vi "HV monitor.vi"() -> ()   [LabVIEW 2018]
uses:
  subvis/location cluster.ctl
  channel_cluster.ctl
  subvis/tabs.ctl
  subvis/crate.ctl
  subvis/card.ctl
  subvis/Channel Properties.ctl
  subvis/Group Properties.ctl
  subvis/channel.ctl
  subvis/Event Sources.ctl
  <vilib>/addons/zeromq/socket_type.ctl
  subvis/logs.ctl
  <vilib>/Utility/error.llb/DialogType.ctl
  history_array_type.ctl
  <vilib>/Utility/miscctls.llb/LVMinMaxIncTypeDef.ctl
  Tom Shaw/Lecroy Control/HV Documentation and Software for Testing/SubVIs/General_lecroy_command.ctl
  subvis/set location.ctl
  <vilib>/addons/zeromq/poll_type.ctl
  CAEN globals.vi
  <vilib>/Instr/_visa.llb/VISA Configure Serial Port (Instr).vi
  <vilib>/Utility/file.llb/Write Delimited Spreadsheet (string).vi
  subvis/bool to string small.vi
  <vilib>/Utility/file.llb/Read Delimited Spreadsheet (string).vi
  <vilib>/addons/zeromq/zmq_poll_scalar.vi
  <userlib>/_OpenG.lib/array/array.llb/Filter 1D Array with Scalar (I32)__ogtk.vi
  <userlib>/_OpenG.lib/array/array.llb/Delete Elements from 1D Array (I32)__ogtk.vi
  <userlib>/_OpenG.lib/array/array.llb/Remove Duplicates from 1D Array (I32)__ogtk.vi
  subvis/Timestamp String to LV Timestamp.vi
  subvis/buffer 2D array clust.vi
  subvis/buffer array clust.vi
  <vilib>/regexp/Match Regular Expression.xnode
  <vilib>/Utility/miscctls.llb/LVRowAndColumnTypeDef.ctl
  <vilib>/Utility/miscctls.llb/LVBoundsTypeDef.ctl
  <vilib>/addons/zeromq/zmq_context.lvclass
  <vilib>/addons/zeromq/zeromq.lvlib
  <vilib>/addons/zeromq/zmq_socket.lvclass
  <vilib>/platform/TimedLoop/XDataNode/XDataNode.xnode
  <vilib>/Platform/TimedLoop/XDataNode/nitl_modes.ctl
  <vilib>/Platform/TimedLoop/XDataNode/XDNodeRunTimeDep.lvlib
  <vilib>/Platform/TimedLoop/XDataNode/wakeup.ctl
  <vilib>/Platform/TimedLoop/XDataNode/timing_clust.ctl
panel:
  in  "Redundant bool":bool
  out "ZMQ_PMT_Err":string="\"%s\":\"%s\""
  out "slack":T1
  out "slack error":string
  in  "New Errors":string
  out "read error":cluster{"Crate":i32, "error out":errorcluster}
  in  "Reading LeCroy1 Page":bool
  in  "Reading LeCroy2 Page":bool
  in  "Update Plots & Alarms":T2
  in  "Do L2 Page Read":i32
  in  "Do L1 Page Read":i32
  in  "Read Crate Page":i32
  in  "Read Crate":i32
  in  "Do Caen Page Read":i32
  in  "Save PMT Voltage File":bool=TRUE
  out "Current ZMQ Log":path
  in  "Send ZMQ Reply":bool
  in  "Show hidden tabs":bool
  out "Status":string
  in  "get log file":bool=TRUE
  out "log file to get":string
  in  "Set Card.Channel":T3={" Card.Channel"=1.12, "Crate"=0} {"Card.Channel" format="%.2f"}
  in  "Handle ZMQ message":bool
  out "Selection Position":cluster{i32, i32}
  in  "Display String":string="Q"
  out "Time Element History.old":i32[][][](array[numeric])
  in  "Property":T4
  in  "Value":variant
  in  "Set channel property":bool
  out "bytes read Old":u32
  in  "Tab Control":T5
  in  "Shifter Notes":string
  out "Currents":cluster{dbl[], "TS History":dbl[]}[](graph)
  out "summary status":string
  out "Voltages":cluster{dbl[], "TS History":dbl[]}[](graph)
  in  "Clear Alarms":bool
  out "Read time (ms)":u32
  out "Key sent":string
  out "Screen Cluster":T6
  out "Display":string[][](table)
  out "lecroy2_hw_enable":bool
  out "lecroy1_hw_enable":bool
  out "caen_hw_enable":bool
  in  "Caen enable":bool
  in  "Lecroy 2 enable":bool
  in  "Lecroy 1 enable":bool
  in  "Show Group In Displayed Channels":bool
  in  "Add Group to Displayed Channels":bool
  in  "Restore PMT voltages":bool
  in  "Save PMT voltages":bool
  in  "Nominal PMT voltages":bool
  in  "Group":string(combo)="ACTIVE"
  in  "Set Group Property":bool
  in  "Value 2":dbl min=0.0 max=1.0 step=1.0 format="%1d"
  in  "Group Prop":T7 caption="Property"
  in  "Channel Array":T8[](array[typedef]) caption="Channel Name          ON    Status                                           Crate      Card      Chan       Vmon           Vset             Vfile               Imon            Imax              Timestamp                       Flag" {"Vfile (V)" format="%.1f V"; "Vswmax (V)" format="%#_g V"; "Iset (A)" format="%.2pA"; "Imon (A)" format="%.2pA"; "Vset (V)" format="%#_g V"; "Vmon (V)" format="%.1f V"}
  in  "Abort queued actions":bool
  in  "CAEN Vsel Buffer":bool=TRUE
  in  "re-read vfile voltages":bool
  in  "Channel Settings File":path=path "C:/Users/User/Documents/Logs/Channel_Settings.csv"
  in  "Ramp Voltages Slowly":bool
  in  "Start New Run":bool
  in  "Subrun":i32
  in  "Run":i32=1
  out "Current Channel Log":path
  out "Current Event Log":path
  in  "Start New Event Log":bool
  in  "Start New Channel Log":bool
  in  "Start New Error Log":bool
  in  "CAEN Serial Port":i32=6
  out "Current Error Log":path
  in  "Log Directory":path=path "C:/Users/User/Documents/Logs"
  in  "Log to File":bool=TRUE
  in  "Scan Rate (ms)":i32=1000
  in  "LeCroy 1 Serial Port":i32=5
  in  "LeCroy 2 Serial Port":i32=3
  in  "Slack port":u16=5995
  in  "CAEN Vsel Buffer Pin":u8=3 min=2 max=12 step=1
  in  "CAEN SW Enable Pin":u8=4 min=2 max=12 step=1
  in  "Arduino Serial Port":i32=9
  in  "ZMQ endpoint":string="tcp://*:5555"
  out "Crates":T9[](array[typedef]) caption="Crate Map"
  in  "Refresh Crate Map":bool
  out "Display array":string[][](array[string])
  in  "Crate":i32
  in  "Index":i32
  in  "Card":i32
  out "Current":T11(graph) caption="Current Graph"
  in  "History Length":i32=500
  out "Voltage":T11(graph) caption="Voltage Graph"
  in  "Channel":i32
  out "Error Timestamp":string
  out "Error Log":string[][](table)
  in  "Action log":string
  in  "error out":errorcluster
  out "Event Log":string[][](table)
  out "Alarm status":string
  in  "Send to Self":bool
  in  "Unsent Messages":string[](array[string])
  out "ZMQ Log":string[][](table)
  out "ZMQ message":string
  in  "ZMQ Reply":string[](array[string])
  out "Sending ZMQ":bool=TRUE
  in  "ZMQ Message":string[](array[string])=["{\"msg_id\":\"123\" , \"msg_type\":\"read\", \"msg_property\":\"vset\", \"2.4.2\":\"anything\"}", "{\"msg_id\":\"123\" , \"msg_type\":\"write\", \"msg_property\":\"vset\", \"2.4.2\":\"-1500\"}"]
  in  "Manual ZMQ Write":bool
  out "Screencap Timestamp":string
  out "Alarm Screencap":string
  out "Read buffer LeCroy 1":string
  out "Read buffer LeCroy 2":string
  out "Read buffer CAEN":string
  in  "Read":bool
  in  "'\\' codes display":bool
  in  "Line Wrapping":bool=TRUE
  in  "Write buffer":string caption="Write buffer ( '\\' code format)"
  in  "Write":bool
  in  "Reading page label":string="Reading page ..."
  in  "Config pg Crate":i32 caption="Crate" min=0 max=2 step=1
  in  "delay (ms)":u32=700 max=600000 step=1
  in  "stop":bool
  out "Reading page":bool
  in  "scan":bool=TRUE
  in  "Lock Page":bool
  in  "Kill All":bool
  out "Writing...":bool
  out "Reading...":bool
  in  "Timestamp":string
  in  "Status message":string
  out "hb":bool
  out "bytes read":cluster{dbl, "element":i32}(graph)
  # "N.B. demonstration messages: these are valid messages\nClear the array and write your own before sending!!!"
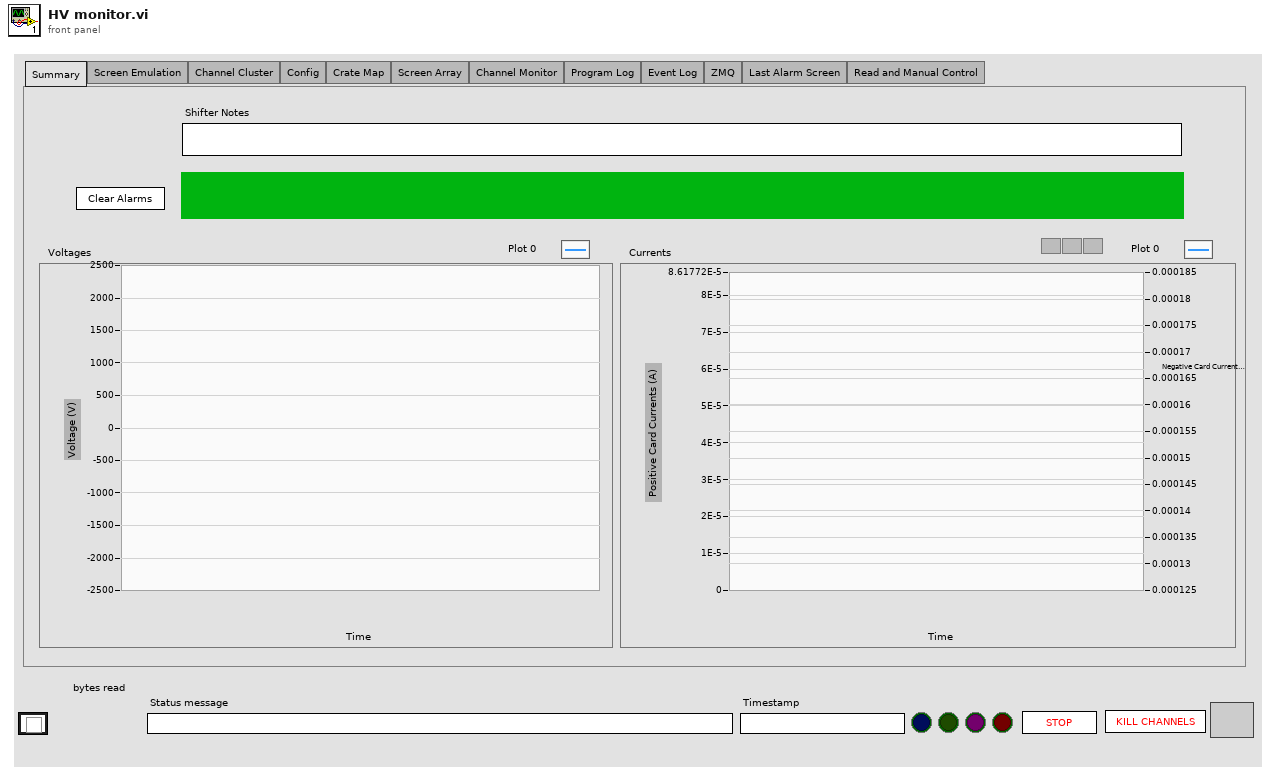
[diagram p1: front panel]
types:
  T1 = typedef "Semaphore RefNum" = refnum<k1>
  T2 = cluster{"Start Index":i32, "Num Channels Read":i32}
  T3 = typedef "channel.ctl" = cluster{" Card.Channel":dbl, "Crate":i32}
  T4 = typedef "Channel Properties.ctl" = enum16{"Name", "Vset", "Vfile", "Vswmax", "Iset", "Enable", "Flag", "Vbackup"}
  T5 = typedef "tabs.ctl" = enum32{"Summary", "Screen Emulation", "Channel Cluster", "Config", "Crate Map", "Screen Array", "Channel Monitor", "Program Log", "Event Log", "ZMQ", "Last Alarm Screen", "Read and Manual Control"}
  T6 = typedef "location cluster.ctl" = cluster{"Column":i32, "Card Type":string, "Channel":i32, "Card":i32, "Default response":string, "Entering":string, "Entering state":bool, "subpage":i32, "page":i32, "Crate":i32, "Screen":string, "Group":string, "Global HV Enable":bool, "Vsel_buffer":bool, "Vdisp_buffer":bool}
  T7 = typedef "Group Properties.ctl" = enum16{"Enable", "Vset", "Imax", "Vswmax", "Trip Time"}
  T8 = typedef "channel_cluster.ctl" = cluster{"Channel Name":string, "Crate":i32, "Card Type":string, "Card":i32, "Channel":i32, "Status Icon":picture, "Vmon (V)":dbl, "Vset (V)":dbl, "Imon (A)":dbl, "Iset (A)":dbl, "Timestamp":string, "ON/OFF":bool, "Status":string, "Vswmax (V)":dbl, "Flag":bool, "Vfile (V)":dbl, "Error Logged":bool[], "enable_file":bool}
  T9 = typedef "crate.ctl" = cluster{"CAENet Address":i32, "Crate Model":string, "Firmware Version":string, "Crate Map":T10[], "Total Channels":i32}
  T10 = typedef "card.ctl" = cluster{"Slot Number":i32, "Card Model":string, "Num Channels":i32, "Polarity":string, "Vmax":dbl, "Imax":dbl, "Revision":string}
  T11 = cluster{"Timestamp History":dbl[], "Vmon Hist":dbl[]}[]
  T12 = typedef "LVBoundsTypeDef.ctl" = cluster{"Width":u32, "Height":u32}
  T13 = typedef "LVRowAndColumnTypeDef.ctl" = cluster{"Row":i32, "Column":i32}
  T14 = cluster{"Channel Name":string, "Crate":i32, "Card Type":string, "Card":i32, "Channel":i32, "Status Icon":picture, "Vmon (V)":dbl, "Vset (V)":dbl, "Imon (mA)":dbl, "Iset (mA)":dbl, "Timestamp":string, "ON/OFF":bool, "Status":string}
  T15 = enum32{"Invalid", "Standard", "Closed", "Hidden", "Minimized", "Maximized"}
  T16 = typedef "Event Sources.ctl" = enum16{"ZMQ", "INTERNAL", "Check_Errors", "Send_ZMQ_Reply", "Save_PMT_Voltages", "Set_Ramp_Voltage", "Restore PMT Voltages"}
  T17 = typedef "zeromq.lvlib/socket_type.ctl" = enum8{"ZMQ_PAIR", "ZMQ_PUB", "ZMQ_SUB", "ZMQ_REQ", "ZMQ_REP", "ZMQ_DEALER", "ZMQ_ROUTER", "ZMQ_PULL", "ZMQ_PUSH", "ZMQ_XPUB", "ZMQ_XSUB"}
  T18 = cluster{"Group Name":string, "Channels in Group":T3[]}
  T19 = cluster{"Group Name":string, "Channels in Group":T3[]}[]
  T20 = typedef "logs.ctl" = enum16{"Event", "ZMQ", "Channel", "Program"}
  T21 = cluster{"seconds since 1Jan1904":timestamp, "element":cluster{"Source":T16, "Command":string}}[]
  T22 = typedef "LVMinMaxIncTypeDef.ctl" = cluster{"Minimum":dbl, "Maximum":dbl, "Increment":dbl}
  T23 = typedef "General_lecroy_command.ctl" = string
  T24 = typedef "set location.ctl" = cluster{"set index":i32, "set Screen":string, "set subpage":i32, "set column":i32, "Group":string, "Crate":i32}
  T25 = typedef "zeromq.lvlib/poll_type.ctl" = enum16{"None", "In", "Out", "In/Out"}
  T26 = cluster{"Group Value":timestamp, "element":cluster{"Source":T16, "Command":string}}
  T27 = cluster{"Group Value":timestamp, "element":cluster{"Source":T16, "Command":string}}[]
  T28 = typedef "eventvkey.ctl" = enum16{"ASCII", "Enter", "Return", "Shift", "Ctrl", "Alt", "Cmd", "Opt", "Caps", "NumLock", "Clear", "Break", "Up", "Down", "Left", "Right", "Insert", "Delete", "Home", "End", "PageUp", "PageDown", "Escape", "Help", "Pause", "ScrollLock", "F1", "F2", "F3", "F4", "F5", "F6", "F7", "F8", "F9", "F10", "F11", "F12", "F13", "F14", "F15", "F16", "F17", "F18", "F19", "F20", "F21", "F22", "F23", "F24", "Play", "VolumeUp", "VolumeDown", "Mute", "Two Byte Char"}
  T29 = cluster{"seconds since 1Jan1904":timestamp, "element":cluster{"Source":T16, "Command":string}}
  T30 = typedef "DialogType.ctl" = u16
  T31 = typedef "history_array_type.ctl" = enum16{"Vmon", "Vset", "Imon", "Iset", "TimeStamp"}
  T32 = typedef "XDNodeRunTimeDep.lvlib/timing_clust.ctl" = cluster{"Expected End [f-1]":u64, "Actual End [f-1]":u64, "Finished Late? [f-1]":bool, "Expected End [i-1]":u64, "Actual End [i-1]":u64, "Finished Late? [i-1]":bool, "Expected Start [i]":u64, "Actual Start [i]":u64, "Expected Start [f]":u64, "Actual Start [f]":u64, "Source Name":string, "Structure Name":string, "Period":i64, "Deadline":i64, "Offset":i64, "Start":i64, "Priority":i32, "Timeout":i32, "Mode":T33, "Wakeup Reason":T34, "Error":errorcluster, "Source Type":string, "Secondary Source Type":string, "Global End Time":u64, "Global Start Time":u64, "Frame Duration":u64, "Iteration Duration":u64, "Assigned CPU":i32, "I/O Scan Engine Mode":u32}
  T33 = typedef "XDNodeRunTimeDep.lvlib/nitl_modes.ctl" = enum32{"No Change", "Process missed periods, maintain original phase", "Discard missed periods, maintain original phase", "Process missed periods, ignore original phase", "Discard missed periods, ignore original phase"}
  T34 = typedef "XDNodeRunTimeDep.lvlib/wakeup.ctl" = enum32{"Normal", "Aborted", "Asynchronous wakeup", "Timing source error", "Timed loop error", "Timeout"}
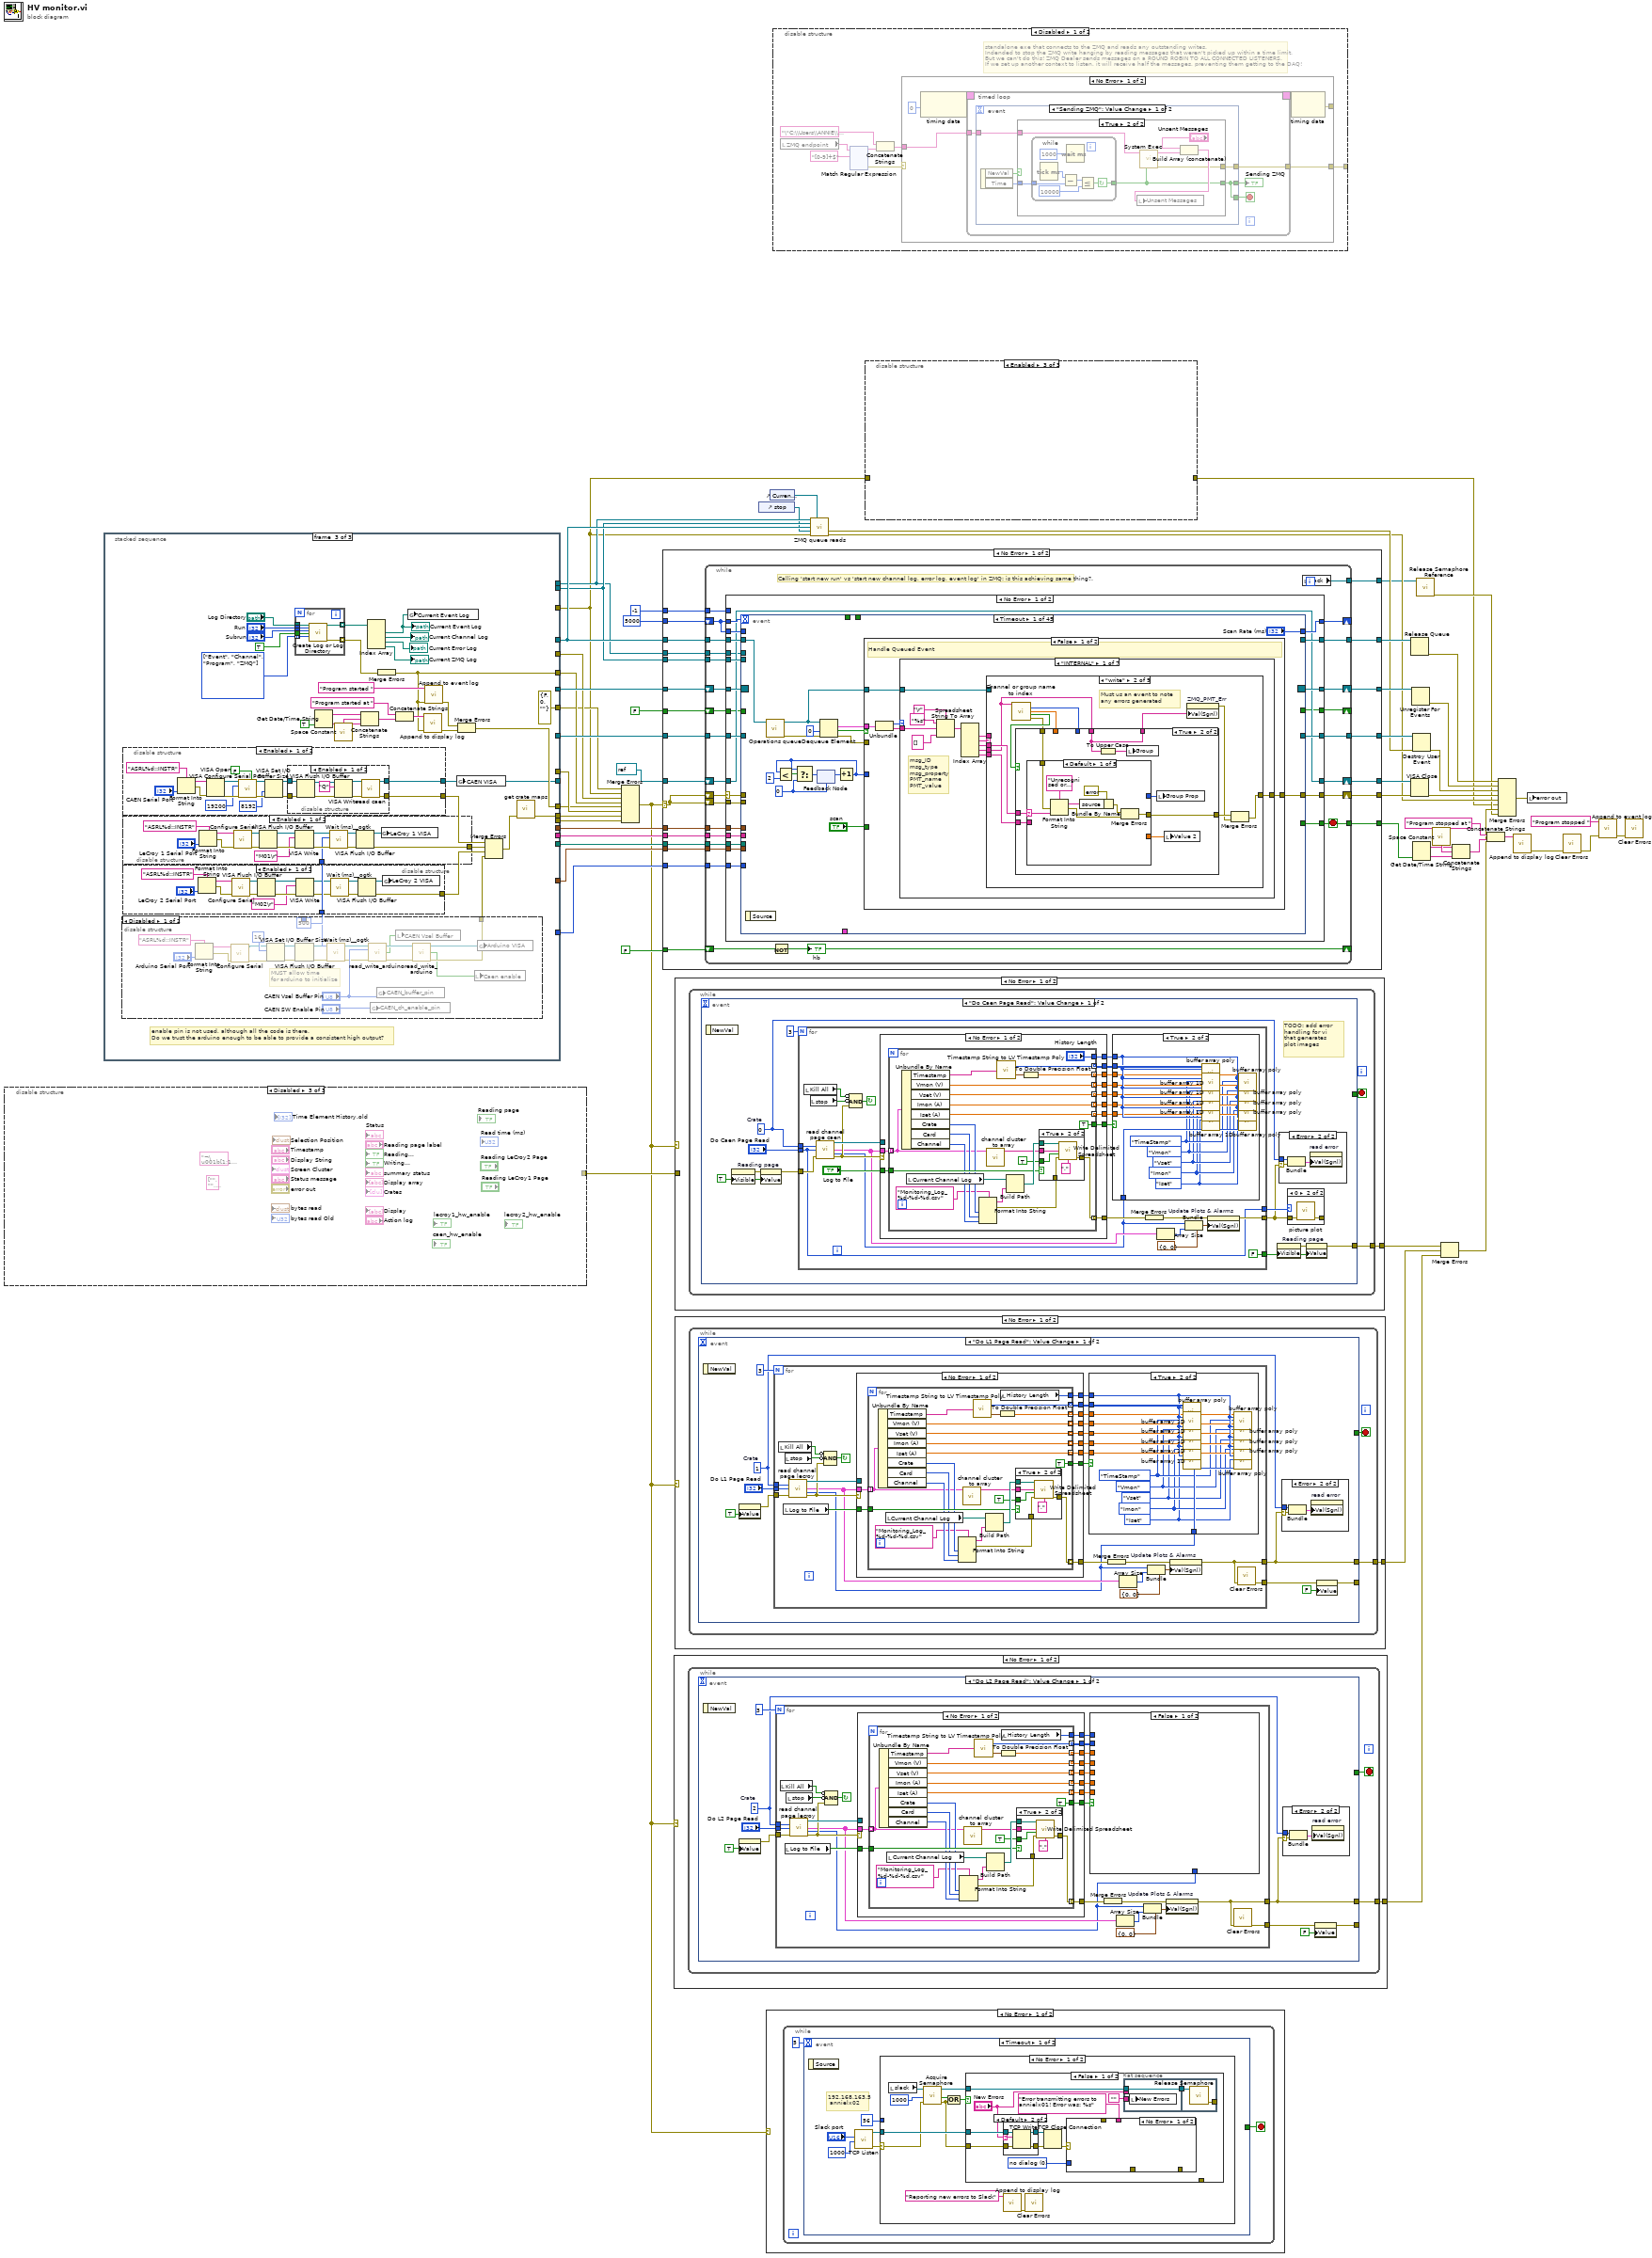
[diagram p0: block diagram]
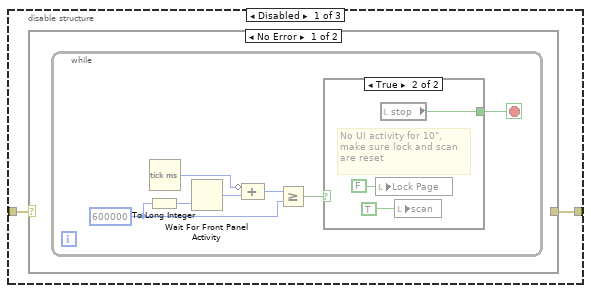
[diagram p2: hidden frame]
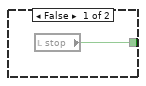
[diagram p3: hidden frame]
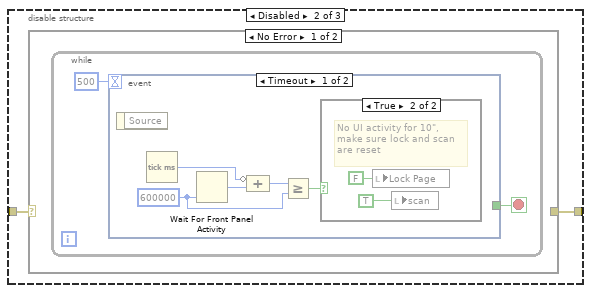
[diagram p5: hidden frame]
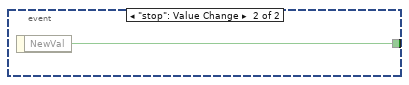
[diagram p7: hidden frame]
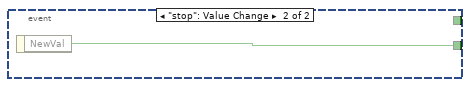
[diagram p10: hidden frame]
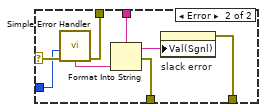
[diagram p13: hidden frame]
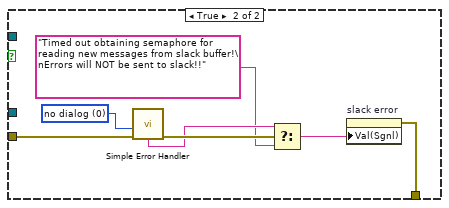
[diagram p15: hidden frame]
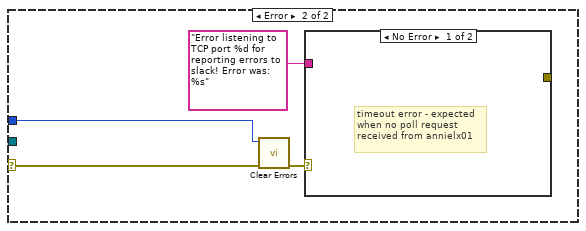
[diagram p16: hidden frame]
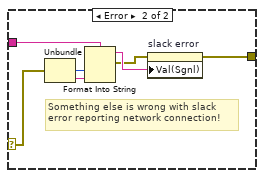
[diagram p17: hidden frame]
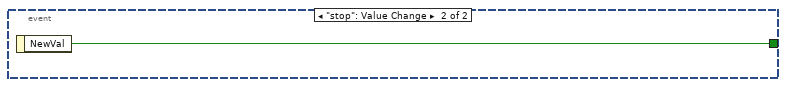
[diagram p18: hidden frame]
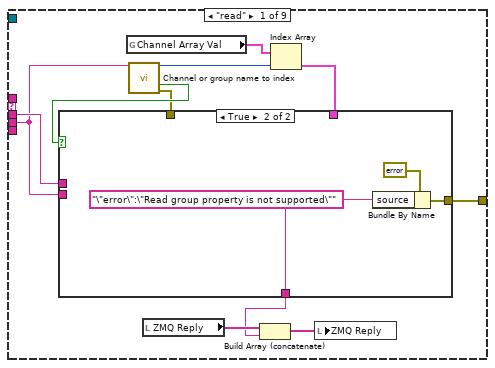
[diagram p20: hidden frame]
diagram:
  n1 = disable-structure shown="Disabled" {
    disable-tunnel: [w59 _ _] -> w11
    frame Disabled {
      w58 = 140 ("number")
      n2 = disable-structure shown="Disabled" {
        disable-tunnel: [w68 _] -> w65
        frame Disabled {
          n3 = property on="Display" class="Tbl (strict)"("Number of Columns"=u32 75, "Number of Rows"=u32 22 ("Number of Columns")) -> (error out=w68:errorcluster)  [unwired: 2 in, 1 out]
        }
        frame Enabled {
        }
      }
      n4 = property on="Display" class="Tbl (strict)" props=["Number of Columns", "Number of Rows"](error in=w65) -> ("Number of Rows"=w62:u32)  [unwired: 1 in, 3 out]
      n5 = To Long Integer(number=w62) -> (32bit integer=w63:i32)
      n6 = To Long Integer(number=w58) -> (32bit integer=w64:i32)
      n7 = disable-structure shown="Disabled" {
        disable-tunnel: w64 -> [w72 _]
        disable-tunnel: w63 -> [w71 _]
        disable-tunnel: [w70 w82] -> w61
        disable-tunnel: T12 {"Width"=13, "Height"=18} ("Active Cell:Cell Size") -> [w69 w82]
        frame Disabled {
          n8 = for {
            N: w72 -> [_]
            tunnel: w71 -> [w76]
            tunnel: [w74] -> w70
            tunnel: w69 -> [w73]
            i -> [w75]
            n9 = for {
              N: w76 -> [_]
              tunnel: w75 -> [w78]
              tunnel: [w77] -> w74
              tunnel: w73 -> [w77]
              i -> [w79]
              n10 = Bundle By Name(cluster=T13 {"Row"=0, "Column"=0} ("Active Cell:Active Cell"), "Row"=w79, "Column"=w78) -> (w80:T13)
              n11 = property on="Display" class="Tbl (strict)"("Active Cell"=w80, "Cell Size"=w77) -> ()  [unwired: 2 in, 2 out]
            }
          }
        }
        frame Enabled {
        }
      }
      n12 = for {
        N: w58 -> [_]
        tunnel: w61 -> [w84]
        tunnel: [w83] -> w59
        i -> [w86]
        n13 = Bundle By Name(cluster=T13 {"Row"=0, "Column"=0} ("Active Cell:Active Cell"), "Row"=0, "Column"=w86) -> (w87:T13)
        n14 = property on="Display" class="Tbl (strict)"("Active Cell"=w87, "Cell Size"=w84) -> (error out=w83:errorcluster)  [unwired: 2 in, 1 out]
      }
    }
    frame Enabled {
      (unwired) T14 {"Channel Name"="", "Crate"=0, "Card Type"="", "Card"=0, "Channel"=0, "Status Icon"=bytes[0], "Vmon (V)"=0.0, "Vset (V)"=0.0, "Imon (mA)"=0.0, "Iset (mA)"=0.0, "Timestamp"="", "ON/OFF"=FALSE, "Status"=""} ("Channel cluster")
      # "Channel, HVmax, Vmon, Imon, V*set, I*set, Pw, Status, Ch#\nChannel, SVmax, Rup, Rdwn, Trip, TripEx, PrOn, PrOff, Pon, Pdwn, Pswd, On/Off, Ch#"
      # "NEGAIVE: xxx.xxx mA only on chx.24\nreading also in mA\n\nPOSITIVE: xxxx.xx uA on all channels"
      # "0.* Channel name\n1.   Crate\n2.   Card Type\n3.   Card\n4.   Channel\n5.* Status Icon\n6.   Vmon\n7.* Vset\n8.   Imon\n9.* Iset\n10. Timestamp\n11.*On/Off"
      # "Display\nSet Protection (subpages todo)\nMain Menu\nLogo\nCrate Map\nKill Confirm\nConfigure Alarms\nFormat EEPROM\nUpgrade Firmware\nPage not recognised!"
    }
    frame Disabled {
      (unwired) "¬\u001b[1;1H¬\u001b[2J¬\u001b[4;10H¬\u001b[1mC.A.E.N.       SY527        V3.18¬\u001b[0m¬\u001b[4;62H¬\u001b[1mCrate 01¬\u001b[0m¬\u001b[9;7H¬\u001b[1mM A I N   M E N U¬\u001b[0m¬\u001b[11;1H      ¬\u001b[1mD¬\u001b[0misplay             Display/Modify channels\r\n      ¬\u001b[1mP¬\u001b[0mrotections         Set/Reset password\r\n      ¬\u001b[1mC¬\u001b[0mrate               Connect a new crate\r\n      ¬\u001b[1mM¬\u001b[0map                 Crate map\r\n      ¬\u001b[1mK¬\u001b[0mill                Kill all channels\r\n      ¬\u001b[1mA¬\u001b[0mlarms              Reset alarms\r\n      ¬\u001b[1mQ¬\u001b[0muit                Abandon program\r\n¬\u001b[0m¬\u001b[23;7HSelect item\r\n¬\u001b[23;1H¬\u001b[KEnter the crate number to be connected. [01]: " ("stripped output")
      (unwired) string[][] [["", "", "", "", "", "", "", "", "", "", "", "", ""], ["", "C.A.E.N.", "SY527", "V3.18", "A734 ", "", "", "", "", "", "", "", ""], ["", "GROUP00", "Ch_En is: On", "V0-SEL", "I0-SEL", "Crate 01", "Page 0 ", "", "", "", "", "", ""], ["", "", "", "", "", "", "", "", "", "", "", "", ""], ["Channel", "SVmax", "Rup", "Rdwn", "Trip", "TripEx", "PrOn", "PrOff", "Pon", "Pdwn", "Pswd", "On/Off", "Ch#"], ["KLn_1", "2200", "100", "100", "600.0", "--", "01", "01", "Off", "Kill", "Req", "En", "0.00"], ["KLn_2", "2200", "100", "100", "011.0", "--", "01", "01", "Off", "Kill", "", "", "0.01"], ["KLn_3", "2200", "100", "100", "010.0", "--", "01", "01", "Off", "Kill", "", "", "0.02"], ["KLn_4", "2200", "100", "100", "010.0", "--", "01", "01", "Off", "Kill", "", "", "0.03"], ["KLn_5", "2200", "100", "100", "010.0", "--", "01", "01", "Off", "Kill", "", "", "0.04"], ["KLn_6", "2200", "100", "100", "010.0", "--", "01", "01", "Off", "Kill", "", "", "0.05"], ["KLn_7", "2200", "100", "100", "010.0", "--", "01", "01", "Off", "Kill", "", "", "0.06"], ["KLn_8", "2200", "100", "100", "010.0", "--", "01", "01", "Off", "Kill", "", "", "0.07"], ["KLn_9", "2200", "100", "100", "010.0", "--", "01", "01", "Off", "Kill", "", "", "0.08"], ["KLn_10", "2200", "100", "100", "010.0", "--", "01", "01", "Off", "Kill", "", "", "0.09"], ["KLn_11", "2200", "100", "100", "010.0", "--", "01", "01", "Off", "Kill", "", "", "0.10"], ["KLn_12", "2200", "100", "100", "010.0", "--", "01", "01", "Off", "Kill", "", "", "0.11"], ["KLn_13", "2200", "100", "100", "010.0", "--", "01", "01", "Off", "Kill", "", "", "0.12"], ["KLn_14", "2200", "100", "100", "010.0", "--", "01", "01", "Off", "Kill", "", "", "0.13"], ["KLn_15", "2200", "100", "100", "110.0", "--", "01", "01", "Off", "Kill", "", "", "0.14"], ["KLn_16", "2200", "100", "100", "010.0", "--", "01", "01", "Off", "Kill", "", "", "0.15"], ["", "", "", "", "", "", "", "", "", "", "", "", ""], ["", "", "", "", "", "", "", "", "", "", "", "", ""], ["", "", "", "", "", "", "", "", "", "", "", "", ""], [" Quit Edit Change Update Next Prev More Switch", "", "", "", "", "", "", "", "", "", "", "", ""]] ("Display array 2")
    }
  }
  n15 = stacked-sequence {
    tunnel: [_ _ w191] -> w46
    tunnel: [_ w144 _] -> w49
    tunnel: [_ w170 _] -> w48
    tunnel: [_ w165 _] -> w47
    tunnel: [_ w169 _] -> w9
    tunnel: [_ w168 _] -> w19
    tunnel: [_ w167 _] -> w2
    tunnel: [_ _ w189] -> _
    tunnel: [w95 _ _] -> w17
    tunnel: [w93 _ _] -> w40
    tunnel: [_ _ w196] -> w39
    tunnel: [_ w161 _] -> w37
    tunnel: [_ w160 _] -> w38
    tunnel: [_ _ w197] -> w24
    tunnel: [w97 _ _] -> w23
    tunnel: [_ w151 _] -> w22
    tunnel: [_ w150 _] -> w21
    tunnel: [_ _ errorcluster {"status"=FALSE, "code"=0, "source"=""} ("error IO")] -> w20
    tunnel: [w109 _ _] -> w8
    frame #0 {
      w119 = "Everything is awesome" ("Alarm String")
      w120 = FALSE ("Append if exists?")
      # "This list MUST match the\ngroups defined on the CAEN\nand no additional groups\nshould be defined in the \nchannel settings file"
      # "num active\ncaen pages"
      n16 = invoke on="Action log" class="Str" method="Reinit To Default"() -> ()  [unwired: 3 in, 3 out]
      n17 = invoke on="Set Group Property" class="Bool (strict)" method="Reinit To Default"() -> ()  [unwired: 3 in, 3 out]
      n18 = invoke on="Channel Array" class="Arr (strict)" method="Reinit To Default"() -> ()  [unwired: 3 in, 3 out]
      n19 = invoke on="re-read vfile voltages" class="Bool" method="Reinit To Default"() -> ()  [unwired: 3 in, 3 out]
      n20 = invoke on="stop" class="Bool (strict)" method="Reinit To Default"() -> ()  [unwired: 3 in, 3 out]
      n21 = property on="summary status" class="Str"("Value"=w119, "Text.BGColor"=u32 46096, "Blinking"=w120) -> (error out=w118:errorcluster)  [unwired: 2 in, 1 out]
      n22 = invoke on="Writing..." class="Bool (strict)" method="Reinit To Default"() -> ()  [unwired: 3 in, 3 out]
      n23 = invoke on="New Errors" class="Str" method="Reinit To Default"() -> ()  [unwired: 3 in, 3 out]
      n24 = invoke on="Reading LeCroy1 Page" class="Bool (strict)" method="Reinit To Default"() -> ()  [unwired: 3 in, 3 out]
      n25 = invoke on="Reading LeCroy2 Page" class="Bool (strict)" method="Reinit To Default"() -> ()  [unwired: 3 in, 3 out]
      n26 = invoke on="Reading page" class="Bool (strict)" method="Reinit To Default"() -> ()  [unwired: 3 in, 3 out]
      n27 = call "load channel file.vi"("Group Names"=string[] ["GROUP00", "ACTIVE", "CARD0", "CARD1", "CARD2", "CARD3", "AGROUP", "CARD4", "MRD", "FACC", "TANK", "CAEN", "LeCroy1", "LeCroy2", "SPARE", "Broken"], "Channel List"="Channel Settings File") -> ("error out"=w98:errorcluster, "ACTIVE"=w106:T18, "GROUP00"=w108:T18, "Groups"=w100:T19)  [unwired: 5 in, 1 out]
      n28 = Read from Text File(file (use dialog)=path "C:/Users/User/Documents/Logs/Shifter_Notes.txt") -> (refnum out=w115:refnum<file>, text=w112:string, error out=w114:errorcluster)  [unwired: 3 in, 1 out]
      n29 = property on="Status message" class="Str"(error in=w118, "Value"=w119, "Blinking"=w120) -> ()  [unwired: 1 in, 2 out]
      n30 = Close File(refnum=w115, error in=w114) -> (error out=w113:errorcluster)  [unwired: 1 out]
      n31 = local write "Shifter Notes"(w112) -> ()
      n32 = for {
        tunnel: w100 -> [w131] mode=indexing
        tunnel: [w130] -> w99 mode=indexing
        n33 = Unbundle By Name(w131) -> ("Group Name"=w130:string)
      }
      n34 = global write "CAEN globals.vi" "Groups"(w100) -> ()
      n35 = Unbundle By Name(w106) -> ("Channels in Group"=w93:T3[])
      n36 = Unbundle By Name(w108) -> ("Channels in Group"=w95:T3[])
      n37 = call <vilib>:"Clear Errors.vi"("error in (no error)"=w113) -> ()  [unwired: 5 in, 2 out]
      n38 = property on="Group" class="CmbBox"(error in=w98, "Strings[]"=w99) -> (error out=w97:errorcluster)  [unwired: 1 in, 1 out]
      n39 = for {
        tunnel: w93 -> [w137] mode=indexing
        shift-right: [w134] -> w110
        shift-left: 0 ("Crate") -> [w132]
        n40 = Unbundle By Name(w137) -> ("Crate"=w136:i32)
        n41 = Increment(x=w132) -> (x+1=w133:i32)
        n42 = Not Equal To 0?(x=w136) -> (x != 0?=w135:bool)
        n43 = Select(t=w132, s=w135, f=w133) -> (s? t:f=w134:i32)
      }
      n44 = for {
        tunnel: w93 -> [w139] mode=indexing
        tunnel: w95 -> [w140]
        tunnel: [w138] -> w117 mode=indexing
        n45 = Search 1D Array(1D array=w140, element=w139) -> (index of element=w138:i32)  [unwired: 1 in]
      }
      n46 = control-ref of="CAEN Vsel Buffer"() -> (w89:refnum<vi>)
      n47 = control-ref of="Caen enable"() -> (w104:refnum<vi>)
      n48 = control-ref of="Lecroy 1 enable"() -> (w103:refnum<vi>)
      n49 = control-ref of="Lecroy 2 enable"() -> (w102:refnum<vi>)
      n50 = control-ref of="caen_hw_enable"() -> (w92:refnum<vi>)
      n51 = control-ref of="lecroy1_hw_enable"() -> (w91:refnum<vi>)
      n52 = control-ref of="lecroy2_hw_enable"() -> (w90:refnum<vi>)
      n53 = control-ref of="Writing..."() -> (w123:refnum<vi>)
      n54 = control-ref of="Reading..."() -> (w124:refnum<vi>)
      n55 = control-ref of="Screen Cluster"() -> (w101:refnum<vi>)
      n56 = control-ref of="This VI"() -> (w129:refnum<vi>)
      n57 = control-ref of="Display String"() -> (w126:refnum<vi>)
      n58 = control-ref of="Action log"() -> (w125:refnum<vi>)
      n59 = control-ref of="Channel Array"() -> (w96:refnum<vi>)
      n60 = control-ref of="Crates"() -> (w111:refnum<vi>)
      n61 = control-ref of="Display"() -> (w127:refnum<vi>)
      n62 = control-ref of="Display array"() -> (w128:refnum<vi>)
      n63 = control-ref of="Event Log"() -> (w122:refnum<vi>)
      n64 = global write "CAEN globals.vi" "Main VI"(w129) -> ()
      n65 = global write "CAEN globals.vi" "Channel Array"(w96) -> ()
      n66 = global write "CAEN globals.vi" "Crate Maps"(w111) -> ()
      n67 = global write "CAEN globals.vi" "Display"(w127) -> ()
      n68 = global write "CAEN globals.vi" "Display array"(w128) -> ()
      n69 = global write "CAEN globals.vi" "Location Cluster"(w101) -> ()
      n70 = global write "CAEN globals.vi" "Display string"(w126) -> ()
      n71 = global write "CAEN globals.vi" "Display Log"(w125) -> ()
      n72 = global write "CAEN globals.vi" "Event Log Indicator"(w122) -> ()
      n73 = global write "CAEN globals.vi" "Reading..."(w124) -> ()
      n74 = global write "CAEN globals.vi" "Writing..."(w123) -> ()
      n75 = global write "CAEN globals.vi" "CAEN HV enable"(w104) -> ()
      n76 = global write "CAEN globals.vi" "Lecroy 1 HV enable"(w103) -> ()
      n77 = global write "CAEN globals.vi" "Lecroy 2 HV enable"(w102) -> ()
      n78 = global write "CAEN globals.vi" "caen_hw_enable"(w92) -> ()
      n79 = global write "CAEN globals.vi" "lecroy1_hw_enable"(w91) -> ()
      n80 = global write "CAEN globals.vi" "lecroy2_hw_enable"(w90) -> ()
      n81 = global write "CAEN globals.vi" "CAEN Vsel Buffer"(w89) -> ()
      n82 = global write "CAEN globals.vi" "Visible Channels"(w117) -> ()
      n83 = global write "CAEN globals.vi" "Indices of ACTIVE"(w117) -> ()
      n84 = expression code="ceil(x/16)"(w110) -> (w109:i32)
    }
    frame #1 {
      w150 = "Run: %d Subrun: %d" ("ZMQ endpoint")
      n85 = control-ref of="This VI"() -> (w149:refnum<vi>)
      n86 = invoke class="VI" method="FP.Open"(reference=w149, "Activate"=TRUE ("Activate?"), "State"=T15."Standard") -> (error out=w143:errorcluster)  [unwired: 2 in, 4 out]
      n87 = disable-structure shown="Enabled" {
        disable-tunnel: [w180 _] -> w167
        disable-tunnel: [w177 _] -> w168
        disable-tunnel: [w182 _] -> w169
        frame Enabled {
          n88 = call <vilib>:"zmq_ctx_create.vi"() -> ("error out"=w185:errorcluster, "context out"=w186:refnum<class "zmq_context.lvclass">)  [unwired: 4 in]
          n89 = call <vilib>:"zmq_socket.vi"("error in"=w185, "linger (ms)"=100, "socket type"=socket_type."ZMQ_DEALER", "context in"=w186) -> ("error out"=w183:errorcluster, "socket out"=w178:refnum<class "zmq_socket.lvclass">, "context out"=w182:refnum<class "zmq_context.lvclass">)  [unwired: 1 in]
          n90 = call <vilib>:"zmq_bind.vi"("error in"=w183, "endpoint"="ZMQ endpoint", "socket in"=w178) -> ("error out"=w180:errorcluster, "socket out"=w177:refnum<class "zmq_socket.lvclass">)  [unwired: 1 in]
        }
        frame Disabled {
        }
      }
      n91 = Equal?(x=tabs."Screen Emulation" ("Tab Control"), y="Tab Control") -> (x = y?=w173:bool)
      n92 = control-ref of="This VI"() -> (w171:refnum<vi>)
      n93 = Select(t=w171, s=w173, f=refnum<vi> refnum ("vi reference")) -> (s? t:f=w175:refnum<vi>)
      n94 = Create User Event(user event datatype="" ("ZMQ endpoint")) -> (user event=w165:refnum<user-event>, error out=w176:errorcluster)  [unwired: 1 in]
      n95 = register-events(error in=w176, w175, w165) -> (reference out=w170:refnum<event-registration>, error out=w145:errorcluster)  [unwired: 1 in]
      n96 = Read from Text File(file (use dialog)=path "C:/Users/User/Documents/Logs/CurrentRun.txt" ("file path (dialog if empty)")) -> (refnum out=w154:refnum<file>, text=w157:string, error out=w153:errorcluster)  [unwired: 3 in, 1 out]
      n97 = call <vilib>:"Obtain Semaphore Reference.vi"() -> ("error out"=w141:errorcluster, "semaphore"=→"slack":T1)  [unwired: 5 in, 1 out]
      n98 = Close File(refnum=w154, error in=w153) -> (path=w151:path, error out=w152:errorcluster)
      n99 = Obtain Queue(element data type=cluster{"Source":T16, "Command":string} {"Source"=enum."ZMQ", "Command"=""} ("element")) -> (queue out=w163:refnum<queue>, error out=w162:errorcluster)  [unwired: 4 in, 1 out]
      n100 = Scan From String(format string=w150, input string=w157, error in=w152) -> (error out=w146:errorcluster, output 1=w156:i32, output 2=w155:i32)  [unwired: 3 in, 2 out]
      n101 = Flush Queue(queue=w163, error in (no error)=w162) -> (queue out=w161:refnum<queue>, error out=w160:errorcluster)  [unwired: 1 out]
      n102 = local write "Run"(w156) -> ()
      n103 = local write "Subrun"(w155) -> ()
      n104 = Merge Errors(w143, w145, w146, w141) -> (w144:errorcluster)
    }
    frame #2 {
      w199 = T20[] [enum."Event", enum."Channel", enum."Program", enum."ZMQ"] items=["Event", "ZMQ", "Channel", "Program"]
      # "enable pin is not used, although all the code is there.\nDo we trust the arduino enough to be able to provide a consistent high output?"
      n105 = disable-structure shown="Disabled" {
        disable-tunnel: [w229 _] -> w188
        disable-tunnel: [w221 _] -> w187
        frame Disabled {
          w229 = u32 500 ("milliseconds to wait")
          # "MUST allow time\nfor arduino to initialize"
          n106 = Format Into String(format string="ASRL%d::INSTR" ("write buffer"), "Arduino Serial Port") -> (resulting string=w233:string, error out=w234:errorcluster)  [unwired: 2 in]
          n107 = call "Configure Serial.vi"("error in"=w234, "Resource Name"=w233) -> ("error out"=w231:errorcluster, "VISA out"=w232:refnum<visa-resource-name>)  [unwired: 8 in]
          n108 = VISA Set I/O Buffer Size(VISA resource name=w232, mask (16)=u16 16 ("I/O Receive\nBuffer mask"), error in (no error)=w231) -> (VISA resource name out=w238:refnum<visa-resource-name>, error out=w237:errorcluster)  [unwired: 1 in]
          n109 = VISA Flush I/O Buffer(VISA resource name=w238, error in (no error)=w237) -> (VISA resource name out=w228:refnum<visa-resource-name>, error out=w230:errorcluster)  [unwired: 1 in]
          n110 = call <userlib>:"Wait (ms)__ogtk.vi"("error in (no error)"=w230, "milliseconds to wait"=w229) -> ("error out"=w225:errorcluster)  [unwired: 8 in, 1 out]
          n111 = call "read_write_arduino.vi"("VISA in"=w228, "Pin Num"="CAEN Vsel Buffer Pin", "error in"=w225) -> ("VISA out"=w223:refnum<visa-resource-name>, "State"=w219:bool, "error out"=w224:errorcluster)  [unwired: 9 in, 1 out]
          n112 = global write "CAEN globals.vi" "CAEN_ch_enable_pin"("CAEN SW Enable Pin") -> ()
          n113 = global write "CAEN globals.vi" "CAEN_buffer_pin"("CAEN Vsel Buffer Pin") -> ()
          n114 = local write "CAEN Vsel Buffer"(w219) -> ()
          n115 = call "read_write_arduino.vi"("VISA in"=w223, "error in"=w224) -> ("VISA out"=w222:refnum<visa-resource-name>, "State"=w220:bool, "error out"=w221:errorcluster)  [unwired: 10 in, 1 out]
          n116 = local write "Caen enable"(w220) -> ()
          n117 = global write "CAEN globals.vi" "Arduino VISA"(w222) -> ()
        }
        frame Enabled {
        }
      }
      n118 = disable-structure shown="Enabled" {
        disable-tunnel: [w283 _] -> w189
        disable-tunnel: [w282 _] -> w195
        frame Enabled {
          n119 = Format Into String(format string="ASRL%d::INSTR" ("write buffer"), "CAEN Serial Port") -> (resulting string=w284:string, error out=w287:errorcluster)  [unwired: 2 in]
          n120 = VISA Open(error in (no error)=w287, VISA resource name=w284) -> (VISA resource name=w291:refnum<visa-resource-name>, error out=w290:errorcluster)  [unwired: 3 in]
          n121 = call-poly "VISA Configure Serial Port"("VISA resource name"=w291, "Enable Termination\nChar (T)"=FALSE ("Enable Termination\nChar (T)"), "baud rate (9600)"=u32 19200, "error in (no error)"=w290) -> ("VISA resource name out"=w281:refnum<visa-resource-name>, "error out"=w280:errorcluster)  [unwired: 10 in]
          n122 = VISA Set I/O Buffer Size(VISA resource name=w281, size (4096)=u32 8192 ("baud rate (9600)"), error in (no error)=w280) -> (VISA resource name out=w279:refnum<visa-resource-name>, error out=w278:errorcluster)  [unwired: 1 in]
          n123 = disable-structure shown="Enabled" {
            disable-tunnel: [w293 w302] -> w283
            disable-tunnel: w278 -> [w297 w301]
            disable-tunnel: w279 -> [w296 w302]
            disable-tunnel: [w292 w301] -> w282
            frame Enabled {
              n124 = VISA Flush I/O Buffer(VISA resource name=w296, error in (no error)=w297) -> (VISA resource name out=w294:refnum<visa-resource-name>, error out=w295:errorcluster)  [unwired: 1 in]
              n125 = VISA Write(VISA resource name=w294, write buffer="Q", error in (no error)=w295) -> (VISA resource name out=w299:refnum<visa-resource-name>, error out=w298:errorcluster)  [unwired: 1 out]
              n126 = call "read caen.vi"("VISA in"=w299, "error in"=w298) -> ("VISA out"=w293:refnum<visa-resource-name>, "error out"=w292:errorcluster)  [unwired: 8 in, 4 out]
            }
            frame Disabled {
            }
          }
        }
        frame Disabled {
        }
      }
      n127 = disable-structure shown="Enabled" {
        disable-tunnel: [w259 _] -> w194
        disable-tunnel: w188 -> [w256 _]
        frame Enabled {
          n128 = Format Into String(format string="ASRL%d::INSTR" ("write buffer"), "LeCroy 1 Serial Port") -> (resulting string=w267:string, error out=w264:errorcluster)  [unwired: 2 in]
          n129 = call "Configure Serial.vi"("error in"=w264, "Resource Name"=w267) -> ("error out"=w265:errorcluster, "VISA out"=w266:refnum<visa-resource-name>)  [unwired: 8 in]
          n130 = VISA Flush I/O Buffer(VISA resource name=w266, error in (no error)=w265) -> (VISA resource name out=w262:refnum<visa-resource-name>, error out=w263:errorcluster)  [unwired: 1 in]
          n131 = VISA Write(VISA resource name=w262, write buffer="M01\r", error in (no error)=w263) -> (VISA resource name out=w261:refnum<visa-resource-name>, error out=w258:errorcluster)  [unwired: 1 out]
          n132 = call <userlib>:"Wait (ms)__ogtk.vi"("error in (no error)"=w258, "milliseconds to wait"=w256) -> ("error out"=w257:errorcluster)  [unwired: 8 in, 1 out]
          n133 = VISA Flush I/O Buffer(VISA resource name=w261, error in (no error)=w257) -> (VISA resource name out=w260:refnum<visa-resource-name>, error out=w259:errorcluster)  [unwired: 1 in]
          n134 = global write "CAEN globals.vi" "LeCroy 1 VISA"(w260) -> ()
        }
        frame Disabled {
        }
      }
      n135 = disable-structure shown="Enabled" {
        disable-tunnel: [w250 _] -> w193
        disable-tunnel: w188 -> [w240 _]
        frame Enabled {
          n136 = Format Into String(format string="ASRL%d::INSTR" ("write buffer"), "LeCroy 2 Serial Port") -> (resulting string=w253:string, error out=w254:errorcluster)  [unwired: 2 in]
          n137 = call "Configure Serial.vi"("error in"=w254, "Resource Name"=w253) -> ("error out"=w248:errorcluster, "VISA out"=w247:refnum<visa-resource-name>)  [unwired: 8 in]
          n138 = VISA Flush I/O Buffer(VISA resource name=w247, error in (no error)=w248) -> (VISA resource name out=w245:refnum<visa-resource-name>, error out=w244:errorcluster)  [unwired: 1 in]
          n139 = VISA Write(VISA resource name=w245, write buffer="M02\r", error in (no error)=w244) -> (VISA resource name out=w246:refnum<visa-resource-name>, error out=w242:errorcluster)  [unwired: 1 out]
          n140 = call <userlib>:"Wait (ms)__ogtk.vi"("error in (no error)"=w242, "milliseconds to wait"=w240) -> ("error out"=w241:errorcluster)  [unwired: 8 in, 1 out]
          n141 = VISA Flush I/O Buffer(VISA resource name=w246, error in (no error)=w241) -> (VISA resource name out=w249:refnum<visa-resource-name>, error out=w250:errorcluster)  [unwired: 1 in]
          n142 = global write "CAEN globals.vi" "LeCroy 2 VISA"(w249) -> ()
        }
        frame Disabled {
        }
      }
      n143 = for {
        tunnel: "Log Directory" -> [w276]
        tunnel: "Run" -> [w275]
        tunnel: "Subrun" -> [w274]
        tunnel: w199 -> [w273] mode=indexing
        tunnel: [w272] -> w206 mode=indexing
        tunnel: [w271] -> w198 mode=indexing
        tunnel: TRUE ("Append if exists?") -> [w270]
        n144 = call "Create Log or Log Directory.vi"("Base Directory"=w276, "Run"=w275, "Subrun"=w274, "Append if exists?"=w270, "Log Type"=w273) -> ("Path"=w272:path, "error out"=w271:errorcluster)  [unwired: 13 in]
      }
      n145 = Get Date/Time String(want seconds? (F)=TRUE) -> (date string=w218:string, time string=w217:string)  [unwired: 2 in]
      n146 = call <vilib>:"Space Constant.vi"() -> ("String"=w216:string)
      n147 = Concatenate Strings(w218, w216, w217) -> (w215:string)
      n148 = Index Array(array=w206) -> (element #1=w202:path, element #2=→"Current Channel Log":path, element #3=→"Current Error Log":path, element #4=→"Current ZMQ Log":path)  [unwired: 4 in]
      "Current Event Log" <- w202
      n149 = Merge Errors(w198) -> (w197:errorcluster)
      n150 = Concatenate Strings("Program started at " ("string"), w215) -> (w210:string)
      n151 = global write "CAEN globals.vi" "Current Event Log"(w202) -> ()
      n152 = call "Append to display log.vi"("error in"=w197, "string"=w210) -> ("error out"=w211:errorcluster)  [unwired: 9 in]
      n153 = call "Append to event log.vi"("error in"=w197, "string"="Program started ") -> ("error out"=w213:errorcluster)  [unwired: 9 in]
      n154 = global write "CAEN globals.vi" "CAEN VISA"(w189) -> ()
      n155 = Merge Errors(w213, w211) -> (w191:errorcluster)
      n156 = Merge Errors(w195, w194, w193, w187) -> (w192:errorcluster)
      n157 = call "get crate maps.vi"("error in"=w192) -> ("error out"=w196:errorcluster)  [unwired: 12 in, 2 out]
    }
  }
  n158 = Merge Errors(w20, w2, w38, w24, w46, w49, w39, w23) -> (w7:errorcluster)
  n159 = case shown="No Error" w7 {
    selector: w7 -> [w304 w2959]
    tunnel: FALSE ("READ") -> [w325 _]
    tunnel: 5000 -> [w324 _]
    tunnel: [w323 w2962] -> w55
    tunnel: w48 -> [w322 w2962]
    tunnel: w47 -> [w321 w2961]
    tunnel: w40 -> [w320 _]
    tunnel: w37 -> [w319 w2964]
    tunnel: [w318 w2964] -> w35
    tunnel: [w317 w2960] -> w33
    tunnel: [w316 w2959] -> w32
    tunnel: [w315 w2961] -> w29
    tunnel: -1 -> [w314 _]
    tunnel: w22 -> [w313 _]
    tunnel: w21 -> [w312 _]
    tunnel: w19 -> [w311 _]
    tunnel: [w310 TRUE ("stop")] -> w18
    tunnel: w17 -> [w309 _]
    tunnel: FALSE ("READ") -> [w308 _]
    tunnel: w8 -> [w307 _]
    tunnel: refnum<visa-resource-name> refnum ("VISA out") -> [w306 w2960]
    tunnel: w9 -> [w305 _]
    tunnel: [w303 w2957] -> w6
    frame No Error {
      n160 = while {
        shift-right: [w348] -> w316
        shift-left: w304 -> [w347]
        shift-right: [w349] -> _
        shift-left: w325 -> [w350]
        shift-right: [w346] -> _
        shift-left: w324 -> [w345]
        shift-right: [w343] -> w323
        shift-left: w322 -> [w344]
        tunnel: w311 -> [w340]
        tunnel: w321 -> [w342]
        tunnel: w309 -> [w341]
        tunnel: w320 -> [w339]
        tunnel: w307 -> [w338]
        tunnel: w319 -> [w337]
        tunnel: [w336] -> w315
        tunnel: [w335] -> w318
        shift-left: w304 -> [w334]
        tunnel: w314 -> [w333]
        tunnel: w313 -> [w332]
        tunnel: w312 -> [w331]
        shift-right: [w351] -> w317
        shift-left: w306 -> [w352]
        tunnel: [w330] -> w310
        shift-right: [w329] -> _
        shift-left: w308 -> [w328]
        tunnel: w305 -> [w327]
        tunnel: [w326] -> w303
        stop <- w330 stop-if-true
        # "Calling 'start new run' vs 'start new channel log, error log, event log' in ZMQ: is this achieving same thing?."
        n161 = case shown="No Error" w347 {
          selector: w347 -> [w374 w2731]
          tunnel: w352 -> [w356 w2729]
          tunnel: [w375 _] -> w330
          tunnel: [w356 w2730] -> w351
          tunnel: w345 -> [w359 w2733]
          tunnel: [w373 w2728] -> w348
          tunnel: [w372 w2733] -> w346
          tunnel: w345 -> [w371 _]
          tunnel: w344 -> [w370 w2732]
          tunnel: [w369 w2732] -> w343
          tunnel: w340 -> [w364 _]
          tunnel: w342 -> [w368 _]
          tunnel: w341 -> [w367 _]
          tunnel: w339 -> [w366 _]
          tunnel: w338 -> [w365 _]
          tunnel: w337 -> [w363 _]
          tunnel: [w362 _] -> w336
          tunnel: [w361 _] -> w335
          tunnel: w334 -> [w360 _]
          tunnel: w333 -> [_ _]
          tunnel: w332 -> [w358 _]
          tunnel: w331 -> [w357 _]
          tunnel: [w355 _] -> w329
          tunnel: w328 -> [w354 _]
          tunnel: w327 -> [w353 _]
          frame No Error {
            n162 = event shown="[0] Timeout" {
              selector: w370 -> [_ _ _ _ _ _ _ _ _ _ _ _ _ _ _ _ _ _ _ _ _ _ _ _ _ _ _ _ _ _ _ _ _ _ _ _ _ _ _ _ w2689 _ _ _ _]
              dyn-events: [_ _ _ _ _ _ _ _ _ _ _ _ _ _ _ _ _ _ _ _ _ _ _ _ _ _ _ _ _ _ _ _ _ _ _ _ _ _ _ _ w2693 _ _ _ _] -> w369
              timeout: w359 -> [_ _ _ w809 _ _ _ _ _ _ _ _ _ _ _ _ _ _ _ _ _ _ _ _ _ _ _ _ _ _ _ _ _ _ _ _ _ _ _ _ _ _ _ _ _]
              tunnel: w374 -> [_ _ _ _ _ _ _ _ _ _ _ _ _ _ _ _ _ _ _ _ _ _ _ _ _ _ _ _ _ _ _ _ _ _ _ _ _ _ _ _ _ _ _ _ _]
              tunnel: [_ _ _ _ _ _ _ _ _ _ _ _ _ _ _ _ _ _ _ _ _ _ _ _ _ _ _ _ _ _ _ _ _ _ _ _ _ _ _ _ _ _ _ _ "stop"] -> w375
              tunnel: [w387 w763 _ w811 _ w910 w993 w1063 w1142 w1166 w1259 w1342 w1382 w1435 w1465 w1487 w1497 w1509 w1523 w1580 w1703 w1724 w1767 w1840 w1869 w1882 w1896 w1916 w1927 w1939 w1967 w2007 w2066 w2088 w2132 w2338 _ w2405 w2597 w2635 w2696 w2706 w2713 w2721 w2725] -> w373
              tunnel: [_ _ "Ramp Voltages Slowly" _ "Redundant bool" "Read" "Write" _ _ _ _ _ _ _ "Start New Run" "Start New Error Log" "Start New Event Log" "Start New Channel Log" _ "Set channel property" _ "Set Group Property" "re-read vfile voltages" _ _ _ _ _ "Save PMT voltages" "Save PMT Voltage File" "Kill All" "Clear Alarms" "Refresh Crate Map" "get log file" "Handle ZMQ message" "Send ZMQ Reply" _ "Manual ZMQ Write" "Show Group In Displayed Channels" "Add Group to Displayed Channels" _ "Show hidden tabs" "'\\' codes display" "Line Wrapping" _] -> _
              tunnel: [_ _ _ _ _ _ _ _ _ _ _ _ _ _ _ _ _ _ "Channel Array" _ _ _ _ _ _ _ _ _ _ _ _ _ _ _ _ _ _ _ _ _ _ _ _ _ _] -> _
              tunnel: ["Scan Rate (ms)" w770 w799 w810 w863 w908 5000 w1065 w1141 w1176 w1263 w1343 w1383 w1441 w1464 w1492 w1505 w1518 w1521 w1581 w1705 w1725 w1763 w1836 w1863 w1876 w1890 w1914 w1932 w1945 5000 w2009 1000 w2102 w2140 w2360 50 ("Scan Rate (ms)") w2421 w2594 w2661 w2684 w2704 w2711 w2718 w2724] -> w372
              tunnel: w371 -> [_ w770 w799 _ w863 w908 _ w1065 w1141 w1176 w1263 w1343 w1383 w1441 w1464 w1492 w1505 w1518 w1521 w1581 w1705 w1725 w1763 w1836 w1863 w1876 w1890 w1914 w1932 w1945 _ w2009 _ w2102 w2140 w2360 _ w2421 w2594 w2661 w2684 w2704 w2711 w2718 w2724]
              tunnel: w364 -> [_ _ _ _ _ _ _ _ _ _ _ _ _ _ _ _ _ _ _ _ _ _ _ _ _ _ _ _ _ _ _ _ _ _ _ w2328 _ w2409 _ _ _ _ _ _ _]
              tunnel: w368 -> [_ _ _ _ _ _ _ _ _ _ _ _ _ _ _ _ _ _ _ _ _ _ _ _ _ _ _ _ _ _ _ _ _ _ _ _ _ _ _ _ w2686 _ _ _ w2723]
              tunnel: w367 -> [_ _ _ _ _ _ _ _ _ _ _ _ _ _ _ _ _ _ _ _ _ _ _ _ _ _ _ _ _ _ _ _ _ _ _ _ _ _ _ _ _ _ _ _ _]
              tunnel: w366 -> [_ _ _ _ _ _ _ _ _ w1153 _ _ _ w1436 _ _ _ _ _ _ _ _ _ _ _ _ _ _ _ _ _ _ _ _ _ _ _ _ _ _ _ _ _ _ _]
              tunnel: w365 -> [_ _ _ _ _ _ _ w1064 _ _ _ _ _ _ _ _ _ _ _ _ _ _ _ _ _ _ _ _ _ _ _ _ _ _ _ _ _ _ _ _ _ _ _ _ _]
              tunnel: w363 -> [w384 w773 _ _ _ _ _ _ _ _ _ _ _ _ _ _ _ _ _ _ _ _ w1764 w1837 _ _ _ _ w1931 _ _ _ _ _ w2136 _ _ _ _ _ _ _ _ _ w2722]
              tunnel: [_ _ _ _ _ _ _ _ _ _ _ _ _ _ _ _ _ _ _ _ _ _ _ _ _ _ _ _ _ _ _ _ _ _ _ _ _ _ _ _ _ _ _ _ w2723] -> w362
              tunnel: [_ w764 _ _ _ _ _ _ _ _ _ _ _ _ _ _ _ _ _ _ _ _ _ _ _ _ _ _ _ _ _ _ _ _ _ _ _ _ _ _ _ _ _ _ w2722] -> w361
              tunnel: w360 -> [_ _ _ _ _ _ _ _ _ _ _ _ _ _ _ _ _ _ _ _ _ _ _ _ _ _ _ _ _ _ _ _ _ _ _ _ w2385 _ _ _ _ _ _ _ _]
              tunnel: w358 -> [_ _ _ _ _ _ _ _ _ _ _ _ _ _ w1463 _ _ _ _ _ _ _ _ _ _ _ _ _ _ _ _ _ _ _ _ _ _ _ _ _ _ _ _ _ _]
              tunnel: w357 -> [_ _ _ _ _ _ _ _ _ _ _ _ _ _ w1462 _ _ _ _ _ _ _ _ _ _ _ _ _ _ _ _ _ _ _ _ _ _ _ _ _ _ _ _ _ _]
              tunnel: [_ "Abort queued actions" _ _ _ _ _ _ _ _ _ _ _ _ _ _ _ _ _ _ _ _ "Restore PMT voltages" "Nominal PMT voltages" _ _ _ _ _ _ _ _ _ _ _ _ _ _ _ _ _ _ _ _ _] -> _
              tunnel: [_ _ _ w808 _ _ _ _ _ _ _ _ _ _ _ _ _ _ _ _ _ _ _ _ _ _ _ _ _ _ _ _ _ _ _ _ _ _ _ _ _ _ _ _ _] -> w355
              tunnel: w354 -> [_ _ _ _ _ w907 _ _ _ _ _ _ _ _ _ _ _ _ _ _ _ _ _ _ _ _ _ _ _ _ _ _ _ _ _ _ _ _ _ _ _ _ _ _ _]
              tunnel: w353 -> [_ _ _ _ _ _ _ _ _ _ _ _ _ _ _ _ _ _ _ _ _ _ _ _ _ _ _ _ _ _ _ _ _ _ _ _ _ w2408 _ _ _ _ _ _ _]
              event Timeout {
                w380 = 0 ("Page")
                n163 = event-data() -> ()  [unwired: 1 in, 1 out]
                n164 = call "Operations queue.vi"("queue in"=w384) -> ("error out"=w385:errorcluster, "queue out"=w376:refnum<queue>)  [unwired: 7 in, 2 out]
                n165 = feedback #1(w380) -> (w383:i32)
                n166 = Dequeue Element(queue=w376, timeout in ms (-1)=0, error in (no error)=w385) -> (element=w388:cluster{"Source":T16, "Command":string}, timed out?=w390:bool, error out=w386:errorcluster)  [unwired: 1 out]
                n167 = Increment(x=w383) -> (x+1=w378:i32)
                n168 = Less?(x=w378, y=2 ("Page")) -> (x < y?=w382:bool)
                n169 = Select(t=w378, s=w382, f=w380) -> (s? t:f=w379:i32)
                n170 = feedback-in #1(w379) -> ()
                n171 = case shown="False" w390 {
                  tunnel: w388 -> [w396 _]
                  tunnel: [w393 w724] -> w387
                  tunnel: w376 -> [w392 _]
                  tunnel: w386 -> [_ _]
                  tunnel: w378 -> [_ w725]
                  tunnel: "scan" -> [_ w726]
                  frame False {
                    # "Handle Queued Event"
                    n172 = Unbundle(w396) -> ("Source"=w395:T16, "Command"=w394:string)
                    n173 = case shown="\"INTERNAL\"" w395 {
                      selector: w395 -> [_ _ w705 _ _ _ _]
                      tunnel: w394 -> [w397 _ w706 _ _ w715 _]
                      tunnel: [w400 _ w708 w710 w712 w716 w721] -> w393
                      tunnel: w392 -> [w399 _ w707 _ _ _ _]
                      frame "INTERNAL" {
                        # "msg_ID\nmsg_type\nmsg_property\nPMT_name\nPMT_value"
                        n174 = Spreadsheet String To Array(delimiter (Tab)="\r", format string="%s" ("spreadsheet string"), spreadsheet string=w397, array type (2D Dbl)=string[] []) -> (array=w406:string[])
                        n175 = Index Array(array=w406) -> (element #1=w404:string, element #2=w405:string, element #3=w403:string, element #4=w402:string, element #5=w401:string)  [unwired: 5 in]
                        n176 = case shown="\"write\"" w405 {
                          selector: w405 -> [_ _ w629 w638 w647 w659 w671 w681 w695]
                          tunnel: w404 -> [_ _ _ _ _ _ _ _ w697]
                          tunnel: w403 -> [w416 w512 _ _ _ _ w670 w680 _]
                          tunnel: w402 -> [w412 w504 _ _ _ _ _ _ _]
                          tunnel: w401 -> [_ w511 _ _ _ _ w668 _ _]
                          tunnel: [w414 w506 w634 w643 w652 w663 w676 w686 w692] -> w400
                          tunnel: w399 -> [_ _ w632 w641 w650 w661 w674 w684 _]
                          frame "read" {
                            n177 = global read "CAEN globals.vi" "Channel Array Val"() -> (w417:T8[])
                            n178 = call "Channel or group name to index.vi"("Name"=w412) -> ("Index"=w411:i32, "Group"=w410:bool, "error out"=w409:errorcluster)  [unwired: 10 in, 2 out]
                            n179 = local read "ZMQ Reply"() -> (w419:string[])
                            n180 = Index Array(array=w417, index=w411) -> (element=w415:T8)
                            n181 = case shown="True" w410 {
                              tunnel: w416 -> [w425 _]
                              tunnel: w415 -> [w424 _]
                              tunnel: [w423 w501] -> w414
                              tunnel: [w422 w499] -> w413
                              tunnel: w412 -> [w421 _]
                              tunnel: w409 -> [w420 _]
                              frame False {
                                n182 = case shown="\"enable\"" w425 {
                                selector: w425 -> [w432 _ _ _ _ _ _ _ _ _]
                                tunnel: w424 -> [_ w440 w447 w454 w461 w468 w477 w484 w491 w498]
                                tunnel: w421 -> [w431 w438 w445 w452 w459 w466 w475 w482 w489 w496]
                                tunnel: [w429 w437 w444 w451 w458 w465 w474 w481 w488 w495] -> w423
                                tunnel: [w428 w436 w443 w450 w457 w464 w473 w480 w487 w494] -> w422
                                tunnel: [w427 _ _ _ _ _ _ _ _ _] -> _
                                tunnel: w420 -> [w426 w434 w441 w448 w455 w462 w469 w478 w485 w492]
                                frame Default {
                                n183 = Format Into String(format string="\"error\":\"Unrecognised read property: %s for PMT %s\"" ("source"), error in=w426, w432, w431) -> (resulting string=w428:string, error out=w427:errorcluster)  [unwired: 1 in]
                                n184 = Bundle By Name(cluster=errorcluster {"status"=TRUE, "code"=0, "source"=""} ("error in"), "source"=w428) -> (w429:errorcluster)
                                }
                                frame "vset" {
                                n185 = Unbundle By Name(w440) -> ("Vset (V)"=w439:dbl)
                                n186 = Format Into String(format string="\"%s\":\"%.3f\"" ("source"), error in=w434, w438, w439) -> (resulting string=w436:string, error out=w437:errorcluster)  [unwired: 1 in]
                                }
                                frame "vmon" {
                                n187 = Unbundle By Name(w447) -> ("Vmon (V)"=w446:dbl)
                                n188 = Format Into String(format string="\"%s\":\"%.3f\"" ("source"), error in=w441, w445, w446) -> (resulting string=w443:string, error out=w444:errorcluster)  [unwired: 1 in]
                                }
                                frame "vswmax" {
                                n189 = Unbundle By Name(w454) -> ("Vswmax (V)"=w453:dbl)
                                n190 = Format Into String(format string="\"%s\":\"%d\"" ("source"), error in=w448, w452, w453) -> (resulting string=w450:string, error out=w451:errorcluster)  [unwired: 1 in]
                                }
                                frame "imax" {
                                n191 = Unbundle By Name(w461) -> ("Iset (A)"=w460:dbl)
                                n192 = Format Into String(format string="\"%s\":\"%.3pA\"" ("source"), error in=w455, w459, w460) -> (resulting string=w457:string, error out=w458:errorcluster)  [unwired: 1 in]
                                }
                                frame "imon" {
                                n193 = Unbundle By Name(w468) -> ("Imon (A)"=w467:dbl)
                                n194 = Format Into String(format string="\"%s\":\"%.3pA\"" ("source"), error in=w462, w466, w467) -> (resulting string=w464:string, error out=w465:errorcluster)  [unwired: 1 in]
                                }
                                frame "card", "channel", "crate" {
                                n195 = Unbundle By Name(w477) -> ("Crate"=w470:i32, "Card"=w476:i32, "Channel"=w471:i32)
                                n196 = Format Into String(format string="\"%s\":\"%d.%d.%02d\"" ("source"), error in=w469, w475, w470, w476, w471) -> (resulting string=w473:string, error out=w474:errorcluster)  [unwired: 1 in]
                                }
                                frame "status" {
                                n197 = Unbundle By Name(w484) -> ("Status"=w483:string)
                                n198 = Format Into String(format string="\"%s\":\"%s\"" ("source"), error in=w478, w482, w483) -> (resulting string=w480:string, error out=w481:errorcluster)  [unwired: 1 in]
                                }
                                frame "enable" {
                                n199 = Unbundle By Name(w491) -> ("ON/OFF"=w490:bool)
                                n200 = Format Into String(format string="\"%s\":\"%s\"" ("source"), error in=w485, w489, w490) -> (resulting string=w487:string, error out=w488:errorcluster)  [unwired: 1 in]
                                }
                                frame "timestamp" {
                                n201 = Unbundle By Name(w498) -> ("Timestamp"=w497:string)
                                n202 = Format Into String(format string="\"%s\":\"%s\"" ("source"), error in=w492, w496, w497) -> (resulting string=w494:string, error out=w495:errorcluster)  [unwired: 1 in]
                                }
                                }
                              }
                              frame True {
                                w499 = "\"error\":\"Read group property is not supported\"" ("spreadsheet string")
                                n203 = Bundle By Name(cluster=errorcluster {"status"=TRUE, "code"=0, "source"=""} ("error IO"), "source"=w499) -> (w501:errorcluster)
                              }
                            }
                            n204 = Build Array (concatenate)(w419, w413) -> (w418:string[])
                            n205 = local write "ZMQ Reply"(w418) -> ()
                          }
                          frame "write" {
                            # "Must us an event to note\nany errors generated"
                            n206 = call "Channel or group name to index.vi"("Name"=w504) -> ("Crate"=w505:i32, "Card.Channel"=w508:dbl, "Group"=w510:bool, "error out"=w509:errorcluster)  [unwired: 10 in, 1 out]
                            n207 = case shown="True" w510 {
                              tunnel: w512 -> [w525 w579]
                              tunnel: [w514 w578] -> w507
                              tunnel: w511 -> [w524 w577]
                              tunnel: w509 -> [w520 w575]
                              tunnel: w504 -> [w513 w572]
                              tunnel: w508 -> [w516 _]
                              tunnel: w505 -> [w515 _]
                              tunnel: [w513 w572] -> w502
                              frame False {
                                n208 = case shown="\"vset\"" w525 {
                                selector: w525 -> [w532 _ _ _ _ _ _]
                                tunnel: w524 -> [_ w538 w545 w552 w558 w565 w568]
                                tunnel: [w527 w539 w546 w553 w557 w561 w569] -> w519
                                tunnel: [_ w536 w543 w550 w560 w564 w570] -> w523
                                tunnel: [_ Channel_Properties."Vset" ("Property") Channel_Properties."Vbackup" ("Property") Channel_Properties."Vswmax" ("Property") Channel_Properties."Iset" ("Property") Channel_Properties."Enable" ("Property") Channel_Properties."Name" ("Property")] -> w522
                                tunnel: w520 -> [w529 w534 w541 w548 w555 w561 w569]
                                frame Default {
                                n209 = Format Into String(format string="Unrecognised or read-ony  property: %s" ("source"), error in=w529, w532) -> (resulting string=w530:string, error out=w526:errorcluster)  [unwired: 1 in]
                                n210 = Bundle By Name(cluster=errorcluster {"status"=TRUE, "code"=0, "source"=""} ("error in"), "source"=w530) -> (w528:errorcluster)
                                n211 = Merge Errors(w528, w526) -> (w527:errorcluster)
                                }
                                frame "vset" {
                                n212 = Scan From String(format string="%f" ("source"), input string=w538, error in=w534) -> (error out=w539:errorcluster, output 1=w537:dbl)  [unwired: 2 in, 2 out]
                                n213 = To Variant(anything=w537) -> (Variant=w536:variant)
                                }
                                frame "vbackup" {
                                n214 = Scan From String(format string="%f" ("source"), input string=w545, error in=w541) -> (error out=w546:errorcluster, output 1=w544:dbl)  [unwired: 2 in, 2 out]
                                n215 = To Variant(anything=w544) -> (Variant=w543:variant)
                                }
                                frame "vswmax" {
                                n216 = Scan From String(format string="%d" ("source"), input string=w552, error in=w548) -> (error out=w553:errorcluster, output 1=w551:i32)  [unwired: 2 in, 2 out]
                                n217 = To Variant(anything=w551) -> (Variant=w550:variant)
                                }
                                frame "imax" {
                                n218 = call "SI string to double.vi"("error in"=w555, "SI String"=w558) -> ("error out"=w557:errorcluster, "Numeric output"=w556:dbl)  [unwired: 6 in, 2 out]
                                n219 = To Variant(anything=w556) -> (Variant=w560:variant)
                                }
                                frame "enable" {
                                n220 = Equal?(x=w565, y="1" ("x")) -> (x = y?=w563:bool)
                                n221 = To Variant(anything=w563) -> (Variant=w564:variant)
                                }
                                frame "name" {
                                n222 = To Upper Case(1:w568) -> (0:w567:string)
                                n223 = To Variant(anything=w567) -> (Variant=w570:variant)
                                }
                                }
                                n224 = Bundle(cluster=T3 {" Card.Channel"=1.12, "Crate"=0} ("Set Card.Channel"), "Card.Channel"=w516, "Crate"=w515) -> (w517:T3)
                                n225 = local write "Set Card.Channel"(w517) -> ()
                                n226 = local write "Property"(w522) -> ()
                                n227 = local write "Value"(w523) -> ()
                                n228 = property on="Set channel property" class="Bool (strict)"(error in=w519, "Val(Sgnl)"=TRUE ("Value (Signaling)")) -> (error out=w514:errorcluster)  [unwired: 1 in, 1 out]
                              }
                              frame True {
                                n229 = case shown="Default" w579 {
                                selector: w579 -> [w586 _ _ _ _]
                                tunnel: w577 -> [_ w594 w602 w610 w615]
                                tunnel: [w580 w588 w597 w604 w613] -> w578
                                tunnel: [_ w593 w601 w609 w612] -> w574
                                tunnel: [_ Group_Properties."Vset" ("Group Prop") Group_Properties."Vswmax" ("Group Prop") Group_Properties."Imax" ("Group Prop") w611] -> w576
                                tunnel: w575 -> [w583 w591 w599 w607 w614]
                                frame Default {
                                n230 = Format Into String(format string="Unrecognised or read-ony  property: %s" ("source"), error in=w583, w586) -> (resulting string=w584:string, error out=w582:errorcluster)  [unwired: 1 in]
                                n231 = Bundle By Name(cluster=errorcluster {"status"=TRUE, "code"=0, "source"=""} ("error in"), "source"=w584) -> (w581:errorcluster)
                                n232 = Merge Errors(w581, w582) -> (w580:errorcluster)
                                }
                                frame "vset" {
                                n233 = Scan From String(format string="%f" ("source"), input string=w594, error in=w591) -> (error out=w589:errorcluster, output 1=w593:dbl)  [unwired: 2 in, 2 out]
                                n234 = property on="Set Group Property" class="Bool (strict)"(error in=w589, "Val(Sgnl)"=TRUE ("Value (Signaling)")) -> (error out=w588:errorcluster)  [unwired: 1 in, 1 out]
                                }
                                frame "vswmax" {
                                n235 = Scan From String(format string="%d" ("source"), input string=w602, error in=w599) -> (error out=w596:errorcluster, output 1=w601:i32)  [unwired: 2 in, 2 out]
                                n236 = property on="Set Group Property" class="Bool (strict)"(error in=w596, "Val(Sgnl)"=TRUE ("Value (Signaling)")) -> (error out=w597:errorcluster)  [unwired: 1 in, 1 out]
                                }
                                frame "imax" {
                                n237 = call "SI string to double.vi"("error in"=w607, "SI String"=w610) -> ("error out"=w605:errorcluster, "Numeric output"=w609:dbl)  [unwired: 6 in, 2 out]
                                n238 = property on="Set Group Property" class="Bool (strict)"(error in=w605, "Val(Sgnl)"=TRUE ("Value (Signaling)")) -> (error out=w604:errorcluster)  [unwired: 1 in, 1 out]
                                }
                                frame "enable" {
                                n239 = case shown="\"0\"" w615 {
                                tunnel: w614 -> [w617 w621 w625]
                                tunnel: [w616 w623 w624] -> w613
                                tunnel: [1.0 ("Card.Channel") _ 0.0 ("Card.Channel")] -> w612
                                tunnel: [Group_Properties."Enable" ("Group Prop") _ Group_Properties."Enable" ("Group Prop")] -> w611
                                frame "1" {
                                n240 = property on="Set Group Property" class="Bool (strict)"(error in=w617, "Val(Sgnl)"=TRUE ("Value (Signaling)")) -> (error out=w616:errorcluster)  [unwired: 1 in, 1 out]
                                }
                                frame Default {
                                n241 = Merge Errors(w621, errorcluster {"status"=TRUE, "code"=0, "source"="Unrecognised enable value"} ("error in")) -> (w623:errorcluster)
                                }
                                frame "0" {
                                n242 = property on="Set Group Property" class="Bool (strict)"(error in=w625, "Val(Sgnl)"=TRUE ("Value (Signaling)")) -> (error out=w624:errorcluster)  [unwired: 1 in, 1 out]
                                }
                                }
                                }
                                }
                                n243 = To Upper Case(1:w572) -> (0:w573:string)
                                n244 = local write "Group"(w573) -> ()
                                n245 = local write "Group Prop"(w576) -> ()
                                n246 = local write "Value 2"(w574) -> ()
                              }
                            }
                            n247 = property on="ZMQ_PMT_Err" class="Str"("Val(Sgnl)"=w502) -> (error out=w503:errorcluster)  [unwired: 2 in, 1 out]
                            n248 = Merge Errors(w507, w503) -> (w506:errorcluster)
                          }
                          frame "kill" {
                            n249 = property on="Kill All" class="Bool (strict)"("Val(Sgnl)"=TRUE ("Value (Signaling)")) -> (error out=w630:errorcluster)  [unwired: 2 in, 1 out]
                            n250 = Bundle(cluster=cluster{"Source":T16, "Command":string} {"Source"=enum."ZMQ", "Command"=""} ("element"), "Source"=Event_Sources."Check_Errors", "Command"=w629) -> (w637:cluster{"Source":T16, "Command":string})
                            n251 = Enqueue Element At Opposite End(queue=w632, element=w637) -> (error out=w635:errorcluster)  [unwired: 2 in, 2 out]
                            n252 = Merge Errors(w630, w635) -> (w634:errorcluster)
                          }
                          frame "clear" {
                            n253 = property on="Clear Alarms" class="Bool (strict)"("Val(Sgnl)"=TRUE ("Value (Signaling)")) -> (error out=w639:errorcluster)  [unwired: 2 in, 1 out]
                            n254 = Bundle(cluster=cluster{"Source":T16, "Command":string} {"Source"=enum."ZMQ", "Command"=""} ("element"), "Source"=Event_Sources."Check_Errors", "Command"=w638) -> (w646:cluster{"Source":T16, "Command":string})
                            n255 = Enqueue Element At Opposite End(queue=w641, element=w646) -> (error out=w644:errorcluster)  [unwired: 2 in, 2 out]
                            n256 = Merge Errors(w639, w644) -> (w643:errorcluster)
                          }
                          frame "map" {
                            n257 = property on="Refresh Crate Map" class="Bool (strict)"("Val(Sgnl)"=TRUE ("Value (Signaling)")) -> (error out=w648:errorcluster)  [unwired: 2 in, 1 out]
                            n258 = Bundle(cluster=cluster{"Source":T16, "Command":string} {"Source"=enum."ZMQ", "Command"=""} ("element"), "Source"=Event_Sources."Check_Errors", "Command"=w647) -> (w655:cluster{"Source":T16, "Command":string})
                            n259 = Enqueue Element At Opposite End(queue=w650, element=w655) -> (error out=w653:errorcluster)  [unwired: 2 in, 2 out]
                            n260 = Merge Errors(w648, w653) -> (w652:errorcluster)
                          }
                          frame "logs" {
                            w656 = TRUE ("Value (Signaling)")
                            n261 = property on="Start New Channel Log" class="Bool (strict)"("Val(Sgnl)"=w656) -> (error out=w660:errorcluster)  [unwired: 2 in, 1 out]
                            n262 = property on="Start New Error Log" class="Bool (strict)"("Val(Sgnl)"=w656) -> (error out=w658:errorcluster)  [unwired: 2 in, 1 out]
                            n263 = property on="Start New Event Log" class="Bool (strict)"("Val(Sgnl)"=w656) -> (error out=w657:errorcluster)  [unwired: 2 in, 1 out]
                            n264 = Bundle(cluster=cluster{"Source":T16, "Command":string} {"Source"=enum."ZMQ", "Command"=""} ("element"), "Source"=Event_Sources."Check_Errors", "Command"=w659) -> (w666:cluster{"Source":T16, "Command":string})
                            n265 = Enqueue Element At Opposite End(queue=w661, element=w666) -> (error out=w664:errorcluster)  [unwired: 2 in, 2 out]
                            n266 = Merge Errors(w660, w664, w658, w657) -> (w663:errorcluster)
                          }
                          frame "run" {
                            n267 = Decimal String To Number(string=w670) -> (number=w669:i32)  [unwired: 2 in, 1 out]
                            n268 = Decimal String To Number(string=w668) -> (number=w667:i32)  [unwired: 2 in, 1 out]
                            n269 = local write "Run"(w669) -> ()
                            n270 = local write "Subrun"(w667) -> ()
                            n271 = property on="Start New Run" class="Bool (strict)"("Val(Sgnl)"=TRUE ("Value (Signaling)")) -> (error out=w672:errorcluster)  [unwired: 2 in, 1 out]
                            n272 = Bundle(cluster=cluster{"Source":T16, "Command":string} {"Source"=enum."ZMQ", "Command"=""} ("element"), "Source"=Event_Sources."Check_Errors", "Command"=w671) -> (w679:cluster{"Source":T16, "Command":string})
                            n273 = Enqueue Element At Opposite End(queue=w674, element=w679) -> (error out=w677:errorcluster)  [unwired: 2 in, 2 out]
                            n274 = Merge Errors(w672, w677) -> (w676:errorcluster)
                          }
                          frame "get" {
                            n275 = property on="get log file" class="Bool (strict)"("Val(Sgnl)"=TRUE ("Value (Signaling)")) -> (error out=w682:errorcluster)  [unwired: 2 in, 1 out]
                            n276 = Bundle(cluster=cluster{"Source":T16, "Command":string} {"Source"=enum."ZMQ", "Command"=""} ("element"), "Source"=Event_Sources."Check_Errors", "Command"=w681) -> (w689:cluster{"Source":T16, "Command":string})
                            n277 = Enqueue Element At Opposite End(queue=w684, element=w689) -> (error out=w687:errorcluster)  [unwired: 2 in, 2 out]
                            n278 = Merge Errors(w682, w687) -> (w686:errorcluster)
                            "log file to get" <- w680
                          }
                          frame Default {
                            n279 = Format Into String(format string="Unrecognised ZMQ message type: %s for message ID %s" ("source"), w695, w697) -> (resulting string=w700:string, error out=w690:errorcluster)  [unwired: 2 in]
                            n280 = local read "ZMQ Reply"() -> (w702:string[])
                            n281 = Format Into String(format string="\"error\":\"unrecognised message type: %s\"" ("source"), w695) -> (resulting string=w696:string, error out=w691:errorcluster)  [unwired: 2 in]
                            n282 = Build Array (concatenate)(w702, w696) -> (w701:string[])
                            n283 = Bundle By Name(cluster=errorcluster {"status"=TRUE, "code"=0, "source"=""} ("error in"), "source"=w700) -> (w693:errorcluster)
                            n284 = local write "ZMQ Reply"(w701) -> ()
                            n285 = Merge Errors(w693, w690, w691) -> (w692:errorcluster)
                          }
                        }
                      }
                      frame "Check_Errors" {
                        # "Deprecated case, not used"
                      }
                      frame "ZMQ" {
                        # "perform message interpretation"
                        n286 = Bundle("Source"=w705, "Command"=w706) -> (w704:cluster{"Source":T16, "Command":string})  [unwired: 1 in]
                        n287 = Enqueue Element At Opposite End(queue=w707, element=w704) -> (error out=w703:errorcluster)  [unwired: 2 in, 2 out]
                        n288 = property on="Handle ZMQ message" class="Bool (strict)"(error in=w703, "Val(Sgnl)"=TRUE ("Value (Signaling)")) -> (error out=w708:errorcluster)  [unwired: 1 in, 1 out]
                      }
                      frame "Send_ZMQ_Reply" {
                        # "perform message interpretation"
                        n289 = property on="Send ZMQ Reply" class="Bool (strict)"("Val(Sgnl)"=TRUE ("Value (Signaling)")) -> (error out=w710:errorcluster)  [unwired: 2 in, 1 out]
                      }
                      frame "Save_PMT_Voltages" {
                        # "perform message interpretation"
                        n290 = property on="Save PMT Voltage File" class="Bool (strict)"("Val(Sgnl)"=TRUE ("Value (Signaling)")) -> (error out=w712:errorcluster)  [unwired: 2 in, 1 out]
                      }
                      frame "Set_Ramp_Voltage" {
                        n291 = Fract/Exp String To Number(string=w715) -> (number=w714:dbl)  [unwired: 3 in, 1 out]
                        n292 = local write "Value 2"(w714) -> ()
                        n293 = property on="Group Prop" class="Enum (strict)"("Val(Sgnl)"=Group_Properties."Vset" ("Value (Signaling)")) -> (error out=w717:errorcluster)  [unwired: 2 in, 1 out]
                        n294 = local write "Group"("ACTIVE" ("Group")) -> ()
                        n295 = property on="Set Group Property" class="Bool (strict)"(error in=w717, "Val(Sgnl)"=TRUE ("Value (Signaling)")) -> (error out=w716:errorcluster)  [unwired: 1 in, 1 out]
                      }
                      frame "Restore PMT Voltages" {
                        n296 = property on="Restore PMT voltages" class="Bool (strict)"("Val(Sgnl)"=TRUE ("Value (Signaling)")) -> (error out=w721:errorcluster)  [unwired: 2 in, 1 out]
                      }
                    }
                  }
                  frame True {
                    # "No Queued Events - Trigger Idle Read"
                    n297 = case shown="True" w726 {
                      tunnel: w725 -> [_ w738]
                      tunnel: [w728 w739] -> w723
                      frame False {
                        # "read any trailing info from read buffers"
                        # "Page Scanning Paused"
                        n298 = for {
                          N: 3 -> [_]
                          tunnel: [w731] -> w728 mode=indexing
                          i -> [w730]
                          # "skip reads if we're already busy"
                          n299 = case shown="0" w730 {
                            tunnel: [w734 w735 TRUE ("Reading page") w737] -> w729
                            frame 1 {
                              n300 = local read "Reading LeCroy1 Page"() -> (w734:bool)
                            }
                            frame 2 {
                              n301 = local read "Reading LeCroy2 Page"() -> (w735:bool)
                            }
                            frame Default {
                            }
                            frame 0 {
                              n302 = local read "Reading page"() -> (w737:bool)
                            }
                          }
                          n303 = case shown="False" w729 {
                            tunnel: [w733 _] -> w731
                            tunnel: w730 -> [w732 _]
                            frame False {
                              n304 = property on="Read Crate" class="DigNum (strict)"("Val(Sgnl)"=w732) -> (error out=w733:errorcluster)  [unwired: 2 in, 1 out]
                            }
                            frame True {
                            }
                          }
                        }
                      }
                      frame True {
                        # "Scan Through Pages - Trigger Next Page Read"
                        n305 = case shown="2" w738 {
                          tunnel: [w741 w752] -> w739
                          frame Default {
                            n306 = for {
                              N: 3 -> [_]
                              tunnel: [w744] -> w741 mode=indexing
                              i -> [w743]
                              # "read any trailing info from read buffers"
                              n307 = case shown="0" w743 {
                                tunnel: [w747 w748 TRUE ("Reading page") w750] -> w742
                                frame 1 {
                                n308 = local read "Reading LeCroy1 Page"() -> (w747:bool)
                                }
                                frame 2 {
                                n309 = local read "Reading LeCroy2 Page"() -> (w748:bool)
                                }
                                frame Default {
                                }
                                frame 0 {
                                n310 = local read "Reading page"() -> (w750:bool)
                                }
                              }
                              n311 = case shown="False" w742 {
                                tunnel: [w746 _] -> w744
                                tunnel: w743 -> [w745 _]
                                frame False {
                                n312 = property on="Read Crate" class="DigNum (strict)"("Val(Sgnl)"=w745) -> (error out=w746:errorcluster)  [unwired: 2 in, 1 out]
                                }
                                frame True {
                                }
                              }
                            }
                          }
                          frame 2 {
                            n313 = for {
                              N: 3 -> [_]
                              tunnel: [w755] -> w752 mode=indexing
                              i -> [w754]
                              # "read the next page from each crate"
                              n314 = case shown="0" w754 {
                                tunnel: [w758 w759 TRUE ("Reading page") w761] -> w753
                                frame 1 {
                                n315 = local read "Reading LeCroy1 Page"() -> (w758:bool)
                                }
                                frame 2 {
                                n316 = local read "Reading LeCroy2 Page"() -> (w759:bool)
                                }
                                frame Default {
                                }
                                frame 0 {
                                n317 = local read "Reading page"() -> (w761:bool)
                                }
                              }
                              n318 = case shown="False" w753 {
                                tunnel: [w757 _] -> w755
                                tunnel: w754 -> [w756 _]
                                frame False {
                                n319 = property on="Read Crate Page" class="DigNum (strict)"("Val(Sgnl)"=w756) -> (error out=w757:errorcluster)  [unwired: 2 in, 1 out]
                                }
                                frame True {
                                }
                              }
                            }
                          }
                        }
                      }
                    }
                    n320 = Merge Errors(w723) -> (w724:errorcluster)
                  }
                }
              }
              event "Abort queued actions": Value Change {
                n321 = event-data() -> ()  [unwired: 1 in, 1 out]
                n322 = Get Queue Status(queue=w773, return elements? (F)=TRUE) -> (queue out=w768:refnum<queue>, error out=w767:errorcluster, elements=w769:cluster{"Source":T16, "Command":string}[])  [unwired: 1 in, 5 out]
                n323 = Flush Queue(queue=w768, error in (no error)=w767) -> (queue out=w765:refnum<queue>, error out=w766:errorcluster)  [unwired: 1 out]
                n324 = for {
                  tunnel: w769 -> [w775] mode=indexing
                  shift-right: [w776] -> w763
                  shift-left: w766 -> [w778]
                  shift-right: [w777] -> w764
                  shift-left: w765 -> [w779]
                  n325 = Unbundle By Name(w775) -> ("Source"=w774:T16)
                  n326 = case shown="Default" w774 {
                    tunnel: w779 -> [w781 w787]
                    tunnel: w778 -> [w780 w786]
                    tunnel: [w781 w785] -> w777
                    tunnel: [w780 w784] -> w776
                    tunnel: w775 -> [_ w783]
                    frame "INTERNAL" {
                    }
                    frame Default {
                      n327 = Enqueue Element(queue=w787, element=w783, timeout in ms (-1)=500, error in (no error)=w786) -> (queue out=w785:refnum<queue>, error out=w784:errorcluster)  [unwired: 1 out]
                    }
                  }
                }
                n328 = global write "CAEN globals.vi" "Held Actions"(T21 [] ("Held Actions")) -> ()
              }
              event "Ramp Voltages Slowly": Value Change {
                (unwired) cluster{"Source":T16, "Command":string} {"Source"=enum."Restore PMT Voltages", "Command"="0"} ("element")
                w798 = dbl[] [0.0, 60.0, 120.0, 180.0]  # Delays in mins
                # "this needs to have a manual override.\nyou have to be able to see queued operations and delete them\nbefore they occur. \nalso possibly add a queued operation"
                # "make entry string more general so that\nthe event case in timeout can be used to\nset more than just group active voltages"
                n329 = event-data() -> ()  [unwired: 1 in, 1 out]
                n330 = local write "Ramp Voltages Slowly"(FALSE ("Ramp Voltages Slowly")) -> ()
                n331 = Get Date/Time In Seconds() -> (seconds since 1Jan1904=w795:timestamp)
                n332 = Multiply(x=w798, y=60.0 ("Group Value")) -> (x*y=w796:dbl[])
                n333 = Add(x=w795, y=w796) -> (x+y=w789:timestamp[])
                n334 = Build Array(cluster{"Source":T16, "Command":string} {"Source"=enum."Set_Ramp_Voltage", "Command"="200"} ("element"), cluster{"Source":T16, "Command":string} {"Source"=enum."Set_Ramp_Voltage", "Command"="400"} ("element"), cluster{"Source":T16, "Command":string} {"Source"=enum."Set_Ramp_Voltage", "Command"="700"} ("element"), cluster{"Source":T16, "Command":string} {"Source"=enum."Set_Ramp_Voltage", "Command"="1000"} ("element")) -> (w788:cluster{"Source":T16, "Command":string}[])
                n335 = for {
                  tunnel: w789 -> [w803] mode=indexing
                  tunnel: w788 -> [w802] mode=indexing
                  n336 = global read "CAEN globals.vi" "Held Actions"() -> (w804:T21)
                  n337 = Bundle("Group Value"=w803, "element"=w802) -> (w801:T26)  [unwired: 1 in]
                  n338 = Build Array (concatenate)(w804, w801) -> (w805:T27)
                  n339 = global write "CAEN globals.vi" "Held Actions"(w805) -> ()
                }
              }
              event Key Down? {
                n340 = event-data() -> ("VKey"=w812:T28, "Char"=w813:i16)  [unwired: 1 in]
                n341 = Tick Count (ms)() -> (millisecond timer value=w807:u32)
                n342 = while {
                  tunnel: w807 -> [w857]
                  tunnel: [w852] -> w806
                  stop <- w859 stop-if-true
                  # "if we're in the process of a page read, \nwait up to 6s for it to finish, \nthen timeout and abandon the key send."
                  n343 = Tick Count (ms)() -> (millisecond timer value=w858:u32)
                  n344 = local read "stop"() -> (w853:bool)
                  n345 = local read "Reading page"() -> (w860:bool)
                  n346 = Subtract(x=w858, y=w857) -> (x-y=w856:u32)
                  n347 = Greater?(x=w856, y=u32 6000) -> (0:w854:bool)
                  n348 = Or(x=w854, y=w853) -> (x .or. y?=w852:bool)
                  n349 = Wait (ms)(milliseconds to wait=u32 50) -> ()  [unwired: 1 out]
                  n350 = Compound Arithmetic op=OR(w852, invert w860) -> (w859:bool)
                }
                n351 = case shown="False" w806 {
                  tunnel: w813 -> [w824 _]
                  tunnel: w812 -> [w823 _]
                  tunnel: [w822 _] -> w811
                  tunnel: [w818 _] -> w808
                  tunnel: [w819 w850] -> w810
                  tunnel: w809 -> [w817 w850]
                  frame False {
                    n352 = case shown="\"Up\"" w823 {
                      tunnel: w824 -> [w841 _ _ _ _ _ _]
                      tunnel: [w840 "" ("search string") "\r" ("search string") "\u001b[A" ("search string") "\u001b[B" ("search string") "\u001b[D" ("search string") "\u001b[C" ("search string")] -> w821
                      tunnel: [_ TRUE ("Value (Signaling)") _ _ _ _ _] -> w820
                      frame "ASCII" {
                        n353 = Build Array(w841) -> (w842:i16[])
                        n354 = Byte Array To String(unsigned byte array=w842) -> (string=w840:string)
                      }
                      frame Default {
                      }
                      frame "Enter", "Return" {
                      }
                      frame "Up" {
                      }
                      frame "Down" {
                      }
                      frame "Left" {
                      }
                      frame "Right" {
                      }
                    }
                    n355 = call "Get Mainframe VISA.vi"("Crate"=0) -> ("Error Out"=w815:errorcluster, "VISA out"=w816:refnum<visa-resource-name>)  [unwired: 8 in, 1 out]
                    n356 = case shown="False" w820 {
                      tunnel: w816 -> [w838 _]
                      tunnel: [w834 _] -> w822
                      tunnel: w821 -> [w830 _]
                      tunnel: [w833 _] -> _
                      tunnel: [5000 w839] -> w819
                      tunnel: [TRUE ("READ") _] -> w818
                      tunnel: w817 -> [_ w839]
                      tunnel: w815 -> [w825 _]
                      frame False {
                        n357 = VISA Write(VISA resource name=w838, write buffer=w830, error in (no error)=w825) -> (error out=w835:errorcluster)  [unwired: 2 out]
                        n358 = call <userlib>:"Wait (ms)__ogtk.vi"("error in (no error)"=w835, "milliseconds to wait"=u32 10) -> ("error out"=w837:errorcluster)  [unwired: 8 in, 1 out]
                        n359 = property on="Read Crate" class="DigNum (strict)"(error in=w837, "Val(Sgnl)"=0 ("Value (Signaling)")) -> (error out=w834:errorcluster)  [unwired: 1 in, 1 out]
                        n360 = Concatenate Strings("Sending key '" ("string"), w830, "'" ("string")) -> (w832:string)
                        n361 = call "Append to display log.vi"("string"=w832) -> ("error out"=w833:errorcluster)  [unwired: 10 in]
                        "Key sent" <- w830
                      }
                      frame True {
                      }
                    }
                  }
                  frame True {
                    # "timed out waiting for a page read to finish,\nor 'Stop' button was pressed. Abandon the write."
                  }
                }
                n362 = event-data() -> ()  [unwired: 2 in, 1 out]
              }
              event "Redundant bool": Value Change {
                # "Redundant case: See 'restore PMT Voltages' event to re-read Vfile values from file,\nor see 'Nominal PMT voltages' event for restoring from internal Vfile to Vset"
                n363 = event-data() -> ()  [unwired: 1 in, 6 out]
                n364 = global read "CAEN globals.vi" "Channel Array Val"() -> (w862:T8[])
                n365 = for {
                  tunnel: w862 -> [w891] mode=indexing
                  stop <- FALSE stop-if-true
                  w883 = "." ("string")
                  # "Held actions are more useful for adding times to events\notherwise this is the same as just adding to the queue"
                  # "msg_ID                 (unused)\nmsg_type             (write) \nmsg_property      (vset)\nPMT_name           (crate.card.channel)\nPMT_value           (vset value)"
                  # "msg_id -999 generates no response"
                  n366 = Unbundle By Name(w891) -> ("Crate"=w864:i32, "Card"=w871:i32, "Channel"=w888:i32, "Vfile (V)"=w887:dbl)
                  n367 = Equal To 0?(x=w864) -> (x = 0?=w873:bool)
                  n368 = Number To Decimal String(number=w871) -> (decimal integer string=w885:string)  [unwired: 1 in]
                  n369 = Number To Decimal String(number=w888) -> (decimal integer string=w884:string)  [unwired: 1 in]
                  n370 = Number To Fractional String(number=w887) -> (F-format string=w880:string)  [unwired: 3 in]
                  n371 = Number To Decimal String(number=w864) -> (decimal integer string=w886:string)  [unwired: 1 in]
                  n372 = Concatenate Strings(w886, w883, w885, w883, w884) -> (w881:string)
                  n373 = Select(t="vset" ("format string"), s=w873, f="vbackup" ("format string")) -> (s? t:f=w874:string)
                  n374 = Build Array (concatenate)(string[] ["-999", "write"] ("array type (2D Dbl)"), w874, w881, w880) -> (w879:string[])
                  n375 = Array To Spreadsheet String(delimiter (Tab)="\r", array=w879, 3:"%s" ("spreadsheet string")) -> (spreadsheet string=w872:string)
                  n376 = Bundle By Name(cluster=cluster{"Source":T16, "Command":string} {"Source"=enum."ZMQ", "Command"=""} ("element"), "Command"=w872, "Source"=Event_Sources."INTERNAL") -> (w868:cluster{"Source":T16, "Command":string})
                  n377 = global read "CAEN globals.vi" "Held Actions"() -> (w866:T21)
                  n378 = Get Date/Time In Seconds() -> (seconds since 1Jan1904=w869:timestamp)
                  n379 = Bundle("seconds since 1Jan1904"=w869, "element"=w868) -> (w867:T29)  [unwired: 1 in]
                  n380 = case shown="4" w864 {
                    tunnel: w867 -> [_ w895]
                    tunnel: w866 -> [w892 w894]
                    tunnel: [w892 w893] -> w865
                    frame 4 {
                    }
                    frame Default {
                      n381 = Build Array (concatenate)(w894, w895) -> (w893:T21)
                    }
                  }
                  n382 = global write "CAEN globals.vi" "Held Actions"(w865) -> ()
                }
              }
              event "Read", "Read Crate": Value Change {
                n383 = event-data() -> ("CtlRef"=w906:refnum<vi>, "NewVal"=w899:variant)  [unwired: 1 in]
                n384 = control-ref of="Read Crate"() -> (w903:refnum<vi>)
                n385 = local read "Config pg Crate"() -> (w905:i32)
                n386 = Equal?(x=w903, y=w906) -> (x = y?=w904:bool)
                n387 = Variant To Data(type="Read Crate", Variant=w899) -> (data=w897:i32, error out=w896:errorcluster)  [unwired: 1 in]
                n388 = Tick Count (ms)() -> (millisecond timer value=w901:u32)
                n389 = Select(t=w897, s=w904, f=w905) -> (s? t:f=w902:i32)
                n390 = local write "Read"(FALSE ("READ")) -> ()
                n391 = case shown="0" w902 {
                  tunnel: w901 -> [w950 w962 w974 _]
                  tunnel: [w949 w961 w973 _] -> w900
                  tunnel: w896 -> [_ _ _ _]
                  frame 0 {
                    n392 = while {
                      tunnel: w950 -> [w958]
                      tunnel: [w953] -> w949
                      stop <- w960 stop-if-true
                      # "if we're in the process of a page read, \nwait up to 6s for it to finish, \nthen timeout and abandon the read."
                      n393 = Tick Count (ms)() -> (millisecond timer value=w959:u32)
                      n394 = local read "stop"() -> (w954:bool)
                      n395 = local read "Reading page"() -> (w951:bool)
                      n396 = Subtract(x=w959, y=w958) -> (x-y=w957:u32)
                      n397 = Greater?(x=w957, y=u32 6000) -> (0:w955:bool)
                      n398 = Or(x=w955, y=w954) -> (x .or. y?=w953:bool)
                      n399 = Wait (ms)(milliseconds to wait=u32 50) -> ()  [unwired: 1 out]
                      n400 = Compound Arithmetic op=OR(w953, invert w951) -> (w960:bool)
                    }
                  }
                  frame 1 {
                    n401 = while {
                      tunnel: w962 -> [w970]
                      tunnel: [w965] -> w961
                      stop <- w972 stop-if-true
                      # "if we're in the process of a page read, \nwait up to 6s for it to finish, \nthen timeout and abandon the read."
                      n402 = local read "Reading LeCroy1 Page"() -> (w963:bool)
                      n403 = Tick Count (ms)() -> (millisecond timer value=w971:u32)
                      n404 = local read "stop"() -> (w966:bool)
                      n405 = Subtract(x=w971, y=w970) -> (x-y=w969:u32)
                      n406 = Greater?(x=w969, y=u32 6000) -> (0:w967:bool)
                      n407 = Or(x=w967, y=w966) -> (x .or. y?=w965:bool)
                      n408 = Wait (ms)(milliseconds to wait=u32 50) -> ()  [unwired: 1 out]
                      n409 = Compound Arithmetic op=OR(w965, invert w963) -> (w972:bool)
                    }
                  }
                  frame 2 {
                    n410 = while {
                      tunnel: w974 -> [w982]
                      tunnel: [w977] -> w973
                      stop <- w984 stop-if-true
                      # "if we're in the process of a page read, \nwait up to 6s for it to finish, \nthen timeout and abandon the read."
                      n411 = local read "Reading LeCroy2 Page"() -> (w975:bool)
                      n412 = Tick Count (ms)() -> (millisecond timer value=w983:u32)
                      n413 = local read "stop"() -> (w978:bool)
                      n414 = Subtract(x=w983, y=w982) -> (x-y=w981:u32)
                      n415 = Greater?(x=w981, y=u32 6000) -> (0:w979:bool)
                      n416 = Or(x=w979, y=w978) -> (x .or. y?=w977:bool)
                      n417 = Wait (ms)(milliseconds to wait=u32 50) -> ()  [unwired: 1 out]
                      n418 = Compound Arithmetic op=OR(w977, invert w975) -> (w984:bool)
                    }
                  }
                  frame Default {
                    # "unknown crate"
                  }
                }
                n419 = case shown="False" w900 {
                  tunnel: [w916 w947] -> w910
                  tunnel: w907 -> [w915 _]
                  tunnel: w902 -> [w913 _]
                  frame False {
                    n420 = call "Get Mainframe VISA.vi"("Crate"=w913) -> ("Error Out"=w912:errorcluster, "VISA out"=w914:refnum<visa-resource-name>)  [unwired: 8 in, 1 out]
                    n421 = case shown="0" w913 {
                      selector: w913 -> [w923 _]
                      tunnel: w914 -> [w918 w936]
                      tunnel: [w924 w935] -> w916
                      tunnel: w915 -> [_ w934]
                      tunnel: w912 -> [w917 w929]
                      frame Default {
                        n422 = property class="Instr"(reference=w918, error in=w917) -> (reference out=w922:refnum<visa-resource-name>, error out=w921:errorcluster, "Serial Settings:Number of Bytes at Serial Port"=w920:u32)
                        n423 = VISA Read(VISA resource name=w922, byte count=w920, error in (no error)=w921) -> (read buffer=w919:string, error out=w924:errorcluster)  [unwired: 2 out]
                        n424 = case shown="1" w923 {
                          tunnel: w919 -> [_ w925 w927]
                          frame Default {
                          }
                          frame 2 {
                            n425 = case shown="Default" w925 {
                              selector: w925 -> [_ w926]
                              frame "" {
                              }
                              frame Default {
                                "Read buffer LeCroy 2" <- w926
                              }
                            }
                          }
                          frame 1 {
                            n426 = case shown="Default" w927 {
                              selector: w927 -> [_ w928]
                              frame "" {
                              }
                              frame Default {
                                "Read buffer LeCroy 1" <- w928
                              }
                            }
                          }
                        }
                      }
                      frame 0 {
                        # "Already updated in Read Caen vi"
                        n427 = case shown="True" w934 {
                          tunnel: [u32 150 ("Short Loop Read Time (ms)") w942] -> w931
                          tunnel: [u32 310 ("First read time (ms)") w941] -> w930
                          frame False {
                          }
                          frame True {
                            n428 = local read "Key sent"() -> (w940:string)
                            n429 = To Lower Case(string=w940) -> (all lower case string=w939:string)
                            n430 = case shown="Default" w939 {
                              tunnel: [u32 50 ("First read time (ms)") u32 150 ("Short Loop Read Time (ms)")] -> w942
                              tunnel: [u32 150 ("First read time (ms)") u32 310 ("First read time (ms)")] -> w941
                              frame Default {
                              }
                              frame "g", "n", "p" {
                              }
                            }
                          }
                        }
                        n431 = call "read caen.vi"("VISA in"=w936, "Extended Delay"=FALSE, "error in"=w929, "First read time (ms)"=w930, "Short Loop Read Time (ms)"=w931) -> ("error out"=w932:errorcluster)  [unwired: 5 in, 5 out]
                        n432 = call <vilib>:"Clear Errors.vi"("error in (no error)"=w932) -> ("error out"=w935:errorcluster)  [unwired: 5 in, 1 out]
                      }
                    }
                  }
                  frame True {
                    n433 = disable-structure shown="Disabled" {
                      disable-tunnel: [errorcluster {"status"=TRUE, "code"=0, "source"="Skipped manual read due to timeout waiting\nfor page read"} ("error out") _] -> w947
                      frame Disabled {
                      }
                      frame Enabled {
                      }
                    }
                  }
                }
              }
              event "Write": Value Change {
                n434 = event-data() -> ()  [unwired: 1 in, 1 out]
                n435 = Tick Count (ms)() -> (millisecond timer value=w985:u32)
                n436 = case shown="1" "Config pg Crate" {
                  tunnel: [w1023 w1035 w1047 _] -> w987
                  tunnel: w985 -> [w1022 w1034 w1046 _]
                  frame 0 {
                    n437 = while {
                      tunnel: w1022 -> [w1030]
                      tunnel: [w1025] -> w1023
                      stop <- w1032 stop-if-true
                      # "if we're in the process of a page read, \nwait up to 6s for it to finish, \nthen timeout and abandon the write."
                      n438 = Tick Count (ms)() -> (millisecond timer value=w1031:u32)
                      n439 = local read "stop"() -> (w1026:bool)
                      n440 = local read "Reading page"() -> (w1033:bool)
                      n441 = Subtract(x=w1031, y=w1030) -> (x-y=w1029:u32)
                      n442 = Greater?(x=w1029, y=u32 6000) -> (0:w1027:bool)
                      n443 = Or(x=w1027, y=w1026) -> (x .or. y?=w1025:bool)
                      n444 = Wait (ms)(milliseconds to wait=u32 500) -> ()  [unwired: 1 out]
                      n445 = Compound Arithmetic op=OR(w1025, invert w1033) -> (w1032:bool)
                    }
                  }
                  frame 1 {
                    n446 = while {
                      tunnel: w1034 -> [w1042]
                      tunnel: [w1037] -> w1035
                      stop <- w1044 stop-if-true
                      # "if we're in the process of a page read, \nwait up to 6s for it to finish, \nthen timeout and abandon the write."
                      n447 = local read "Reading LeCroy1 Page"() -> (w1045:bool)
                      n448 = Tick Count (ms)() -> (millisecond timer value=w1043:u32)
                      n449 = local read "stop"() -> (w1038:bool)
                      n450 = Subtract(x=w1043, y=w1042) -> (x-y=w1041:u32)
                      n451 = Greater?(x=w1041, y=u32 6000) -> (0:w1039:bool)
                      n452 = Or(x=w1039, y=w1038) -> (x .or. y?=w1037:bool)
                      n453 = Wait (ms)(milliseconds to wait=u32 500) -> ()  [unwired: 1 out]
                      n454 = Compound Arithmetic op=OR(w1037, invert w1045) -> (w1044:bool)
                    }
                  }
                  frame 2 {
                    n455 = while {
                      tunnel: w1046 -> [w1054]
                      tunnel: [w1049] -> w1047
                      stop <- w1056 stop-if-true
                      # "if we're in the process of a page read, \nwait up to 6s for it to finish, \nthen timeout and abandon the write."
                      n456 = local read "Reading LeCroy2 Page"() -> (w1057:bool)
                      n457 = Tick Count (ms)() -> (millisecond timer value=w1055:u32)
                      n458 = local read "stop"() -> (w1050:bool)
                      n459 = Subtract(x=w1055, y=w1054) -> (x-y=w1053:u32)
                      n460 = Greater?(x=w1053, y=u32 6000) -> (0:w1051:bool)
                      n461 = Or(x=w1051, y=w1050) -> (x .or. y?=w1049:bool)
                      n462 = Wait (ms)(milliseconds to wait=u32 500) -> ()  [unwired: 1 out]
                      n463 = Compound Arithmetic op=OR(w1049, invert w1057) -> (w1056:bool)
                    }
                  }
                  frame Default {
                  }
                }
                n464 = local write "Write"(FALSE ("Write")) -> ()
                n465 = call "Append to display log.vi"("string"="Performing manual write") -> ("error out"=w989:errorcluster)  [unwired: 10 in]
                n466 = call <vilib>:"Clear Errors.vi"("error in (no error)"=w989) -> ("error out"=w988:errorcluster)  [unwired: 5 in, 1 out]
                n467 = case shown="False" w987 {
                  tunnel: [w1000 errorcluster {"status"=TRUE, "code"=0, "source"="Skipping manual write due to read page timeout"} ("error out")] -> w993
                  tunnel: "Config pg Crate" -> [w995 _]
                  tunnel: w988 -> [w998 _]
                  frame False {
                    n468 = call "Get Mainframe VISA.vi"("Crate"=w995) -> ("Error Out"=w997:errorcluster, "VISA out"=w996:refnum<visa-resource-name>)  [unwired: 8 in, 1 out]
                    n469 = case shown="Default" w995 {
                      selector: w995 -> [w1001 _]
                      tunnel: [w1012 w1019] -> w1000
                      tunnel: "Write buffer" -> [w1013 w1018]
                      tunnel: w998 -> [_ _]
                      tunnel: w997 -> [w1003 _]
                      tunnel: w996 -> [w1002 w1020]
                      frame Default {
                        n470 = VISA Write(VISA resource name=w1002, write buffer=w1013, error in (no error)=w1003) -> (VISA resource name out=w1010:refnum<visa-resource-name>, error out=w1011:errorcluster)  [unwired: 1 out]
                        n471 = call <userlib>:"Wait (ms)__ogtk.vi"("error in (no error)"=w1011, "milliseconds to wait"="delay (ms)") -> ("error out"=w1008:errorcluster)  [unwired: 8 in, 1 out]
                        n472 = property class="Instr"(reference=w1010, error in=w1008) -> (reference out=w1009:refnum<visa-resource-name>, error out=w1007:errorcluster, "Serial Settings:Number of Bytes at Serial Port"=w1006:u32)
                        n473 = VISA Read(VISA resource name=w1009, byte count=w1006, error in (no error)=w1007) -> (read buffer=w1004:string, error out=w1012:errorcluster)  [unwired: 2 out]
                        n474 = case shown="2" w1001 {
                          tunnel: w1004 -> [_ w1014 w1015]
                          frame Default {
                          }
                          frame 1 {
                            n475 = local write "Read buffer LeCroy 1"(w1014) -> ()
                          }
                          frame 2 {
                            n476 = local write "Read buffer LeCroy 2"(w1015) -> ()
                          }
                        }
                      }
                      frame 0 {
                        n477 = VISA Write(VISA resource name=w1020, write buffer=w1018) -> (VISA resource name out=w1017:refnum<visa-resource-name>, error out=w1016:errorcluster)  [unwired: 1 in, 1 out]
                        n478 = call "read caen.vi"("VISA in"=w1017, "error in"=w1016) -> ("error out"=w1019:errorcluster)  [unwired: 8 in, 5 out]
                      }
                    }
                  }
                  frame True {
                  }
                }
              }
              event "Read Crate Page": Value Change {
                n479 = event-data() -> ("NewVal"=w1060:i32)  [unwired: 1 in]
                n480 = local read "Crate"() -> (w1058:i32)
                n481 = Greater?(x=3, y=w1060) -> (0:w1062:bool)
                n482 = case shown="True" w1062 {
                  tunnel: w1064 -> [_ w1079]
                  tunnel: [w1067 w1078] -> w1063
                  tunnel: "Lock Page" -> [_ w1073]
                  tunnel: w1060 -> [w1066 w1076]
                  tunnel: w1058 -> [_ w1077]
                  frame False {
                    # "Invalid crate number"
                    n483 = Format Into String(format string="Request to read page from crate out of range: %d" ("source"), w1066) -> (resulting string=w1071:string, error out=w1069:errorcluster)  [unwired: 2 in]
                    n484 = Bundle By Name(cluster=errorcluster {"status"=TRUE, "code"=0, "source"=""} ("error out"), "code"=w1066, "source"=w1071) -> (w1068:errorcluster)
                    n485 = Merge Errors(w1068, w1069) -> (w1067:errorcluster)
                  }
                  frame True {
                    # "Crate number is valid"
                    n486 = Equal?(x=w1076, y=w1077) -> (x = y?=w1074:bool)
                    n487 = And(x=w1074, y=w1073) -> (x .and. y?=w1075:bool)
                    n488 = case shown="False" w1075 {
                      tunnel: w1079 -> [w1082 _]
                      tunnel: [w1081 w1120] -> w1078
                      tunnel: w1076 -> [w1080 w1119]
                      frame False {
                        # "cycle through pages"
                        n489 = case shown="0" w1080 {
                          selector: w1080 -> [_ w1093 w1106 w1116]
                          tunnel: w1082 -> [w1085 _ _ _]
                          tunnel: [w1086 w1099 w1112 w1117] -> w1081
                          frame 0 {
                            # "read CAEN page"
                            # "Otherwise, scan through all active channels. \nIncrement shift register to read next page\non next execution."
                            n490 = feedback #2() -> (w1083:i32)  [unwired: 1 in]
                            n491 = Increment(x=w1083) -> (x+1=w1087:i32)
                            n492 = Less?(x=w1087, y=w1085) -> (x < y?=w1088:bool)
                            n493 = Select(t=w1087, s=w1088, f=0 ("t")) -> (s? t:f=w1084:i32)
                            n494 = feedback-in #2(w1084) -> ()
                            n495 = property on="Do Caen Page Read" class="DigNum (strict)"("Val(Sgnl)"=w1083) -> (error out=w1086:errorcluster)  [unwired: 2 in, 1 out]
                          }
                          frame 1 {
                            # "num pages of channels\non this crate"
                            n496 = global read "CAEN globals.vi" "Crate Maps"() -> (w1095:refnum<vi>)
                            n497 = property class="Arr (strict)"(reference=w1095) -> (error out=w1091:errorcluster, "Value"=w1094:T9[])  [unwired: 1 in, 1 out]
                            n498 = Index Array(array=w1094, index=w1093) -> (element=w1096:T9)
                            n499 = Unbundle By Name(w1096) -> ("Total Channels"=w1092:i32)
                            n500 = expression code="ceil((x+1)/16)-1"(w1092) -> (w1090:i32)
                            n501 = feedback #3() -> (w1097:i32)  [unwired: 1 in]
                            n502 = Increment(x=w1097) -> (x+1=w1100:i32)
                            n503 = Less?(x=w1100, y=w1090) -> (x < y?=w1101:bool)
                            n504 = Select(t=w1100, s=w1101, f=0 ("t")) -> (s? t:f=w1098:i32)
                            n505 = feedback-in #3(w1098) -> ()
                            n506 = property on="Do L1 Page Read" class="DigNum (strict)"(error in=w1091, "Val(Sgnl)"=w1097) -> (error out=w1099:errorcluster)  [unwired: 1 in, 1 out]
                          }
                          frame 2 {
                            # "num pages of channels\non this crate"
                            n507 = global read "CAEN globals.vi" "Crate Maps"() -> (w1108:refnum<vi>)
                            n508 = property class="Arr (strict)"(reference=w1108) -> (error out=w1104:errorcluster, "Value"=w1107:T9[])  [unwired: 1 in, 1 out]
                            n509 = Index Array(array=w1107, index=w1106) -> (element=w1109:T9)
                            n510 = Unbundle By Name(w1109) -> ("Total Channels"=w1105:i32)
                            n511 = expression code="ceil((x+1)/16)-1"(w1105) -> (w1103:i32)
                            n512 = feedback #4() -> (w1110:i32)  [unwired: 1 in]
                            n513 = Increment(x=w1110) -> (x+1=w1113:i32)
                            n514 = Less?(x=w1113, y=w1103) -> (x < y?=w1114:bool)
                            n515 = Select(t=w1113, s=w1114, f=0 ("t")) -> (s? t:f=w1111:i32)
                            n516 = feedback-in #4(w1111) -> ()
                            n517 = property on="Do L2 Page Read" class="DigNum (strict)"(error in=w1104, "Val(Sgnl)"=w1110) -> (error out=w1112:errorcluster)  [unwired: 1 in, 1 out]
                          }
                          frame Default {
                            n518 = Bundle By Name(cluster=errorcluster {"status"=TRUE, "code"=0, "source"="Read Crate Page: Invalid Crate Number"} ("error out"), "code"=w1116) -> (w1117:errorcluster)
                          }
                        }
                      }
                      frame True {
                        # "Reading fixed page based on channel selected on monitoring page"
                        n519 = local read "Channel"() -> (w1125:i32)
                        n520 = local read "Card"() -> (w1124:i32)
                        n521 = call "convert rel chan num.vi"("Card"=w1124, "Channel"=w1125, "Crate"=w1119) -> ("error out"=w1123:errorcluster, "Crate index"=w1121:i32, "ACTIVE index"=w1122:i32)  [unwired: 5 in, 1 out]
                        n522 = case shown="0" w1119 {
                          selector: w1119 -> [_ _ _ w1138]
                          tunnel: w1123 -> [w1126 w1131 w1135 _]
                          tunnel: w1122 -> [w1128 _ _ _]
                          tunnel: w1121 -> [_ w1133 w1137 _]
                          tunnel: [w1127 w1130 w1134 w1139] -> w1120
                          frame 0 {
                            # "read caen page based on which page in ACTIVE"
                            n523 = expression code="ceil((x+1)/16)-1"(w1128) -> (w1129:i32)
                            n524 = property on="Do Caen Page Read" class="DigNum (strict)"(error in=w1126, "Val(Sgnl)"=w1129) -> (error out=w1127:errorcluster)  [unwired: 1 in, 1 out]
                          }
                          frame 1 {
                            # "Read lecroy page based on index in crate\n(lecroys cannot hide inactive channels)"
                            n525 = expression code="ceil((x+1)/16)-1"(w1133) -> (w1132:i32)
                            n526 = property on="Do L1 Page Read" class="DigNum (strict)"(error in=w1131, "Val(Sgnl)"=w1132) -> (error out=w1130:errorcluster)  [unwired: 1 in, 1 out]
                          }
                          frame 2 {
                            # "Read lecroy page based on index in crate\n(lecroys cannot hide inactive channels)"
                            n527 = expression code="ceil((x+1)/16)-1"(w1137) -> (w1136:i32)
                            n528 = property on="Do L2 Page Read" class="DigNum (strict)"(error in=w1135, "Val(Sgnl)"=w1136) -> (error out=w1134:errorcluster)  [unwired: 1 in, 1 out]
                          }
                          frame Default {
                            n529 = Bundle By Name(cluster=errorcluster {"status"=TRUE, "code"=0, "source"="Read Crate Page: Invalid Crate Number"} ("error out"), "code"=w1138) -> (w1139:errorcluster)
                          }
                        }
                      }
                    }
                  }
                }
              }
              event "Shifter Notes": Value Change {
                w1145 = "Updating shifter notes" ("string")
                n530 = event-data() -> ()  [unwired: 1 in, 2 out]
                n531 = Write to Text File(file (use dialog)=path "C:/Users/ANNIE/Documents/Logs/Shifter_Notes.txt", text="Shifter Notes") -> (refnum out=w1147:refnum<file>, error out=w1148:errorcluster)  [unwired: 2 in, 1 out]
                n532 = Close File(refnum=w1147, error in=w1148) -> (error out=w1143:errorcluster)  [unwired: 1 out]
                n533 = call "Append to display log.vi"("string"=w1145) -> ("error out"=w1146:errorcluster)  [unwired: 10 in]
                n534 = call "Append to event log.vi"("string"=w1145) -> ("error out"=w1144:errorcluster)  [unwired: 10 in]
                n535 = call <vilib>:"Clear Errors.vi"("error in (no error)"=w1146) -> ()  [unwired: 5 in, 2 out]
                n536 = Merge Errors(w1143, w1144) -> (w1142:errorcluster)
              }
              event "Update Plots & Alarms": Value Change {
                n537 = event-data() -> ("NewVal"=w1162:T2)  [unwired: 1 in]
                n538 = global read "CAEN globals.vi" "TimeStamp History"() -> (w1160:dbl[][])
                n539 = global read "CAEN globals.vi" "Vmon History"() -> (w1156:dbl[][])
                n540 = global read "CAEN globals.vi" "Imon History"() -> (w1158:dbl[][])
                n541 = global read "CAEN globals.vi" "Vset History"() -> (w1157:dbl[][])
                n542 = global read "CAEN globals.vi" "Iset History"() -> (w1159:dbl[][])
                n543 = Unbundle By Name(w1162) -> ("Num Channels Read"=w1161:i32, "Start Index"=w1151:i32)
                n544 = call "active_index_to_crate_card_chan.vi"("Channels in Active"=w1153, "Index"=w1151) -> ("Crate"=w1152:i32)  [unwired: 7 in, 2 out]
                n545 = Get Date/Time String(want seconds? (F)=TRUE) -> (date string=w1175:string, time string=w1174:string)  [unwired: 2 in]
                n546 = call <vilib>:"Space Constant.vi"() -> ("String"=w1173:string)
                n547 = call "convert rel chan num.vi"("Card"="Card", "Channel"="Channel", "Crate"="Crate") -> ("ACTIVE index"=w1168:i32)  [unwired: 5 in, 3 out]
                n548 = Concatenate Strings(w1175, w1173, w1174) -> (w1171:string)
                n549 = call "form alarm string.vi"("Vmon"=w1156, "Vset"=w1157, "Imon"=w1158, "Iset"=w1159, "Timestamps"=w1160, "Start index"=w1151, "Crate"=w1152, "Num Channels Read"=w1161) -> ("Alarm String"=w1181:string, "Background colour"=w1189:u32, "All alarms string"=w1167:string, "Alarm Array"=w1188:string[][], "Alarm"=w1182:bool, "error out"=w1163:errorcluster)  [unwired: 6 in]
                "Alarm status" <- w1167
                n550 = local write "Timestamp"(w1171) -> ()
                n551 = Transpose 2D Array(2D array=w1158) -> (transposed array=w1184:dbl[][])
                n552 = Transpose 2D Array(2D array=w1160) -> (transposed array=w1185:dbl[][])
                n553 = call "extract channel history.vi"("Vmon Hist in"=w1156, "Vset Hist in"=w1157, "Imon Hist in"=w1158, "Iset Hist in"=w1159, "TS History"=w1160, "index"=w1168) -> ("Voltage"=→"Voltage":cluster{dbl[], dbl[]}[], "Current"=→"Current":cluster{dbl[], dbl[]}[])  [unwired: 8 in, 4 out]
                n554 = Transpose 2D Array(2D array=w1160) -> (transposed array=w1186:dbl[][])
                n555 = Transpose 2D Array(2D array=w1156) -> (transposed array=w1187:dbl[][])
                n556 = call "Append to display log.vi"("string"="Updating plots & alarms") -> ("error out"=w1180:errorcluster)  [unwired: 10 in]
                n557 = call "trim history.vi"("Values"=w1184, "Timestamps"=w1185) -> ("Array 3"=→"Currents":cluster{dbl[], dbl[]}[])  [unwired: 13 in]
                n558 = call <vilib>:"Clear Errors.vi"("error in (no error)"=w1180) -> ()  [unwired: 5 in, 2 out]
                n559 = call "trim history.vi"("Values"=w1187, "Timestamps"=w1186) -> ("Array 3"=→"Voltages":cluster{dbl[], dbl[]}[])  [unwired: 13 in]
                n560 = case shown="Default" w1167 {
                  tunnel: w1189 -> [_ w1220]
                  tunnel: [_ w1219] -> w1165
                  tunnel: w1188 -> [_ w1198]
                  tunnel: w1182 -> [_ w1218]
                  tunnel: w1181 -> [_ w1217]
                  tunnel: [_ w1211] -> w1164
                  tunnel: "Crate" -> [_ w1208]
                  tunnel: [_ w1194] -> w1155
                  frame "" {
                    # "No errors or alarms"
                  }
                  frame Default {
                    # "this array has already \nlogged errors removed"
                    n561 = property on="summary status" class="Str"("Value"=w1217, "Text.BGColor"=w1220, "Blinking"=w1218) -> (error out=w1210:errorcluster)  [unwired: 2 in, 1 out]
                    n562 = local read "slack"() -> (w1197:T1)
                    n563 = local read "Current Event Log"() -> (w1216:path)
                    n564 = call <vilib>:"Acquire Semaphore.vi"("ms timeout (-1)"=5000, "semaphore"=w1197) -> ("error out"=w1192:errorcluster, "timed out"=w1191:bool, "semaphore out"=w1195:T1)  [unwired: 3 in]
                    n565 = property on="Status message" class="Str"(error in=w1210, "Value"=w1217, "Blinking"=w1218) -> (error out=w1209:errorcluster)  [unwired: 1 in, 1 out]
                    n566 = Or(x=w1191, y=w1192) -> (x .or. y?=w1193:bool)
                    n567 = Empty Array?(array=w1198) -> (empty?=w1199:bool)
                    n568 = case shown="False" w1193 {
                      tunnel: w1198 -> [w1224 _]
                      tunnel: w1195 -> [w1222 _]
                      tunnel: [w1221 w1238] -> w1194
                      tunnel: w1192 -> [_ w1239]
                      tunnel: w1191 -> [_ w1235]
                      frame False {
                        n569 = flat-sequence {
                          tunnel: w1224 -> [w1229]
                          tunnel: [w1226] -> w1223
                          tunnel: w1222 -> [w1226]
                          tunnel: w1223 -> [w1233]
                          tunnel: [w1232] -> w1221
                          frame #0 {
                            n570 = local read "New Errors"() -> (w1228:string)
                            n571 = Array To Spreadsheet String(delimiter (Tab)=",", array=w1229, 3:"%s" ("delimiter (Tab)")) -> (spreadsheet string=w1230:string)
                            n572 = Concatenate Strings(w1230, w1228) -> (w1227:string)
                            n573 = local write "New Errors"(w1227) -> ()
                          }
                          frame #1 {
                            n574 = call <vilib>:"Release Semaphore.vi"("semaphore"=w1233) -> ("error out"=w1232:errorcluster)  [unwired: 5 in, 1 out]
                          }
                        }
                      }
                      frame True {
                        # "timeout does not generate an error:\nmake one manually"
                        n575 = Select(t=errorcluster {"status"=TRUE, "code"=0, "source"="Timed out obtaining semaphore for writing new messages to slack buffer!\nErrors will NOT be sent to slack!!"} ("error out"), s=w1235, f=errorcluster {"status"=FALSE, "code"=0, "source"=""}) -> (s? t:f=w1234:errorcluster)
                        n576 = Merge Errors(w1239, w1234) -> (w1238:errorcluster)
                      }
                    }
                    n577 = call <vilib>:"Check if File or Folder Exists.vi"("path"=w1216) -> ("error out"=w1213:errorcluster, "file or folder exists?"=w1215:bool, "dup path"=w1214:path)  [unwired: 8 in]
                    n578 = case shown="False" w1199 {
                      tunnel: [w1242 w1251] -> w1211
                      tunnel: w1209 -> [w1241 w1251]
                      tunnel: w1208 -> [w1240 _]
                      frame False {
                        n579 = case shown="0" w1240 {
                          tunnel: [w1243 w1250] -> w1242
                          tunnel: w1241 -> [w1243 w1249]
                          frame Default {
                            # "Only take a screenshot for the CAEN"
                          }
                          frame 0 {
                            n580 = local read "Display String"() -> (w1246:string)
                            n581 = Search and Replace String(replace all?=TRUE ("want seconds? (F)"), input string=w1246, search string="\t", error in=w1249) -> (result string=w1247:string, error out=w1248:errorcluster)  [unwired: 4 in, 2 out]
                            n582 = property on="Alarm Screencap" class="Str"(error in=w1248, "Val(Sgnl)"=w1247) -> (error out=w1250:errorcluster)  [unwired: 1 in, 1 out]
                          }
                        }
                      }
                      frame True {
                      }
                    }
                    n583 = case shown="False" w1215 {
                      tunnel: w1214 -> [w1255 w1258]
                      tunnel: [w1253 w1257] -> w1203
                      tunnel: w1213 -> [w1256 w1257]
                      tunnel: [w1254 w1258] -> w1202
                      tunnel: string[] ["Timestamp", "Type", "Info"] ("subarray") -> [w1252 _]
                      frame False {
                        n584 = call-poly <vilib>:"Write Delimited Spreadsheet.vi"("file path (dialog if empty)"=w1255, "1D data"=w1252, "error in (no error)"=w1256) -> ("new file path (Not A Path if cancelled)"=w1254:path, "error out"=w1253:errorcluster)  [unwired: 11 in]
                      }
                      frame True {
                      }
                    }
                    n585 = local read "Event Log"() -> (w1200:string[][])
                    n586 = Build Array (concatenate)(w1200, w1198) -> (w1205:string[][])
                    n587 = Delete From Array(array=w1205, length=100) -> (deleted portion=→"Event Log":string[][])  [unwired: 2 in, 1 out]
                    n588 = call-poly <vilib>:"Write Delimited Spreadsheet.vi"("file path (dialog if empty)"=w1202, "2D data"=w1198, "append to file? (new file:F)"=TRUE ("append to file? (F)"), "error in (no error)"=w1203, "delimiter (\\t)"="," ("delimiter (\\t)")) -> ("error out"=w1219:errorcluster)  [unwired: 9 in, 1 out]
                  }
                }
                n589 = Merge Errors(w1164, w1165, w1163, w1155) -> (w1166:errorcluster)
              }
              event "read error": Value Change {
                n590 = event-data() -> ("NewVal"=w1262:cluster{"Crate":i32, "error out":errorcluster})  [unwired: 1 in, 1 out]
                n591 = Unbundle(w1262) -> ("Crate"=w1260:i32, "error out"=w1261:errorcluster)
                n592 = case shown="Error" w1261 {
                  selector: w1261 -> [_ w1304]
                  tunnel: w1260 -> [_ w1282]
                  tunnel: [_ w1286] -> w1259
                  frame No Error {
                  }
                  frame Error {
                    w1303 = TRUE ("Alarm")
                    n593 = Unbundle By Name(w1304) -> ("source"=w1279:string)
                    n594 = Get Date/Time String(want seconds? (F)=TRUE) -> (date string=w1278:string, time string=w1277:string)  [unwired: 2 in]
                    n595 = call <vilib>:"Space Constant.vi"() -> ("String"=w1276:string)
                    n596 = Concatenate Strings(w1278, w1276, w1277) -> (w1274:string)
                    n597 = call "Append to display log.vi"("string"="Logging Read Error") -> ("error out"=w1305:errorcluster)  [unwired: 10 in]
                    n598 = Format Into String(format string="Crate %d Error: %s" ("stripped output"), w1282, w1279) -> (resulting string=w1281:string, error out=w1280:errorcluster)  [unwired: 2 in]
                    n599 = Build Array(w1274, "Read Error" ("stripped output"), w1279) -> (w1272:string[])
                    n600 = call <vilib>:"Clear Errors.vi"("error in (no error)"=w1305) -> ()  [unwired: 5 in, 2 out]
                    n601 = Build Array(w1272) -> (w1265:string[][])
                    n602 = property on="summary status" class="Str"(error in=w1280, "Value"=w1281, "Text.BGColor"=u32 16711680, "Blinking"=w1303) -> (error out=w1296:errorcluster)  [unwired: 1 in, 1 out]
                    n603 = local write "Alarm status"(w1281) -> ()
                    n604 = local read "Current Event Log"() -> (w1301:path)
                    n605 = local read "slack"() -> (w1271:T1)
                    n606 = call <vilib>:"Acquire Semaphore.vi"("ms timeout (-1)"=5000, "semaphore"=w1271) -> ("error out"=w1264:errorcluster, "timed out"=w1267:bool, "semaphore out"=w1269:T1)  [unwired: 3 in]
                    n607 = property on="Status message" class="Str"(error in=w1296, "Value"=w1281, "Blinking"=w1303) -> (error out=w1295:errorcluster)  [unwired: 1 in, 1 out]
                    n608 = Or(x=w1267, y=w1264) -> (x .or. y?=w1268:bool)
                    n609 = call <vilib>:"Check if File or Folder Exists.vi"("path"=w1301) -> ("error out"=w1298:errorcluster, "file or folder exists?"=w1300:bool, "dup path"=w1299:path)  [unwired: 8 in]
                    n610 = case shown="False" w1268 {
                      tunnel: w1265 -> [w1310 _]
                      tunnel: w1269 -> [w1308 _]
                      tunnel: [w1307 w1324] -> w1266
                      tunnel: w1264 -> [_ w1325]
                      tunnel: w1267 -> [_ w1321]
                      frame False {
                        n611 = flat-sequence {
                          tunnel: w1310 -> [w1315]
                          tunnel: [w1312] -> w1309
                          tunnel: w1308 -> [w1312]
                          tunnel: w1309 -> [w1319]
                          tunnel: [w1318] -> w1307
                          frame #0 {
                            n612 = local read "New Errors"() -> (w1314:string)
                            n613 = Array To Spreadsheet String(delimiter (Tab)=",", array=w1315, 3:"%s" ("delimiter (Tab)")) -> (spreadsheet string=w1316:string)
                            n614 = Concatenate Strings(w1316, w1314) -> (w1313:string)
                            n615 = local write "New Errors"(w1313) -> ()
                          }
                          frame #1 {
                            n616 = call <vilib>:"Release Semaphore.vi"("semaphore"=w1319) -> ("error out"=w1318:errorcluster)  [unwired: 5 in, 1 out]
                          }
                        }
                      }
                      frame True {
                        # "timeout does not generate an error:\nmake one manually"
                        n617 = Select(t=errorcluster {"status"=TRUE, "code"=0, "source"="Timed out obtaining semaphore for writing new messages to slack buffer!\nErrors will NOT be sent to slack!!"} ("error out"), s=w1321, f=errorcluster {"status"=FALSE, "code"=0, "source"=""}) -> (s? t:f=w1320:errorcluster)
                        n618 = Merge Errors(w1325, w1320) -> (w1324:errorcluster)
                      }
                    }
                    n619 = case shown="0" w1282 {
                      tunnel: [w1333 w1340] -> w1285
                      tunnel: w1295 -> [w1333 w1339]
                      frame Default {
                        # "Only take a screenshot for the CAEN"
                      }
                      frame 0 {
                        n620 = local read "Display String"() -> (w1336:string)
                        n621 = Search and Replace String(replace all?=TRUE ("want seconds? (F)"), input string=w1336, search string="\t", error in=w1339) -> (result string=w1337:string, error out=w1338:errorcluster)  [unwired: 4 in, 2 out]
                        n622 = property on="Alarm Screencap" class="Str"(error in=w1338, "Val(Sgnl)"=w1337) -> (error out=w1340:errorcluster)  [unwired: 1 in, 1 out]
                      }
                    }
                    n623 = local read "Event Log"() -> (w1288:string[][])
                    n624 = case shown="False" w1300 {
                      tunnel: w1299 -> [w1329 w1332]
                      tunnel: [w1327 w1331] -> w1290
                      tunnel: w1298 -> [w1330 w1331]
                      tunnel: [w1328 w1332] -> w1289
                      tunnel: string[] ["Timestamp", "Type", "Info"] ("subarray") -> [w1326 _]
                      frame False {
                        n625 = call-poly <vilib>:"Write Delimited Spreadsheet.vi"("file path (dialog if empty)"=w1329, "1D data"=w1326, "error in (no error)"=w1330) -> ("new file path (Not A Path if cancelled)"=w1328:path, "error out"=w1327:errorcluster)  [unwired: 11 in]
                      }
                      frame True {
                      }
                    }
                    n626 = Build Array (concatenate)(w1288, w1265) -> (w1292:string[][])
                    n627 = Delete From Array(array=w1292, length=100) -> (deleted portion=w1287:string[][])  [unwired: 2 in, 1 out]
                    n628 = call-poly <vilib>:"Write Delimited Spreadsheet.vi"("file path (dialog if empty)"=w1289, "2D data"=w1265, "append to file? (new file:F)"=TRUE ("append to file? (F)"), "error in (no error)"=w1290, "delimiter (\\t)"="," ("delimiter (\\t)")) -> ("error out"=w1284:errorcluster)  [unwired: 9 in, 1 out]
                    n629 = local write "Event Log"(w1287) -> ()
                    n630 = Merge Errors(w1285, w1284, w1266) -> (w1286:errorcluster)
                  }
                }
              }
              event "slack error": Value Change {
                n631 = event-data() -> ("NewVal"=w1341:string)  [unwired: 1 in]
                n632 = case shown="Default" w1341 {
                  selector: w1341 -> [_ w1346]
                  tunnel: [_ w1344] -> w1342
                  frame "" {
                  }
                  frame Default {
                    w1370 = TRUE ("Alarm")
                    # "if we couldn't send the messages to slack\nwipe the new errors variable\notherwise if it keeps happening\nwe'll never flush the new errors variable\nand it'll just keep growing"
                    n633 = Get Date/Time String(want seconds? (F)=TRUE) -> (date string=w1354:string, time string=w1353:string)  [unwired: 2 in]
                    n634 = call <vilib>:"Space Constant.vi"() -> ("String"=w1352:string)
                    n635 = Concatenate Strings(w1354, w1352, w1353) -> (w1350:string)
                    n636 = call "Append to display log.vi"("string"="Logging Slack Error") -> ("error out"=w1371:errorcluster)  [unwired: 10 in]
                    n637 = Build Array(w1350, "Slack Error" ("stripped output"), w1346) -> (w1348:string[])
                    n638 = call <vilib>:"Clear Errors.vi"("error in (no error)"=w1371) -> ()  [unwired: 5 in, 2 out]
                    n639 = Build Array(w1348) -> (w1347:string[][])
                    n640 = property on="summary status" class="Str"("Value"=w1346, "Text.BGColor"=u32 16711680, "Blinking"=w1370) -> (error out=w1363:errorcluster)  [unwired: 2 in, 1 out]
                    n641 = local write "Alarm status"(w1346) -> ()
                    n642 = local read "Current Event Log"() -> (w1368:path)
                    n643 = property on="Status message" class="Str"(error in=w1363, "Value"=w1346, "Blinking"=w1370) -> ()  [unwired: 1 in, 2 out]
                    n644 = call <vilib>:"Check if File or Folder Exists.vi"("path"=w1368) -> ("error out"=w1365:errorcluster, "file or folder exists?"=w1367:bool, "dup path"=w1366:path)  [unwired: 8 in]
                    n645 = local read "Event Log"() -> (w1356:string[][])
                    n646 = case shown="False" w1367 {
                      tunnel: w1366 -> [w1376 w1379]
                      tunnel: [w1374 w1378] -> w1358
                      tunnel: w1365 -> [w1377 w1378]
                      tunnel: [w1375 w1379] -> w1357
                      tunnel: string[] ["Timestamp", "Type", "Info"] ("subarray") -> [w1373 _]
                      frame False {
                        n647 = call-poly <vilib>:"Write Delimited Spreadsheet.vi"("file path (dialog if empty)"=w1376, "1D data"=w1373, "error in (no error)"=w1377) -> ("new file path (Not A Path if cancelled)"=w1375:path, "error out"=w1374:errorcluster)  [unwired: 11 in]
                      }
                      frame True {
                      }
                    }
                    n648 = local write "New Errors"("") -> ()
                    n649 = Build Array (concatenate)(w1356, w1347) -> (w1360:string[][])
                    n650 = Delete From Array(array=w1360, length=100) -> (deleted portion=w1355:string[][])  [unwired: 2 in, 1 out]
                    n651 = call-poly <vilib>:"Write Delimited Spreadsheet.vi"("file path (dialog if empty)"=w1357, "2D data"=w1347, "append to file? (new file:F)"=TRUE ("append to file? (F)"), "error in (no error)"=w1358, "delimiter (\\t)"="," ("delimiter (\\t)")) -> ("error out"=w1344:errorcluster)  [unwired: 9 in, 1 out]
                    n652 = local write "Event Log"(w1355) -> ()
                  }
                }
              }
              event "Alarm Screencap": Value Change {
                w1389 = TRUE ("want seconds? (F)")
                n653 = event-data() -> ("NewVal"=→"Alarm Screencap":string)  [unwired: 1 in]
                n654 = local read "Current Error Log"() -> (w1419:path)
                n655 = local read "Display"() -> (w1417:string[][])
                n656 = Get File Size(file=w1419) -> (refnum out=w1390:refnum<file>, size (in bytes)=w1394:i64, 0:w1393:errorcluster)  [unwired: 1 in]
                n657 = Array To Spreadsheet String(delimiter (Tab)=",", array=w1417, 3:"%s" ("delimiter (Tab)")) -> (spreadsheet string=w1388:string)
                n658 = Close File(refnum=w1390, error in=w1393) -> (path=w1391:path, error out=w1392:errorcluster)
                n659 = global read "CAEN globals.vi" "Selection Position"() -> (w1410:cluster{i32, i32})
                n660 = case shown="0" w1394 {
                  tunnel: [w1426 w1429] -> w1420
                  tunnel: [w1425 w1428] -> w1421
                  tunnel: w1392 -> [w1424 w1428]
                  tunnel: w1391 -> [w1423 w1429]
                  frame 0 {
                    # "write headers if \nthis is a new file"
                    n661 = call-poly <vilib>:"Write Delimited Spreadsheet.vi"("file path (dialog if empty)"=w1423, "1D data"=string[] ["Timestamp", "Error Code", "Error Source", "Display at Time of Error", "Selection Position"] ("subarray"), "error in (no error)"=w1424) -> ("new file path (Not A Path if cancelled)"=w1426:path, "error out"=w1425:errorcluster)  [unwired: 11 in]
                  }
                  frame Default {
                  }
                }
                n662 = local read "Event Log"() -> (w1385:string[][])
                n663 = Search and Replace String(replace all?=w1389, input string=w1388, search string="\n" ("input string"), replace string="\\n" ("input string")) -> (result string=w1406:string, error out=w1405:errorcluster)  [unwired: 4 in, 2 out]
                n664 = Search and Replace String(replace all?=w1389, input string=w1406, search string="\t" ("input string"), replace string="\\t" ("input string"), error in=w1405) -> (result string=w1400:string, error out=w1402:errorcluster)  [unwired: 3 in, 2 out]
                n665 = local read "Alarm status"() -> (w1387:string)
                n666 = Unbundle(w1410) -> (w1409:i32, w1408:i32)
                n667 = Delete From Array(array=w1385) -> (deleted portion=w1384:string[])  [unwired: 3 in, 1 out]
                n668 = Search and Replace String(replace all?=w1389, input string=w1400, search string="\r" ("input string"), replace string="\\r" ("input string"), error in=w1402) -> (result string=w1401:string, error out=w1396:errorcluster)  [unwired: 3 in, 2 out]
                n669 = Index Array(array=w1384) -> (element=w1380:string)  [unwired: 1 in]
                "Screencap Timestamp" <- w1380
                n670 = Number To Decimal String(number=-1) -> (decimal integer string=w1414:string)  [unwired: 1 in]
                n671 = Format Into String(w1409, w1408) -> (resulting string=w1407:string, error out=w1397:errorcluster)  [unwired: 3 in]
                n672 = call <vilib>:"Trim Whitespace.vi"("string"=w1401) -> ("trimmed string"=w1415:string)  [unwired: 1 in]
                n673 = Merge Errors(w1396, w1397) -> (w1395:errorcluster)
                n674 = Build Array(w1380, w1414, w1387, w1415, w1407) -> (w1418:string[])
                n675 = call <vilib>:"Find First Error.vi"("error in (no error)"=w1395) -> ()  [unwired: 3 in, 2 out]
                n676 = call-poly <vilib>:"Write Delimited Spreadsheet.vi"("file path (dialog if empty)"=w1420, "1D data"=w1418, "append to file? (new file:F)"=TRUE ("append to file? (F)"), "error in (no error)"=w1421) -> ("error out"=w1382:errorcluster)  [unwired: 10 in, 1 out]
              }
              event "Card", "Channel", "Index", "Crate": Value Change {
                n677 = event-data() -> ("CtlRef"=w1439:refnum<vi>)  [unwired: 1 in]
                n678 = control-ref of="Index"() -> (w1440:refnum<vi>)
                n679 = Equal?(x=w1440, y=w1439) -> (x = y?=w1438:bool)
                n680 = case shown="True" w1438 {
                  tunnel: w1436 -> [_ w1449]
                  tunnel: [w1445 "Index"] -> w1437
                  tunnel: [w1444 _] -> w1435
                  frame False {
                    n681 = local read "Channel"() -> (w1447:i32)
                    n682 = local read "Crate"() -> (w1448:i32)
                    n683 = local read "Card"() -> (w1446:i32)
                    n684 = call "convert rel chan num.vi"("Card"=w1446, "Channel"=w1447, "Crate"=w1448) -> ("error out"=w1444:errorcluster, "ACTIVE index"=w1445:i32)  [unwired: 5 in, 2 out]
                    n685 = local write "Index"(w1445) -> ()
                  }
                  frame True {
                    n686 = call "active_index_to_crate_card_chan.vi"("Channels in Active"=w1449, "Index"="Index") -> ("Card"=w1452:i32, "Channel"=w1451:i32, "Crate"=w1450:i32)  [unwired: 7 in]
                    n687 = local write "Channel"(w1451) -> ()
                    n688 = local write "Card"(w1452) -> ()
                    n689 = local write "Crate"(w1450) -> ()
                  }
                }
                n690 = global read "CAEN globals.vi" "TimeStamp History"() -> (w1430:dbl[][])
                n691 = global read "CAEN globals.vi" "Vmon History"() -> (w1433:dbl[][])
                n692 = global read "CAEN globals.vi" "Imon History"() -> (w1434:dbl[][])
                n693 = global read "CAEN globals.vi" "Vset History"() -> (w1432:dbl[][])
                n694 = global read "CAEN globals.vi" "Iset History"() -> (w1431:dbl[][])
                n695 = call "extract channel history.vi"("Vmon Hist in"=w1433, "Vset Hist in"=w1432, "Imon Hist in"=w1434, "Iset Hist in"=w1431, "TS History"=w1430, "index"=w1437) -> ("Voltage"=w1443:cluster{dbl[], dbl[]}[], "Current"=w1442:cluster{dbl[], dbl[]}[])  [unwired: 8 in, 4 out]
                n696 = local write "Voltage"(w1443) -> ()
                n697 = local write "Current"(w1442) -> ()
              }
              event "Start New Run": Value Change {
                w1472 = T20[] [enum."Event", enum."Channel", enum."Program", enum."ZMQ"] items=["Event", "ZMQ", "Channel", "Program"]
                n698 = event-data() -> ()  [unwired: 1 in, 1 out]
                n699 = local read "Log Directory"() -> (w1470:path)
                n700 = local write "Start New Run"(FALSE ("Start New Run")) -> ()
                n701 = local read "Subrun"() -> (w1458:i32)
                n702 = local read "Run"() -> (w1459:i32)
                n703 = Format Into String(format string=w1462, w1459, w1458) -> (resulting string=w1461:string, error out=w1460:errorcluster)  [unwired: 2 in]
                n704 = for {
                  tunnel: w1470 -> [w1481]
                  tunnel: w1459 -> [w1480]
                  tunnel: w1458 -> [w1479]
                  tunnel: w1472 -> [w1478] mode=indexing
                  tunnel: [w1477] -> w1471 mode=indexing
                  tunnel: [w1476] -> w1466 mode=indexing
                  n705 = call "Create Log or Log Directory.vi"("Base Directory"=w1481, "Run"=w1480, "Subrun"=w1479, "Append if exists?"=TRUE, "Log Type"=w1478) -> ("Path"=w1477:path, "error out"=w1476:errorcluster)  [unwired: 13 in]
                }
                n706 = Write to Text File(file (use dialog)=w1463, text=w1461, error in=w1460) -> (refnum out=w1455:refnum<file>, error out=w1457:errorcluster)  [unwired: 1 in, 1 out]
                n707 = Close File(refnum=w1455, error in=w1457) -> (error out=w1456:errorcluster)  [unwired: 1 out]
                n708 = Index Array(array=w1471) -> (element #1=w1469:path, element #2=w1468:path, element #3=w1467:path, element #4=w1454:path)  [unwired: 4 in]
                n709 = Merge Errors(w1466, w1456) -> (w1465:errorcluster)
                n710 = global write "CAEN globals.vi" "Current Event Log"(w1469) -> ()
                n711 = local write "Current Event Log"(w1469) -> ()
                n712 = local write "Current Channel Log"(w1468) -> ()
                n713 = local write "Current Error Log"(w1467) -> ()
                n714 = local write "Current ZMQ Log"(w1454) -> ()
              }
              event "Start New Error Log": Value Change {
                w1482 = "starting new error log" ("string")
                n715 = event-data() -> ()  [unwired: 1 in, 1 out]
                n716 = local read "Current Error Log"() -> (w1490:path)
                n717 = local write "Start New Error Log"(FALSE ("Start new Error Log")) -> ()
                n718 = call "Append to display log.vi"("string"=w1482) -> ("error out"=w1491:errorcluster)  [unwired: 10 in]
                n719 = call "Creat new log or directory.vi"("Log"=w1490) -> ("error out"=w1488:errorcluster, "New Log"=w1484:path)  [unwired: 9 in]
                n720 = call <vilib>:"Clear Errors.vi"("error in (no error)"=w1491) -> ()  [unwired: 5 in, 2 out]
                n721 = call <vilib>:"Space Constant.vi"() -> ("String"=w1483:string)
                n722 = Path To String(path=w1484) -> (string=w1485:string)
                n723 = local write "Current Error Log"(w1484) -> ()
                n724 = Concatenate Strings(w1482, w1483, w1485) -> (w1486:string)
                n725 = call "Append to event log.vi"("string"=w1486) -> ("error out"=w1489:errorcluster)  [unwired: 10 in]
                n726 = Merge Errors(w1488, w1489) -> (w1487:errorcluster)
              }
              event "Start New Event Log": Value Change {
                w1495 = "starting new event log" ("string")
                n727 = event-data() -> ()  [unwired: 1 in, 1 out]
                n728 = local write "Start New Event Log"(FALSE ("Start new Error Log")) -> ()
                n729 = local read "Current Event Log"() -> (w1503:path)
                n730 = call "Creat new log or directory.vi"("Log"=w1503) -> ("error out"=w1498:errorcluster, "New Log"=w1496:path)  [unwired: 9 in]
                n731 = call <vilib>:"Space Constant.vi"() -> ("String"=w1499:string)
                n732 = Path To String(path=w1496) -> (string=w1500:string)
                n733 = Concatenate Strings(w1495, w1499, w1500) -> (w1501:string)
                n734 = global write "CAEN globals.vi" "Current Event Log"(w1496) -> ()
                n735 = local write "Current Event Log"(w1496) -> ()
                n736 = call "Append to event log.vi"("string"=w1501) -> ("error out"=w1502:errorcluster)  [unwired: 10 in]
                n737 = call "Append to display log.vi"("string"=w1495) -> ("error out"=w1504:errorcluster)  [unwired: 10 in]
                n738 = call <vilib>:"Clear Errors.vi"("error in (no error)"=w1504) -> ()  [unwired: 5 in, 2 out]
                n739 = Merge Errors(w1498, w1502) -> (w1497:errorcluster)
              }
              event "Start New Channel Log": Value Change {
                w1508 = "Starting new channel log" ("string")
                n740 = event-data() -> ()  [unwired: 1 in, 2 out]
                n741 = local read "Current Channel Log"() -> (w1516:path)
                n742 = local write "Start New Channel Log"(FALSE ("Start new Channel Log")) -> ()
                n743 = call "Creat new log or directory.vi"("Log"=w1516) -> ("error out"=w1510:errorcluster, "New Log"=w1511:path)  [unwired: 9 in]
                n744 = local write "Current Channel Log"(w1511) -> ()
                n745 = call <vilib>:"Space Constant.vi"() -> ("String"=w1512:string)
                n746 = Path To String(path=w1511) -> (string=w1513:string)
                n747 = Concatenate Strings(w1508, w1512, w1513) -> (w1514:string)
                n748 = call "Append to display log.vi"("string"=w1508) -> ("error out"=w1517:errorcluster)  [unwired: 10 in]
                n749 = call "Append to event log.vi"("string"=w1514) -> ("error out"=w1515:errorcluster)  [unwired: 10 in]
                n750 = call <vilib>:"Clear Errors.vi"("error in (no error)"=w1517) -> ()  [unwired: 5 in, 2 out]
                n751 = Merge Errors(w1510, w1515) -> (w1509:errorcluster)
              }
              event "Channel Array": Value Change {
                # "scan through channels and update any with new properties"
                n752 = event-data() -> ("NewVal"=w1525:T8[], "OldVal"=w1524:T8[])  [unwired: 1 in]
                n753 = for {
                  tunnel: w1525 -> [w1531] mode=indexing
                  tunnel: w1524 -> [w1530] mode=indexing
                  tunnel: [w1527] -> w1523
                  i -> [w1528]
                  stop <- w1526 stop-if-true
                  n754 = Not Equal?(x=w1531, y=w1530) -> (x != y?=w1529:bool)
                  n755 = case shown="True" w1529 {
                    tunnel: w1531 -> [_ w1539]
                    tunnel: w1530 -> [_ w1535]
                    tunnel: [_ w1540] -> w1527
                    tunnel: w1528 -> [_ _]
                    tunnel: [_ w1536] -> w1526
                    frame False {
                      # "skip channel if no elements have changed"
                    }
                    frame True {
                      n756 = Unbundle By Name(w1535) -> ("Crate"=w1532:i32, "Card"=w1534:i32, "Channel"=w1533:i32)
                      n757 = call <userlib>:"Cluster to Array of VData__ogtk.vi"("Cluster"=w1539) -> ("Array of VData"=w1538:variant[])  [unwired: 9 in, 1 out]
                      n758 = call <userlib>:"Cluster to Array of VData__ogtk.vi"("Cluster"=w1535) -> ("Array of VData"=w1537:variant[])  [unwired: 9 in, 1 out]
                      n759 = for {
                        tunnel: [w1548] -> w1540
                        tunnel: w1538 -> [w1549] mode=indexing
                        tunnel: w1537 -> [w1546] mode=indexing
                        tunnel: [w1547] -> w1536
                        tunnel: w1534 -> [w1545]
                        tunnel: w1533 -> [w1544]
                        tunnel: w1532 -> [w1541]
                        i -> [w1551]
                        stop <- w1547 stop-if-true
                        n760 = To Double Precision Float(number=w1544) -> (double precision float=w1543:dbl)
                        n761 = Not Equal?(x=w1549, y=w1546) -> (x != y?=w1550:bool)
                        n762 = case shown="True" w1550 {
                          tunnel: [_ w1563] -> w1548
                          tunnel: w1551 -> [_ w1565]
                          tunnel: w1549 -> [_ w1564]
                          tunnel: [_ TRUE ("Value (Signaling)")] -> w1547
                          tunnel: w1545 -> [_ w1558]
                          tunnel: w1543 -> [_ w1560]
                          tunnel: 100.0 ("x") -> [_ w1557]
                          tunnel: w1541 -> [_ w1553]
                          frame False {
                          }
                          frame True {
                            n763 = local write "Value"(w1564) -> ()
                            n764 = Divide(x=w1560, y=w1557) -> (x/y=w1559:dbl)
                            n765 = case shown="13" w1565 {
                              tunnel: [_ _ _ _ _ _ TRUE ("Value (Signaling)")] -> w1562
                              tunnel: [Channel_Properties."Name" ("Property") Channel_Properties."Vset" ("Property") Channel_Properties."Iset" ("Property") Channel_Properties."Enable" ("Property") Channel_Properties."Vswmax" ("Property") Channel_Properties."Flag" ("Property") w1574] -> w1556
                              frame 0 {
                              }
                              frame 7 {
                              }
                              frame 9 {
                              }
                              frame 11 {
                              }
                              frame 13 {
                              }
                              frame 14 {
                              }
                              frame 1..6, 8, 10, 12, Default {
                                n766 = local read "Property"() -> (w1574:T4)
                              }
                            }
                            n767 = Add(x=w1558, y=w1559) -> (x+y=w1552:dbl)
                            n768 = Bundle By Name(cluster=T3 {" Card.Channel"=1.12, "Crate"=0} ("Set Card.Channel"), "Crate"=w1553, "Card.Channel"=w1552) -> (w1554:T3)
                            n769 = local write "Property"(w1556) -> ()
                            n770 = case shown="True" w1562 {
                              tunnel: [w1566 _] -> w1563
                              frame False {
                                n771 = property on="Set channel property" class="Bool (strict)"("Val(Sgnl)"=TRUE ("Value (Signaling)")) -> (error out=w1566:errorcluster)  [unwired: 2 in, 1 out]
                              }
                              frame True {
                                # "read-only column or unrecognised property"
                              }
                            }
                            n772 = local write "Set Card.Channel"(w1554) -> ()
                          }
                        }
                      }
                    }
                  }
                }
              }
              event "Set channel property": Value Change {
                n773 = event-data() -> ()  [unwired: 1 in, 1 out]
                n774 = Unbundle By Name("Set Card.Channel") -> ("Crate"=w1577:i32)
                n775 = Tick Count (ms)() -> (millisecond timer value=w1576:u32)
                n776 = case shown="1" w1577 {
                  tunnel: [_ w1585 w1597 w1609] -> w1579
                  tunnel: w1576 -> [_ w1584 w1596 w1608]
                  frame Default {
                  }
                  frame 0 {
                    n777 = while {
                      tunnel: [w1588] -> w1585
                      tunnel: w1584 -> [w1586]
                      stop <- w1594 stop-if-true
                      # "if we're in the process of a page read, \nwait up to 6s for it to finish, \nthen timeout and abandon the write."
                      n778 = Tick Count (ms)() -> (millisecond timer value=w1593:u32)
                      n779 = local read "stop"() -> (w1589:bool)
                      n780 = local read "Reading page"() -> (w1595:bool)
                      n781 = Subtract(x=w1593, y=w1586) -> (x-y=w1592:u32)
                      n782 = Greater?(x=w1592, y=u32 6000) -> (0:w1590:bool)
                      n783 = Or(x=w1590, y=w1589) -> (x .or. y?=w1588:bool)
                      n784 = Wait (ms)(milliseconds to wait=u32 500) -> ()  [unwired: 1 out]
                      n785 = Compound Arithmetic op=OR(w1588, invert w1595) -> (w1594:bool)
                    }
                  }
                  frame 1 {
                    n786 = while {
                      tunnel: [w1600] -> w1597
                      tunnel: w1596 -> [w1598]
                      stop <- w1606 stop-if-true
                      # "if we're in the process of a page read, \nwait up to 6s for it to finish, \nthen timeout and abandon the write."
                      n787 = Tick Count (ms)() -> (millisecond timer value=w1605:u32)
                      n788 = local read "Reading LeCroy1 Page"() -> (w1607:bool)
                      n789 = local read "stop"() -> (w1601:bool)
                      n790 = Subtract(x=w1605, y=w1598) -> (x-y=w1604:u32)
                      n791 = Greater?(x=w1604, y=u32 6000) -> (0:w1602:bool)
                      n792 = Or(x=w1602, y=w1601) -> (x .or. y?=w1600:bool)
                      n793 = Wait (ms)(milliseconds to wait=u32 500) -> ()  [unwired: 1 out]
                      n794 = Compound Arithmetic op=OR(w1600, invert w1607) -> (w1606:bool)
                    }
                  }
                  frame 2 {
                    n795 = while {
                      tunnel: [w1612] -> w1609
                      tunnel: w1608 -> [w1610]
                      stop <- w1618 stop-if-true
                      # "if we're in the process of a page read, \nwait up to 6s for it to finish, \nthen timeout and abandon the write."
                      n796 = Tick Count (ms)() -> (millisecond timer value=w1617:u32)
                      n797 = local read "Reading LeCroy2 Page"() -> (w1619:bool)
                      n798 = local read "stop"() -> (w1613:bool)
                      n799 = Subtract(x=w1617, y=w1610) -> (x-y=w1616:u32)
                      n800 = Greater?(x=w1616, y=u32 6000) -> (0:w1614:bool)
                      n801 = Or(x=w1614, y=w1613) -> (x .or. y?=w1612:bool)
                      n802 = Wait (ms)(milliseconds to wait=u32 500) -> ()  [unwired: 1 out]
                      n803 = Compound Arithmetic op=OR(w1612, invert w1619) -> (w1618:bool)
                    }
                  }
                }
                n804 = local write "Set channel property"(FALSE ("Set channel property")) -> ()
                n805 = case shown="False" w1579 {
                  tunnel: [w1638 errorcluster {"status"=TRUE, "code"=0, "source"="Aborted Set Channel Property call: timeout waiting for page read to finish"} ("error IO")] -> w1580
                  tunnel: "Set Card.Channel" -> [w1627 _]
                  frame False {
                    n806 = Format Into String("Property") -> (resulting string=w1635:string, error out=w1631:errorcluster)  [unwired: 3 in]
                    n807 = local read "Channel Settings File"() -> (w1622:path)
                    n808 = case shown="\"Vfile\"" "Property" {
                      tunnel: [_ w1666 w1669 w1676 w1683 w1690 w1699] -> w1630
                      tunnel: "Value" -> [w1662 w1667 w1673 w1680 w1687 w1693 w1700]
                      tunnel: [w1658 w1664 w1668 w1675 w1682 w1696 w1698] -> w1634
                      tunnel: w1631 -> [_ _ _ _ _ w1689 _]
                      frame "Iset" {
                        n809 = Variant To Data(type=0.0 ("precision (6)"), Variant=w1662) -> (data=w1660:dbl, error out=w1661:errorcluster)  [unwired: 1 in]
                        n810 = Format Into String(format string="%.2pA", error in=w1661, w1660) -> (resulting string=w1658:string)  [unwired: 1 in, 1 out]
                      }
                      frame "Name" {
                        n811 = Variant To Data(type="" ("format string"), Variant=w1667) -> (data=w1664:string, error out=w1666:errorcluster)  [unwired: 1 in]
                      }
                      frame "Vset", "Vbackup" {
                        n812 = Variant To Data(type=0.0 ("precision (6)"), Variant=w1673) -> (data=w1671:dbl, error out=w1672:errorcluster)  [unwired: 1 in]
                        n813 = Format Into String(format string="%.2fV", error in=w1672, w1671) -> (resulting string=w1668:string, error out=w1669:errorcluster)  [unwired: 1 in]
                      }
                      frame "Vswmax" {
                        n814 = Variant To Data(type=0 ("precision (6)"), Variant=w1680) -> (data=w1678:i32, error out=w1679:errorcluster)  [unwired: 1 in]
                        n815 = Format Into String(format string="%dV", error in=w1679, w1678) -> (resulting string=w1675:string, error out=w1676:errorcluster)  [unwired: 1 in]
                      }
                      frame "Vfile" {
                        n816 = Variant To Data(type=0 ("precision (6)"), Variant=w1687) -> (data=w1685:i32, error out=w1686:errorcluster)  [unwired: 1 in]
                        n817 = Format Into String(format string="%dV", error in=w1686, w1685) -> (resulting string=w1682:string, error out=w1683:errorcluster)  [unwired: 1 in]
                      }
                      frame "Enable" {
                        n818 = Variant To Data(error in=w1689, type=FALSE ("Set channel property"), Variant=w1693) -> (data=w1691:bool, error out=w1690:errorcluster)
                        n819 = Select(t="ON" ("string"), s=w1691, f="OFF" ("string")) -> (s? t:f=w1696:string)
                      }
                      frame "Flag" {
                        n820 = Variant To Data(type=FALSE ("Set channel property"), Variant=w1700) -> (data=w1697:bool, error out=w1699:errorcluster)  [unwired: 1 in]
                        n821 = call-poly "num to string small.vi"("number"=w1697) -> ("String"=w1698:string)  [unwired: 14 in]
                      }
                    }
                    n822 = case shown="\"Vfile\"" "Property" {
                      selector: "Property" -> [w1649 w1651]
                      tunnel: "Value" -> [w1648 w1657]
                      tunnel: w1627 -> [w1650 w1656]
                      tunnel: [_ w1655] -> w1626
                      tunnel: [w1650 w1654] -> w1624
                      tunnel: [w1649 w1653] -> w1620
                      tunnel: [w1648 w1652] -> w1623
                      frame "Vfile" {
                      }
                      frame Default {
                        n823 = call "set channel property.vi"("Value"=w1657, "Property"=w1651, "Card.Channel"=w1656) -> ("error out"=w1655:errorcluster, "Value Out"=w1652:variant, "Property Out"=w1653:T4, "Card.Channel Out"=w1654:T3)  [unwired: 5 in]
                      }
                    }
                    n824 = Unbundle By Name(w1627) -> ("Crate"=w1628:i32, "Card.Channel"=w1629:dbl)
                    n825 = case shown="Default" w1620 {
                      selector: w1620 -> [_ w1642]
                      tunnel: w1626 -> [w1641 w1647]
                      tunnel: [w1641 w1646] -> w1625
                      tunnel: w1624 -> [_ w1645]
                      tunnel: w1623 -> [_ w1644]
                      tunnel: w1622 -> [_ w1643]
                      frame Default {
                      }
                      frame "Flag" {
                        n826 = call "update channel file.vi"("Channel Properties File"=w1643, "error in"=w1647, "Value"=w1644, "Property"=w1642, "Channel"=w1645) -> ("error out"=w1646:errorcluster)  [unwired: 6 in]
                      }
                    }
                    n827 = Format Into String(format string="Setting channel %d.%.2f %s to %s" ("string"), error in=w1630, w1628, w1629, w1635, w1634) -> (resulting string=w1633:string, error out=w1632:errorcluster)  [unwired: 1 in]
                    n828 = call "Append to display log.vi"("error in"=w1632, "string"=w1633) -> ("error out"=w1640:errorcluster)  [unwired: 9 in]
                    n829 = call "Append to event log.vi"("error in"=w1632, "string"=w1633) -> ("error out"=w1637:errorcluster)  [unwired: 9 in]
                    n830 = call <vilib>:"Clear Errors.vi"("error in (no error)"=w1640) -> ()  [unwired: 5 in, 2 out]
                    n831 = Merge Errors(w1625, w1637) -> (w1638:errorcluster)
                  }
                  frame True {
                    # "skip write"
                  }
                }
              }
              event Value Change {
                n832 = event-data() -> ()  [unwired: 1 in, 2 out]
                n833 = case shown="\"Imax\"" "Group Prop" {
                  tunnel: [T22 {"Minimum"=0.0, "Maximum"=2200.0, "Increment"=0.01} ("Data Entry Limits") T22 {"Minimum"=0.0, "Maximum"=1.0, "Increment"=1e-08} ("Data Entry Limits") T22 {"Minimum"=0.0, "Maximum"=2200.0, "Increment"=1.0} ("Data Entry Limits") T22 {"Minimum"=0.0, "Maximum"=1000.0, "Increment"=0.1} ("Data Entry Limits") T22 {"Minimum"=0.0, "Maximum"=1.0, "Increment"=1.0} ("Data Entry Limits") T22 {"Minimum"=0.0, "Maximum"=9999.0, "Increment"=0.001} ("Data Entry Limits")] -> w1707
                  tunnel: ["%07.2f" ("Format String") "%.3pA" ("Format String") "%04d" ("Format String") "%05.1f" ("Format String") "%1d" ("Format String") "%f" ("Format String")] -> w1706
                  frame "Vset" {
                  }
                  frame "Imax" {
                  }
                  frame "Vswmax" {
                  }
                  frame "Trip Time" {
                  }
                  frame "Enable" {
                  }
                  frame Default {
                  }
                }
                n834 = property on="Value 2" class="DigNum (strict)"("FormatString"=w1706, "NumText.FormatString"=w1706, "Data Range"=w1707) -> (error out=w1703:errorcluster)  [unwired: 2 in, 1 out]
              }
              event "Set Group Property": Value Change {
                # "For Vset, Imax, if a group value is applied and some channels have SWmax below the applied value\nwhile others have a SWmax above the applied value, those for which the new value is in range will apply it\nwhile those for which it is out of range will ignore it. \nFor Vswmax, if a group value is applied that is out of range, all channels will coerce to within range.\nFor trip, values will coerce - values > 1000 willl coerce to 'Inf.'"
                n835 = event-data() -> ()  [unwired: 1 in, 1 out]
                n836 = Tick Count (ms)() -> (millisecond timer value=w1723:u32)
                n837 = while {
                  tunnel: w1723 -> [w1732]
                  tunnel: [w1727] -> w1722
                  stop <- w1734 stop-if-true
                  # "wait up to 10s for it to finish a page read.\nif we still haven't finished by then,\nbreak, and abandon the write."
                  n838 = Tick Count (ms)() -> (millisecond timer value=w1733:u32)
                  n839 = local read "stop"() -> (w1728:bool)
                  n840 = local read "Reading page"() -> (w1735:bool)
                  n841 = Subtract(x=w1733, y=w1732) -> (x-y=w1731:u32)
                  n842 = Greater?(x=w1731, y=u32 6000) -> (0:w1729:bool)
                  n843 = Or(x=w1729, y=w1728) -> (x .or. y?=w1727:bool)
                  n844 = Wait (ms)(milliseconds to wait=u32 500) -> ()  [unwired: 1 out]
                  n845 = Compound Arithmetic op=OR(w1727, invert w1735) -> (w1734:bool)
                }
                n846 = local write "Set Group Property"(FALSE ("element")) -> ()
                n847 = case shown="False" w1722 {
                  tunnel: [w1746 errorcluster {"status"=TRUE, "code"=0, "source"="Aborted Set Group Property call: timeout waiting for page read to finish"} ("error IO")] -> w1724
                  frame False {
                    # "units: Volts or Amps\n(use uA or mA to easily type small numbers)"
                    n848 = local read "Group Prop"() -> (w1747:T7)
                    n849 = call "set group poperty.vi"("Group"="Group", "Property"=w1747, "Value to set"="Value 2") -> ("error out"=w1745:errorcluster)  [unwired: 11 in, 1 out]
                    n850 = Format Into String(w1747) -> (resulting string=w1740:string, error out=w1739:errorcluster)  [unwired: 3 in]
                    n851 = Format Into String(format string="Setting %s %s to %d" ("string"), error in=w1739, "Group", w1740, "Value 2") -> (resulting string=w1738:string, error out=w1737:errorcluster)  [unwired: 1 in]
                    n852 = call "Append to event log.vi"("error in"=w1737, "string"=w1738) -> ("error out"=w1744:errorcluster)  [unwired: 9 in]
                    n853 = call "Append to display log.vi"("error in"=w1737, "string"=w1738) -> ("error out"=w1743:errorcluster)  [unwired: 9 in]
                    n854 = call <vilib>:"Clear Errors.vi"("error in (no error)"=w1743) -> ()  [unwired: 5 in, 2 out]
                    n855 = Merge Errors(w1745, w1744) -> (w1746:errorcluster)
                  }
                  frame True {
                    # "skip if we timeout doing a page read, or if stop is pressed\nwhile we were waiting"
                  }
                }
              }
              event "Restore PMT voltages", "re-read vfile voltages": Value Change {
                w1754 = path "C:/Users/User/Documents/Logs/Last PMT Voltages.csv"  # Last PMT Voltages.csv
                n856 = event-data() -> ("CtlRef"=w1758:refnum<vi>)  [unwired: 1 in]
                n857 = control-ref of="Restore PMT voltages"() -> (w1750:refnum<vi>)
                n858 = local read "Channel Settings File"() -> (w1755:path)
                n859 = local write "Restore PMT voltages"(FALSE ("Restore PMT voltages")) -> ()
                n860 = Equal?(x=w1758, y=w1750) -> (x = y?=w1749:bool)
                n861 = case shown="False" w1749 {
                  tunnel: [w1777 w1789] -> w1771
                  tunnel: [w1776 w1788] -> w1770
                  tunnel: [w1775 w1787] -> w1757
                  tunnel: [w1781 w1786] -> w1756
                  tunnel: w1755 -> [w1774 _]
                  tunnel: w1754 -> [_ w1785]
                  tunnel: ["vfile" ("delimiter (\\t)") "vset" ("delimiter (\\t)")] -> w1753
                  frame False {
                    n862 = call-poly <vilib>:"Read Delimited Spreadsheet.vi"("file path (dialog if empty)"=w1774, "delimiter (\\t)"="," ("delimiter (\\t)")) -> ("all rows"=w1783:string[][])  [unwired: 8 in, 5 out]
                    n863 = Index Array(array=w1783, index (col) #1=2 ("index (row)"), index (col) #2=3 ("disabled index (col)"), index (col) #3=4 ("disabled index (col)"), index (col) #4=5 ("disabled index (col)")) -> (element #1=w1777:string[], element #2=w1776:string[], element #3=w1775:string[], element #4=w1781:string[])  [unwired: 4 in]
                  }
                  frame True {
                    n864 = call-poly <vilib>:"Read Delimited Spreadsheet.vi"("file path (dialog if empty)"=w1785, "transpose? (F)"=TRUE, "delimiter (\\t)"="," ("delimiter (\\t)")) -> ("all rows"=w1791:string[][])  [unwired: 7 in, 5 out]
                    n865 = Index Array(array=w1791) -> (element #1=w1789:string[], element #2=w1788:string[], element #3=w1787:string[], element #4=w1786:string[])  [unwired: 8 in]
                  }
                }
                n866 = for {
                  tunnel: w1771 -> [w1798] mode=indexing
                  tunnel: w1770 -> [w1797] mode=indexing
                  tunnel: [w1800] -> w1768 mode=indexing
                  tunnel: w1764 -> [w1799]
                  tunnel: w1757 -> [w1796] mode=indexing
                  tunnel: w1756 -> [w1795] mode=indexing
                  tunnel: w1753 -> [w1794]
                  tunnel: w1749 -> [w1793]
                  n867 = case shown="False" w1793 {
                    tunnel: [w1806 w1826] -> w1800
                    tunnel: w1799 -> [_ w1825]
                    tunnel: w1798 -> [w1816 w1823]
                    tunnel: w1797 -> [w1815 w1821]
                    tunnel: w1796 -> [w1814 w1820]
                    tunnel: w1795 -> [w1803 w1818]
                    tunnel: w1794 -> [_ w1817]
                    frame False {
                      n868 = Decimal String To Number(string=w1816) -> (number=w1812:i32)  [unwired: 2 in, 1 out]
                      n869 = Decimal String To Number(string=w1815) -> (number=w1811:i32)  [unwired: 2 in, 1 out]
                      n870 = Decimal String To Number(string=w1814) -> (number=w1810:i32)  [unwired: 2 in, 1 out]
                      n871 = Fract/Exp String To Number(string=w1803) -> (number=w1802:dbl)  [unwired: 3 in, 1 out]
                      n872 = To Double Precision Float(number=w1811) -> (double precision float=w1808:dbl)
                      n873 = To Double Precision Float(number=w1810) -> (double precision float=w1809:dbl)
                      n874 = To Variant(anything=w1802) -> (Variant=w1801:variant)
                      n875 = expression code="x/100."(w1809) -> (w1807:dbl)
                      n876 = Compound Arithmetic op=ADD(w1808, w1807) -> (w1805:dbl)
                      n877 = Bundle By Name(cluster=T3 {" Card.Channel"=1.12, "Crate"=0} ("Channel"), "Crate"=w1812, "Card.Channel"=w1805) -> (w1804:T3)
                      n878 = call "update_vfile.vi"("Vfile (V)"=w1801, "Channel"=w1804) -> ("error out"=w1806:errorcluster)  [unwired: 9 in]
                    }
                    frame True {
                      w1822 = "." ("delimiter (\\t)")
                      w1830 = "\r"
                      n879 = Concatenate Strings(w1823, w1822, w1821, w1822, w1820) -> (w1819:string)
                      n880 = Concatenate Strings("msg_id (unused)" ("delimiter (\\t)"), w1830, "write" ("delimiter (\\t)"), w1830, w1817, w1830, w1819, w1830, w1818) -> (w1827:string)
                      n881 = Bundle By Name(cluster=cluster{"Source":T16, "Command":string} {"Source"=enum."INTERNAL", "Command"=""} ("element"), "Command"=w1827) -> (w1824:cluster{"Source":T16, "Command":string})
                      n882 = Enqueue Element(queue=w1825, element=w1824) -> (error out=w1826:errorcluster)  [unwired: 2 in, 2 out]
                    }
                  }
                }
                n883 = Select(t="Re-reading nominal PMT voltages" ("string"), s=w1749, f="Restoring last saved PMT voltages" ("string")) -> (s? t:f=w1759:string)
                n884 = call "Append to display log.vi"("string"=w1759) -> ("error out"=w1769:errorcluster)  [unwired: 10 in]
                n885 = call "Append to event log.vi"("string"=w1759) -> ("error out"=w1765:errorcluster)  [unwired: 10 in]
                n886 = call <vilib>:"Clear Errors.vi"("error in (no error)"=w1769) -> ("error out"=w1766:errorcluster)  [unwired: 5 in, 1 out]
                n887 = Merge Errors(w1768, w1766, w1765) -> (w1767:errorcluster)
              }
              event "Nominal PMT voltages": Value Change {
                w1833 = "Restoring nominal PMT voltages" ("string")
                n888 = event-data() -> ()  [unwired: 1 in, 1 out]
                n889 = global read "CAEN globals.vi" "Channel Array Val"() -> (w1832:T8[])
                n890 = local write "Nominal PMT voltages"(FALSE ("Restore PMT voltages")) -> ()
                n891 = for {
                  tunnel: [w1856] -> w1841 mode=indexing
                  tunnel: w1837 -> [w1855]
                  tunnel: [w1854] -> _ mode=indexing
                  tunnel: w1832 -> [w1851] mode=indexing
                  w1853 = "." ("delimiter (\\t)")
                  w1861 = "\r"
                  n892 = Unbundle By Name(w1851) -> ("Crate"=w1850:i32, "Card"=w1849:i32, "Channel"=w1848:i32, "Vfile (V)"=w1847:dbl)
                  n893 = Number To Decimal String(number=w1850) -> (decimal integer string=w1843:string)  [unwired: 1 in]
                  n894 = Number To Decimal String(number=w1849) -> (decimal integer string=w1844:string)  [unwired: 1 in]
                  n895 = Number To Decimal String(number=w1848) -> (decimal integer string=w1845:string)  [unwired: 1 in]
                  n896 = Number To Fractional String(number=w1847) -> (F-format string=w1846:string)  [unwired: 3 in]
                  n897 = Concatenate Strings(w1843, w1853, w1844, w1853, w1845) -> (w1852:string)
                  n898 = Concatenate Strings("msg_id (unused)" ("delimiter (\\t)"), w1861, "write" ("delimiter (\\t)"), w1861, "vset" ("delimiter (\\t)"), w1861, w1852, w1861, w1846) -> (w1857:string)
                  n899 = Bundle By Name(cluster=cluster{"Source":T16, "Command":string} {"Source"=enum."INTERNAL", "Command"=""} ("element"), "Command"=w1857) -> (w1854:cluster{"Source":T16, "Command":string})
                  n900 = Enqueue Element(queue=w1855, element=w1854) -> (error out=w1856:errorcluster)  [unwired: 2 in, 2 out]
                }
                n901 = call "Append to display log.vi"("string"=w1833) -> ("error out"=w1842:errorcluster)  [unwired: 10 in]
                n902 = call "Append to event log.vi"("string"=w1833) -> ("error out"=w1838:errorcluster)  [unwired: 10 in]
                n903 = call <vilib>:"Clear Errors.vi"("error in (no error)"=w1842) -> ("error out"=w1839:errorcluster)  [unwired: 5 in, 1 out]
                n904 = Merge Errors(w1841, w1839, w1838) -> (w1840:errorcluster)
              }
              event "Lecroy 1 enable": Value Change {
                n905 = event-data() -> ()  [unwired: 1 in, 5 out]
                n906 = global read "CAEN globals.vi" "LeCroy 1 VISA"() -> (w1875:refnum<visa-resource-name>)
                n907 = Select(t=T23 "ON" ("Action"), s="Lecroy 1 enable", f=T23 "OFF" ("Action")) -> (s? t:f=w1872:T23)
                n908 = Select(t="Enabling LeCroy 1 HV" ("string"), s="Lecroy 1 enable", f="Disabling LeCroy 1 HV" ("string")) -> (s? t:f=w1864:string)
                n909 = call "General Commands.vi"("Action"=w1872, "VISA in"=w1875) -> ("error out"=w1870:errorcluster)  [unwired: 7 in, 2 out]
                n910 = call "Append to display log.vi"("string"=w1864) -> ("error out"=w1871:errorcluster)  [unwired: 10 in]
                n911 = call "Append to event log.vi"("string"=w1864) -> ("error out"=w1868:errorcluster)  [unwired: 10 in]
                n912 = call <vilib>:"Clear Errors.vi"("error in (no error)"=w1871) -> ()  [unwired: 5 in, 2 out]
                n913 = Merge Errors(w1868, w1870) -> (w1869:errorcluster)
              }
              event "Lecroy 2 enable": Value Change {
                n914 = event-data() -> ()  [unwired: 1 in, 5 out]
                n915 = global read "CAEN globals.vi" "LeCroy 2 VISA"() -> (w1888:refnum<visa-resource-name>)
                n916 = Select(t=T23 "ON" ("Action"), s="Lecroy 2 enable", f=T23 "OFF" ("Action")) -> (s? t:f=w1885:T23)
                n917 = Select(t="Enabling LeCroy 2 HV" ("string"), s="Lecroy 2 enable", f="Disabling LeCroy 2 HV" ("string")) -> (s? t:f=w1878:string)
                n918 = call "General Commands.vi"("Action"=w1885, "VISA in"=w1888) -> ("error out"=w1883:errorcluster)  [unwired: 7 in, 2 out]
                n919 = call "Append to display log.vi"("string"=w1878) -> ("error out"=w1884:errorcluster)  [unwired: 10 in]
                n920 = call "Append to event log.vi"("string"=w1878) -> ("error out"=w1881:errorcluster)  [unwired: 10 in]
                n921 = call <vilib>:"Clear Errors.vi"("error in (no error)"=w1884) -> ()  [unwired: 5 in, 2 out]
                n922 = Merge Errors(w1881, w1883) -> (w1882:errorcluster)
              }
              event "Caen enable": Value Change {
                n923 = event-data() -> ()  [unwired: 1 in, 5 out]
                n924 = disable-structure shown="Enabled" {
                  disable-tunnel: [w1907 w1910] -> w1891
                  disable-tunnel: "Caen enable" -> [w1906 w1908]
                  frame Enabled {
                    n925 = Select(t=1.0 ("Value 2"), s=w1906, f=0.0 ("Value 2")) -> (s? t:f=w1900:dbl)
                    n926 = local write "Value 2"(w1900) -> ()
                    n927 = property on="Group" class="CmbBox"("Value"="TANK" ("Group")) -> (error out=w1904:errorcluster)  [unwired: 2 in, 1 out]
                    n928 = property on="Group Prop" class="Enum (strict)"(error in=w1904, "Value"=Group_Properties."Enable" ("Group Prop")) -> (error out=w1901:errorcluster)  [unwired: 1 in, 1 out]
                    n929 = property on="Set Group Property" class="Bool (strict)"(error in=w1901, "Val(Sgnl)"=TRUE ("Set Group Property")) -> (error out=w1907:errorcluster)  [unwired: 1 in, 1 out]
                  }
                  frame Disabled {
                    n930 = global read "CAEN globals.vi" "CAEN_ch_enable_pin"() -> (w1912:u8)
                    n931 = global read "CAEN globals.vi" "Arduino VISA"() -> (w1911:refnum<visa-resource-name>)
                    n932 = call "read_write_arduino.vi"("VISA in"=w1911, "Pin Num"=w1912, "Read (0, default)/Write (1)"=TRUE, "State"=w1908) -> ("error out"=w1910:errorcluster)  [unwired: 8 in, 3 out]
                  }
                }
                n933 = Select(t="Enabling CAEN HV" ("string"), s="Caen enable", f="Disabling CAEN HV" ("string")) -> (s? t:f=w1892:string)
                n934 = call "Append to display log.vi"("string"=w1892) -> ("error out"=w1897:errorcluster)  [unwired: 10 in]
                n935 = call "Append to event log.vi"("string"=w1892) -> ("error out"=w1895:errorcluster)  [unwired: 10 in]
                n936 = call <vilib>:"Clear Errors.vi"("error in (no error)"=w1897) -> ()  [unwired: 5 in, 2 out]
                n937 = Merge Errors(w1895, w1891) -> (w1896:errorcluster)
              }
              event "CAEN Vsel Buffer": Value Change {
                n938 = event-data() -> ()  [unwired: 1 in, 1 out]
                n939 = global read "CAEN globals.vi" "CAEN_buffer_pin"() -> (w1919:u8)
                n940 = global read "CAEN globals.vi" "Arduino VISA"() -> (w1918:refnum<visa-resource-name>)
                n941 = Select(t="Switching CAEN Vsel Buffer to V1" ("string"), s="CAEN Vsel Buffer", f="Switching CAEN Vsel Buffer to V0" ("string")) -> (s? t:f=w1920:string)
                n942 = call "read_write_arduino.vi"("VISA in"=w1918, "Pin Num"=w1919, "Read (0, default)/Write (1)"=TRUE, "State"="CAEN Vsel Buffer") -> ("error out"=w1915:errorcluster)  [unwired: 8 in, 3 out]
                n943 = call "Append to display log.vi"("string"=w1920) -> ("error out"=w1924:errorcluster)  [unwired: 10 in]
                n944 = call "Append to event log.vi"("string"=w1920) -> ("error out"=w1923:errorcluster)  [unwired: 10 in]
                n945 = call <vilib>:"Clear Errors.vi"("error in (no error)"=w1924) -> ()  [unwired: 5 in, 2 out]
                n946 = Merge Errors(w1923, w1915) -> (w1916:errorcluster)
              }
              event "Save PMT voltages": Value Change {
                # "enqueue the action to actually save the voltages"
                # "But first activate all active\nchannels in the channel\ncluster to ensure they\nare all recorded to the file"
                n947 = event-data() -> ()  [unwired: 1 in, 6 out]
                n948 = local write "Save PMT voltages"(FALSE ("Restore PMT voltages")) -> ()
                n949 = Enqueue Element(queue=w1931, element=cluster{"Source":T16, "Command":string} {"Source"=enum."Save_PMT_Voltages", "Command"=""}, timeout in ms (-1)=10000) -> (error out=w1928:errorcluster)  [unwired: 1 in, 2 out]
                n950 = property on="Show Group In Displayed Channels" class="Bool (strict)"(error in=w1928, "Val(Sgnl)"=TRUE ("Restore PMT voltages")) -> (error out=w1927:errorcluster)  [unwired: 1 in, 1 out]
                n951 = local write "Group"("ACTIVE" ("Group")) -> ()
              }
              event "Save PMT Voltage File": Value Change {
                w1943 = "Saving current PMT set voltages" ("string")
                # "Proper implementation of the saving. \nthe button on the FP actually calls a proxy that first\nenqueues an event to activate the active channels\nin the channel list, first, to ensure we record all the\nactive channels."
                n952 = event-data() -> ()  [unwired: 1 in, 5 out]
                n953 = global read "CAEN globals.vi" "Channel Array Val"() -> (w1949:T8[])
                n954 = for {
                  tunnel: w1949 -> [w1964] mode=indexing
                  shift-right: [w1960] -> w1937
                  shift-left: string[][] [] -> [w1959]
                  n955 = Unbundle By Name(w1964) -> ("Crate"=w1955:i32, "Card"=w1953:i32, "Channel"=w1952:i32, "Vset (V)"=w1962:dbl, "Channel Name"=w1956:string)
                  n956 = Number To Decimal String(number=w1955) -> (decimal integer string=w1954:string)  [unwired: 1 in]
                  n957 = Number To Decimal String(number=w1953) -> (decimal integer string=w1951:string)  [unwired: 1 in]
                  n958 = Number To Decimal String(number=w1952) -> (decimal integer string=w1950:string)  [unwired: 1 in]
                  n959 = Number To Fractional String(number=w1962) -> (F-format string=w1963:string)  [unwired: 3 in]
                  n960 = Empty String/Path?(string/path=w1956) -> (empty?=w1961:bool)
                  n961 = Build Array(w1954, w1951, w1950, w1963) -> (w1958:string[])
                  n962 = Build Array (concatenate)(w1959, w1958) -> (w1957:string[][])
                  n963 = Select(t=w1959, s=w1961, f=w1957) -> (s? t:f=w1960:string[][])
                }
                n964 = local write "Save PMT Voltage File"(FALSE ("Restore PMT voltages")) -> ()
                n965 = call "Append to display log.vi"("string"=w1943) -> ("error out"=w1944:errorcluster)  [unwired: 10 in]
                n966 = call "Append to event log.vi"("string"=w1943) -> ("error out"=w1940:errorcluster)  [unwired: 10 in]
                n967 = call <vilib>:"Clear Errors.vi"("error in (no error)"=w1944) -> ("error out"=w1941:errorcluster)  [unwired: 5 in, 1 out]
                n968 = call-poly <vilib>:"Write Delimited Spreadsheet.vi"("file path (dialog if empty)"=path "C:/Users/User/Documents/Logs/Last PMT Voltages.csv" ("path"), "2D data"=w1937, "append to file? (new file:F)"=FALSE ("append to file? (F)"), "delimiter (\\t)"="," ("delimiter (\\t)")) -> ("error out"=w1942:errorcluster)  [unwired: 10 in, 1 out]
                n969 = Merge Errors(w1942, w1941, w1940) -> (w1939:errorcluster)
              }
              event "Kill All": Value Change {
                # "TODO: add abort to read channel page subvi!"
                n970 = event-data() -> ()  [unwired: 1 in, 1 out]
                n971 = Tick Count (ms)() -> (millisecond timer value=w1966:u32)
                n972 = while {
                  tunnel: w1966 -> [w1977]
                  tunnel: [w1972] -> w1965
                  stop <- w1979 stop-if-true
                  # "wait up to 10s for it to finish a page read.\nif we still haven't finished by then,\nbreak, and abandon the write."
                  n973 = Tick Count (ms)() -> (millisecond timer value=w1978:u32)
                  n974 = local read "stop"() -> (w1973:bool)
                  n975 = local read "Reading page"() -> (w1980:bool)
                  n976 = Subtract(x=w1978, y=w1977) -> (x-y=w1976:u32)
                  n977 = Greater?(x=w1976, y=u32 6000) -> (0:w1974:bool)
                  n978 = Or(x=w1974, y=w1973) -> (x .or. y?=w1972:bool)
                  n979 = Wait (ms)(milliseconds to wait=u32 500) -> ()  [unwired: 1 out]
                  n980 = Compound Arithmetic op=OR(w1972, invert w1980) -> (w1979:bool)
                }
                n981 = local write "Kill All"(FALSE ("Kill All")) -> ()
                n982 = case shown="False" w1965 {
                  tunnel: [w1999 errorcluster {"status"=TRUE, "code"=0, "source"="Could not perform KILL ALL! \nTimeout waiting for page read to finish!"} ("error IO")] -> w1967
                  frame False {
                    w1981 = "OFF\r" ("write buffer")
                    w1997 = "Killing all channels" ("string")
                    n983 = call "Get Mainframe VISA.vi"("Crate"=1) -> ("Error Out"=w1984:errorcluster, "VISA out"=w1985:refnum<visa-resource-name>)  [unwired: 8 in, 1 out]
                    n984 = call "Get Mainframe VISA.vi"("Crate"=2) -> ("Error Out"=w1987:errorcluster, "VISA out"=w1986:refnum<visa-resource-name>)  [unwired: 8 in, 1 out]
                    n985 = call "Get Mainframe VISA.vi"("Crate"=0) -> ("Error Out"=w1992:errorcluster, "VISA out"=w1991:refnum<visa-resource-name>)  [unwired: 8 in, 1 out]
                    n986 = call "go to desired page.vi"("VISA in"=w1991, "Set Cluster"=T24 {"set index"=0, "set Screen"="Kill Confirm", "set subpage"=0, "set column"=0, "Group"="", "Crate"=0}, "error in"=w1992) -> ("VISA out"=w1996:refnum<visa-resource-name>, "error out"=w1995:errorcluster)  [unwired: 9 in, 2 out]
                    n987 = VISA Write(VISA resource name=w1986, write buffer=w1981, error in (no error)=w1987) -> (error out=w1982:errorcluster)  [unwired: 2 out]
                    n988 = VISA Write(VISA resource name=w1985, write buffer=w1981, error in (no error)=w1984) -> (error out=w1983:errorcluster)  [unwired: 2 out]
                    n989 = VISA Write(VISA resource name=w1996, write buffer="Y\n", error in (no error)=w1995) -> (VISA resource name out=w1993:refnum<visa-resource-name>, error out=w1994:errorcluster)  [unwired: 1 out]
                    n990 = call "read caen.vi"("VISA in"=w1993, "error in"=w1994) -> ("error out"=w2000:errorcluster)  [unwired: 8 in, 5 out]
                    n991 = call "Append to event log.vi"("string"=w1997) -> ("error out"=w1998:errorcluster)  [unwired: 10 in]
                    n992 = call "Append to display log.vi"("string"=w1997) -> ("error out"=w2001:errorcluster)  [unwired: 10 in]
                    n993 = Merge Errors(w2000, w1983, w1982, w1998) -> (w1999:errorcluster)
                    n994 = call <vilib>:"Clear Errors.vi"("error in (no error)"=w2001) -> ()  [unwired: 5 in, 2 out]
                  }
                  frame True {
                  }
                }
              }
              event "Clear Alarms": Value Change {
                n995 = event-data() -> ()  [unwired: 1 in, 1 out]
                n996 = Tick Count (ms)() -> (millisecond timer value=w2006:u32)
                n997 = while {
                  tunnel: w2006 -> [w2017]
                  tunnel: [w2012] -> w2005
                  stop <- w2019 stop-if-true
                  # "wait up to 10s for it to finish a page read.\nif we still haven't finished by then,\nbreak, and abandon the write."
                  n998 = Tick Count (ms)() -> (millisecond timer value=w2018:u32)
                  n999 = local read "stop"() -> (w2013:bool)
                  n1000 = local read "Reading page"() -> (w2020:bool)
                  n1001 = Subtract(x=w2018, y=w2017) -> (x-y=w2016:u32)
                  n1002 = Greater?(x=w2016, y=u32 6000) -> (0:w2014:bool)
                  n1003 = Or(x=w2014, y=w2013) -> (x .or. y?=w2012:bool)
                  n1004 = Wait (ms)(milliseconds to wait=u32 500) -> ()  [unwired: 1 out]
                  n1005 = Compound Arithmetic op=OR(w2012, invert w2020) -> (w2019:bool)
                }
                n1006 = local write "Clear Alarms"(FALSE ("Clear Alarms")) -> ()
                n1007 = case shown="False" w2005 {
                  tunnel: [w2038 errorcluster {"status"=TRUE, "code"=0, "source"="Could not perform Clear Alarms: timeout waiting for page read to finish"} ("error IO")] -> w2007
                  frame False {
                    w2036 = "Clearing alarms" ("string")
                    w2035 = "Everything is awesome" ("summary status")
                    w2033 = FALSE ("Blinking")
                    n1008 = property on="Status message" class="Str"() -> (error out=w2027:errorcluster, "Blinking"=w2026:bool)  [unwired: 2 in, 1 out]
                    n1009 = Get Date/Time String(want seconds? (F)=TRUE) -> (date string=w2032:string, time string=w2031:string)  [unwired: 2 in]
                    n1010 = call <vilib>:"Space Constant.vi"() -> ("String"=w2030:string)
                    n1011 = Concatenate Strings(w2032, w2030, w2031) -> (w2028:string)
                    n1012 = property on="Status message" class="Str"(error in=w2027, "Value"=w2035, "Blinking"=w2033) -> (error out=w2025:errorcluster)  [unwired: 1 in, 1 out]
                    n1013 = property on="summary status" class="Str"(error in=w2025, "Value"=w2035, "Text.BGColor"=u32 46096, "Blinking"=w2033) -> (error out=w2023:errorcluster)  [unwired: 1 in, 1 out]
                    n1014 = local write "Timestamp"(w2028) -> ()
                    n1015 = Or(x=w2026, y=w2025) -> (x .or. y?=w2024:bool)
                    n1016 = case shown="True" w2024 {
                      tunnel: [_ w2041] -> w2022
                      tunnel: [_ w2040] -> w2021
                      frame False {
                      }
                      frame True {
                        w2044 = T23 "CL" ("Action")
                        n1017 = disable-structure shown="Enabled" {
                          disable-tunnel: [w2051 _] -> w2040
                          frame Enabled {
                            # "pressing 'a' at main menu clears alarms"
                            n1018 = call "Get Mainframe VISA.vi"("Crate"=0) -> ("Error Out"=w2053:errorcluster, "VISA out"=w2052:refnum<visa-resource-name>)  [unwired: 8 in, 1 out]
                            n1019 = call "go to desired page.vi"("VISA in"=w2052, "Set Cluster"=T24 {"set index"=48, "set Screen"="Main Menu", "set subpage"=0, "set column"=0, "Group"="ACTIVE", "Crate"=0}, "error in"=w2053) -> ("VISA out"=w2062:refnum<visa-resource-name>, "error out"=w2061:errorcluster)  [unwired: 9 in, 2 out]
                            n1020 = VISA Write(VISA resource name=w2062, write buffer="A", error in (no error)=w2061) -> (VISA resource name out=w2057:refnum<visa-resource-name>, error out=w2059:errorcluster)  [unwired: 1 out]
                            n1021 = call <userlib>:"Wait (ms)__ogtk.vi"("error in (no error)"=w2059, "milliseconds to wait"=u32 1000) -> ("error out"=w2056:errorcluster)  [unwired: 8 in, 1 out]
                            n1022 = call "read caen.vi"("VISA in"=w2057, "error in"=w2056) -> ("error out"=w2051:errorcluster)  [unwired: 8 in, 5 out]
                          }
                          frame Disabled {
                          }
                        }
                        n1023 = call "Get Mainframe VISA.vi"("Crate"=1) -> ("Error Out"=w2045:errorcluster, "VISA out"=w2048:refnum<visa-resource-name>)  [unwired: 8 in, 1 out]
                        n1024 = call "Get Mainframe VISA.vi"("Crate"=2) -> ("Error Out"=w2047:errorcluster, "VISA out"=w2046:refnum<visa-resource-name>)  [unwired: 8 in, 1 out]
                        n1025 = call "General Commands.vi"("error in"=w2045, "Action"=w2044, "VISA in"=w2048) -> ("error out"=w2043:errorcluster)  [unwired: 6 in, 2 out]
                        n1026 = call "General Commands.vi"("error in"=w2047, "Action"=w2044, "VISA in"=w2046) -> ("error out"=w2042:errorcluster)  [unwired: 6 in, 2 out]
                        n1027 = Merge Errors(w2043, w2042) -> (w2041:errorcluster)
                      }
                    }
                    n1028 = call "Append to event log.vi"("string"=w2036) -> ("error out"=w2037:errorcluster)  [unwired: 10 in]
                    n1029 = call "Append to display log.vi"("string"=w2036) -> ("error out"=w2039:errorcluster)  [unwired: 10 in]
                    n1030 = call <vilib>:"Clear Errors.vi"("error in (no error)"=w2039) -> ()  [unwired: 5 in, 2 out]
                    n1031 = Merge Errors(w2022, w2021, w2023, w2037) -> (w2038:errorcluster)
                  }
                  frame True {
                  }
                }
              }
              event "Refresh Crate Map": Value Change {
                n1032 = event-data() -> ()  [unwired: 1 in, 2 out]
                n1033 = Tick Count (ms)() -> (millisecond timer value=w2065:u32)
                n1034 = while {
                  tunnel: w2065 -> [w2076]
                  tunnel: [w2071] -> w2064
                  stop <- w2078 stop-if-true
                  # "wait up to 10s for it to finish a page read.\nif we still haven't finished by then,\nbreak, and abandon the write."
                  n1035 = Tick Count (ms)() -> (millisecond timer value=w2077:u32)
                  n1036 = local read "stop"() -> (w2072:bool)
                  n1037 = local read "Reading page"() -> (w2079:bool)
                  n1038 = Subtract(x=w2077, y=w2076) -> (x-y=w2075:u32)
                  n1039 = Greater?(x=w2075, y=u32 6000) -> (0:w2073:bool)
                  n1040 = Or(x=w2073, y=w2072) -> (x .or. y?=w2071:bool)
                  n1041 = Wait (ms)(milliseconds to wait=u32 500) -> ()  [unwired: 1 out]
                  n1042 = Compound Arithmetic op=OR(w2071, invert w2079) -> (w2078:bool)
                }
                n1043 = local write "Refresh Crate Map"(FALSE ("Refresh Crate Map")) -> ()
                n1044 = case shown="False" w2064 {
                  tunnel: [w2083 errorcluster {"status"=TRUE, "code"=0, "source"="Could not refresh crate map: timeout waiting for page read to finish"} ("error IO")] -> w2066
                  frame False {
                    w2081 = "Refreshing crate map" ("string")
                    n1045 = invoke on="Channel Array" class="Arr (strict)" method="Reinit To Default"() -> (error out=w2080:errorcluster)  [unwired: 3 in, 2 out]
                    n1046 = call "Append to event log.vi"("string"=w2081) -> ("error out"=w2082:errorcluster)  [unwired: 10 in]
                    n1047 = call "Append to display log.vi"("string"=w2081) -> ("error out"=w2085:errorcluster)  [unwired: 10 in]
                    n1048 = call <vilib>:"Clear Errors.vi"("error in (no error)"=w2085) -> ()  [unwired: 5 in, 2 out]
                    n1049 = call "get crate maps.vi"("error in"=w2080) -> ("error out"=w2084:errorcluster)  [unwired: 12 in, 2 out]
                    n1050 = Merge Errors(w2084, w2082) -> (w2083:errorcluster)
                  }
                  frame True {
                  }
                }
              }
              event "get log file": Value Change {
                n1051 = event-data() -> ()  [unwired: 1 in, 2 out]
                n1052 = local read "log file to get"() -> (w2091:string)
                n1053 = case shown="\"error\"" w2091 {
                  selector: w2091 -> [w2114 _ _]
                  tunnel: [w2111 w2115 w2116] -> w2100
                  tunnel: "%d-%d-%d" ("format string") -> [w2113 _ _]
                  tunnel: [w2110 _ _] -> w2089
                  tunnel: "Monitoring_Log_%d-%d-%d.csv" ("format string") -> [w2109 _ _]
                  frame Default {
                    n1054 = local read "Current Channel Log"() -> (w2112:path)
                    n1055 = Scan From String(format string=w2113, input string=w2114) -> (error out=w2107:errorcluster, output 1=w2104:i32, output 2=w2105:i32, output 3=w2106:i32)  [unwired: 5 in, 2 out]
                    n1056 = Format Into String(format string=w2109, error in=w2107, w2104, w2105, w2106) -> (resulting string=w2108:string, error out=w2110:errorcluster)  [unwired: 1 in]
                    n1057 = Build Path(base path=w2112, name or relative path=w2108) -> (appended path=w2111:path)
                  }
                  frame "event" {
                    n1058 = local read "Current Event Log"() -> (w2115:path)
                  }
                  frame "error" {
                    n1059 = local read "Current Error Log"() -> (w2116:path)
                  }
                }
                n1060 = local write "get log file"(FALSE ("get log file")) -> ()
                n1061 = Read from Text File(file (use dialog)=w2100, error in=w2089) -> (refnum out=w2099:refnum<file>, text=w2093:string, error out=w2098:errorcluster)  [unwired: 2 in, 1 out]
                n1062 = local read "ZMQ Reply"() -> (w2097:string[])
                n1063 = Concatenate Strings("\"contents\":\"" ("string"), w2093, "\"" ("string")) -> (w2092:string)
                n1064 = Close File(refnum=w2099, error in=w2098) -> (error out=w2088:errorcluster)  [unwired: 1 out]
                n1065 = Build Array (concatenate)(w2097, w2092) -> (w2096:string[])
                n1066 = local write "ZMQ Reply"(w2096) -> ()
              }
              event "Handle ZMQ message": Value Change {
                # "Add writing this ZMQ log\nto file!"
                # "{\"msg_type\": \"Data/Command\", \"msg_property\", \"pmt_name\":\"pmt_value\"}"
                n1067 = event-data() -> ()  [unwired: 1 in, 1 out]
                n1068 = Dequeue Element(queue=w2136) -> (queue out=w2134:refnum<queue>, element=w2133:cluster{"Source":T16, "Command":string}, error out=w2120:errorcluster)  [unwired: 2 in, 1 out]
                n1069 = Get Date/Time String(want seconds? (F)=TRUE) -> (date string=w2131:string, time string=w2130:string)  [unwired: 2 in]
                n1070 = call <vilib>:"Space Constant.vi"() -> ("String"=w2129:string)
                n1071 = Unbundle(w2133) -> ("Command"=w2124:string)  [unwired: 1 out]
                "ZMQ message" <- w2124
                n1072 = Concatenate Strings(w2131, w2129, w2130) -> (w2127:string)
                n1073 = call "get zmq message stats.vi"("message"=w2124, "error in"=w2120) -> ("msg_id"=w2118:string, "msg_type"=w2123:string, "msg_property"=w2122:string, "message dup"=w2121:string, "error out"=w2119:errorcluster)  [unwired: 8 in, 1 out]
                n1074 = local read "ZMQ Log"() -> (w2126:string[][])
                n1075 = Build Array(w2127, w2118, w2124) -> (w2117:string[])
                n1076 = while {
                  shift-right: [w2155] -> _
                  shift-left: w2121 -> [w2158]
                  tunnel: w2119 -> [w2157]
                  tunnel: " *\"([^\"]+)\" *: *\"([^\"]+)\"" ("regular expression") -> [w2156]
                  tunnel: [w2152] -> _ mode=indexing
                  tunnel: [w2151] -> _ mode=indexing
                  tunnel: w2134 -> [w2147]
                  tunnel: w2133 -> [w2146]
                  tunnel: [w2141] -> w2132
                  tunnel: w2118 -> [w2148]
                  tunnel: w2123 -> [w2150]
                  tunnel: w2122 -> [w2149]
                  stop <- w2144 stop-if-true
                  n1077 = xnode "Match Regular Expression"("input string"=w2158, "regular expression"=w2156, "error in"=w2157) -> ("after match"=w2155:string, "offset past match"=w2154:i32, "error out"=w2143:errorcluster, "submatch 1"=w2152:string, "submatch 2"=w2151:string)  [unwired: 3 in, 2 out]
                  n1078 = case shown="No Error" w2143 {
                    selector: w2143 -> [_ w2192]
                    tunnel: w2152 -> [w2168 _]
                    tunnel: w2151 -> [w2167 _]
                    tunnel: w2150 -> [w2166 _]
                    tunnel: w2149 -> [w2165 _]
                    tunnel: w2148 -> [w2164 _]
                    tunnel: w2147 -> [w2163 _]
                    tunnel: w2146 -> [w2162 _]
                    tunnel: [w2161 w2192] -> w2141
                    tunnel: Event_Sources."INTERNAL" ("Source") -> [w2160 _]
                    tunnel: "{\"msg_id\":\"" ("Command") -> [w2159 _]
                    frame No Error {
                      n1079 = case shown="\"\"" w2168 {
                        selector: w2168 -> [_ w2171 _]
                        tunnel: w2167 -> [_ w2170 _]
                        tunnel: w2166 -> [_ w2173 _]
                        tunnel: w2165 -> [_ w2172 _]
                        tunnel: w2164 -> [_ w2175 w2184]
                        tunnel: w2163 -> [_ w2180 w2191]
                        tunnel: w2162 -> [_ w2178 w2189]
                        tunnel: [_ w2176 w2188] -> w2161
                        tunnel: w2160 -> [_ w2169 _]
                        tunnel: w2159 -> [_ _ w2183]
                        frame "msg_id", "msg_property", "msg_type", "run" {
                        }
                        frame Default {
                          w2174 = "\r"
                          # "Queue INTERNAL action to\nperform requested operation"
                          n1080 = Concatenate Strings(w2175, w2174, w2173, w2174, w2172, w2174, w2171, w2174, w2170) -> (w2177:string)
                          n1081 = Bundle(cluster=w2178, "Source"=w2169, "Command"=w2177) -> (w2179:cluster{"Source":T16, "Command":string})
                          n1082 = Enqueue Element(queue=w2180, element=w2179) -> (error out=w2176:errorcluster)  [unwired: 2 in, 2 out]
                        }
                        frame "" {
                          # "Send ZMQ reply once all requsted actions\nare performed (we may queue many)"
                          n1083 = Concatenate Strings(w2183, w2184, "\"" ("Command")) -> (w2182:string)
                          n1084 = Build Array(w2182) -> (w2185:string[])
                          n1085 = local write "ZMQ Reply"(w2185) -> ()
                          n1086 = Bundle(cluster=w2189, "Source"=Event_Sources."Send_ZMQ_Reply", "Command"="") -> (w2190:cluster{"Source":T16, "Command":string})
                          n1087 = Enqueue Element(queue=w2191, element=w2190) -> (error out=w2188:errorcluster)  [unwired: 2 in, 2 out]
                        }
                      }
                    }
                    frame Error {
                    }
                  }
                  n1088 = Less Than 0?(x=w2154) -> (x < 0?=w2153:bool)
                  n1089 = Or(x=w2153, y=w2141) -> (x .or. y?=w2144:bool)
                }
                n1090 = Build Array (concatenate)(w2126, w2117) -> (→"ZMQ Log":string[][])
                n1091 = call "Append to display log.vi"("string"="Receiving ZMQ message") -> ("error out"=w2139:errorcluster)  [unwired: 10 in]
                n1092 = call <vilib>:"Clear Errors.vi"("error in (no error)"=w2139) -> ()  [unwired: 5 in, 2 out]
              }
              event "Send ZMQ Reply": Value Change {
                w2352 = "}\u0000" ("delimiter (Tab)")
                # "show response on the ZMQ reply indicator"
                # "Log the ZMQ response"
                # "Strip contents before saving to log"
                # "'Send Multi-Part' blocks if there is no connection\n(not if the connected listener is not 'receive'ing)\nso poll for a connection first"
                n1093 = event-data() -> ()  [unwired: 1 in, 1 out]
                n1094 = Array To Spreadsheet String(delimiter (Tab)=",", array="ZMQ Reply", 3:"%s" ("delimiter (Tab)")) -> (spreadsheet string=w2355:string)
                n1095 = call <vilib>:"Trim Whitespace.vi"("string"=w2355) -> ("trimmed string"=w2310:string)  [unwired: 1 in]
                n1096 = Delete From Array(array="ZMQ Reply") -> (deleted portion=w2353:string, array with subset deleted=w2351:string[])  [unwired: 2 in]
                n1097 = call "Append to display log.vi"("string"="Sending ZMQ reply") -> ("error out"=w2359:errorcluster)  [unwired: 10 in]
                n1098 = call <vilib>:"Clear Errors.vi"("error in (no error)"=w2359) -> ()  [unwired: 5 in, 2 out]
                n1099 = Concatenate Strings(w2353, w2352) -> (w2350:string)
                n1100 = Concatenate Strings(w2310, w2352) -> (w2334:string)
                n1101 = Concatenate Strings(w2310, "}" ("delimiter (Tab)")) -> (w2312:string)
                n1102 = Build Array (concatenate)(w2351, w2350) -> (w2349:string[])
                n1103 = Build Array(w2334) -> (w2332:string[])
                n1104 = Match Pattern(string=w2312, regular expression="\"contents\":\"") -> (before substring=w2315:string, after substring=w2316:string, offset past match=w2313:i32)  [unwired: 1 in, 1 out]
                n1105 = local write "ZMQ Reply"(w2349) -> ()
                n1106 = Match Pattern(string=w2316, regular expression="\"") -> (after substring=w2314:string)  [unwired: 1 in, 3 out]
                n1107 = for {
                  N: 10 -> [_]
                  tunnel: [w2363] -> w2330
                  tunnel: [w2370] -> w2329
                  tunnel: w2328 -> [w2368]
                  stop <- w2365 continue-if-true
                  n1108 = Build Array(w2368) -> (w2372:refnum<class "zmq_socket.lvclass">[])
                  n1109 = call-poly <vilib>:"zmq_poll.vi"("timeout"=100, "poll type"=poll_type."Out", "sockets"=w2372) -> ("error out"=w2363:errorcluster, "polled events"=w2371:T25[])  [unwired: 1 in, 2 out]
                  n1110 = Unbundle(w2363) -> ("code"=w2362:i32)  [unwired: 2 out]
                  n1111 = Index Array(array=w2371) -> (element=w2370:T25)  [unwired: 1 in]
                  n1112 = Equal?(x=w2362, y=156384720 ("code")) -> (x = y?=w2365:bool)
                  n1113 = Wait (ms)(milliseconds to wait=u32 200) -> ()  [unwired: 1 out]
                }
                n1114 = Concatenate Strings(w2315, "\"contents\":\"[removed]\"" ("regular expression"), w2314) -> (w2320:string)
                n1115 = Less Than 0?(x=w2313) -> (x < 0?=w2321:bool)
                n1116 = Select(t=w2312, s=w2321, f=w2320) -> (s? t:f=w2311:string)
                n1117 = property on="Sending ZMQ" class="Bool (strict)"("Val(Sgnl)"=TRUE ("Value (Signaling)")) -> (error out=w2331:errorcluster)  [unwired: 2 in, 1 out]
                n1118 = local read "Current ZMQ Log"() -> (w2337:path)
                n1119 = Get Date/Time String(want seconds? (F)=TRUE) -> (date string=w2340:string, time string=w2341:string)  [unwired: 2 in]
                n1120 = local read "ZMQ Log"() -> (w2335:string[][])
                n1121 = call <vilib>:"Space Constant.vi"() -> ("String"=w2342:string)
                n1122 = call "get zmq message stats.vi"("message"=w2311, "error in"=w2331) -> ("Self Message"=w2324:bool, "msg_id"=w2347:string, "error out"=w2327:errorcluster)  [unwired: 8 in, 3 out]
                n1123 = Concatenate Strings(w2340, w2342, w2341) -> (w2344:string)
                n1124 = Build Array(w2344, w2347, w2311) -> (w2333:string[])
                n1125 = case shown="False" w2324 {
                  tunnel: [w2377 w2383] -> w2339
                  tunnel: w2332 -> [w2376 _]
                  tunnel: w2330 -> [w2375 w2383]
                  tunnel: w2329 -> [w2374 _]
                  tunnel: w2328 -> [w2373 _]
                  frame False {
                    n1126 = case shown="\"Out\", \"In/Out\"" w2374 {
                      tunnel: [w2381 w2382] -> w2377
                      tunnel: w2376 -> [w2380 _]
                      tunnel: w2373 -> [w2379 _]
                      tunnel: w2375 -> [w2378 w2382]
                      frame "Out", "In/Out" {
                        n1127 = call <vilib>:"zmq_send_multi.vi"("error in"=w2378, "parts"=w2380, "socket in"=w2379) -> ("error out"=w2381:errorcluster)  [unwired: 1 in, 1 out]
                      }
                      frame Default {
                        # "no listener\nDO NOT \nsend or it\n will block"
                      }
                    }
                  }
                  frame True {
                    # "self messages\nget the silent\ntreatment"
                  }
                }
                n1128 = call-poly <vilib>:"Write Delimited Spreadsheet.vi"("file path (dialog if empty)"=w2337, "1D data"=w2333, "append to file? (new file:F)"=TRUE ("append to file? (F)"), "delimiter (\\t)"="," ("delimiter (\\t)")) -> ("error out"=w2326:errorcluster)  [unwired: 10 in, 1 out]
                n1129 = Build Array (concatenate)(w2335, w2333) -> (w2336:string[][])
                n1130 = local write "ZMQ Log"(w2336) -> ()
                n1131 = Merge Errors(w2326, w2327) -> (w2325:errorcluster)
                n1132 = Merge Errors(w2339, w2325) -> (w2338:errorcluster)
              }
              event "ZMQ_PMT_Err": Value Change {
                # "Check whether the last action had any errors and if so, propagate them to the ZMQ reply"
                # "Name of PMT or Group\naction was on"
                n1133 = event-data() -> ("NewVal"=w2386:string)  [unwired: 1 in]
                n1134 = case shown="Error" w2385 {
                  selector: w2385 -> [_ w2395]
                  tunnel: w2386 -> [w2393 w2399]
                  tunnel: [w2392 w2398] -> w2387
                  tunnel: [w2391 w2397] -> _
                  frame No Error {
                    n1135 = Format Into String(format string="\"%s\":\"success\"" ("string"), w2393) -> (resulting string=w2392:string, error out=w2391:errorcluster)  [unwired: 2 in]
                  }
                  frame Error {
                    n1136 = Unbundle By Name(w2395) -> ("source"=w2394:string)
                    n1137 = Format Into String(format string="\"%s\":\"%s\"" ("string"), w2399, w2394) -> (resulting string=w2398:string, error out=w2397:errorcluster)  [unwired: 2 in]
                  }
                }
                n1138 = local read "ZMQ Reply"() -> (w2389:string[])
                n1139 = Build Array (concatenate)(w2389, w2387) -> (w2388:string[])
                n1140 = local write "ZMQ Reply"(w2388) -> ()
              }
              event "Manual ZMQ Write": Value Change {
                # "To send a message to ourselves we should open a separate connection to the port. We must close it immediately\nafter to prevent it intercepting messages sent from the DAQ. TODO: move this to a separate port, and set up a\nseparate internal listener on that port?"
                # "WE MUST CHECK SOMEONE IS LISTENING BEFORE SENDING ANY MESSAGES!"
                n1141 = event-data() -> ()  [unwired: 1 in, 1 out]
                n1142 = case shown="True" "Send to Self" {
                  selector: "Send to Self" -> [_ w2433]
                  tunnel: w2409 -> [w2427 _]
                  tunnel: [w2427 w2439] -> w2402
                  tunnel: w2408 -> [_ w2444]
                  tunnel: [_ w2434] -> w2407
                  tunnel: [_ w2433] -> w2406
                  tunnel: "ZMQ Message" -> [w2426 w2429]
                  tunnel: [w2426 w2428] -> w2400
                  frame False {
                  }
                  frame True {
                    # "replace msg_ids with -999: indiicate as from self"
                    # "replace endpoint from\n tcp://*:port to tcp://localhost:port"
                    n1143 = local read "ZMQ endpoint"() -> (w2432:string)
                    n1144 = for {
                      tunnel: w2429 -> [w2449] mode=indexing
                      tunnel: [w2448] -> w2428 mode=indexing
                      w2447 = TRUE ("ignore case? (F)")
                      n1145 = Search and Replace String(replace all?=w2447, case sensitive?=w2447, input string=w2449, search string="\"msg_id\" *: *\"[^\"]+\"", replace string="\"msg_id\" : \"-999\"" ("search string")) -> (result string=w2448:string)  [unwired: 3 in, 3 out]
                    }
                    n1146 = xnode "Match Regular Expression"("input string"=w2432, "regular expression"="tcp://[^:]+:([0-9]+)") -> ("error out"=w2442:errorcluster, "submatch 1"=w2443:string)  [unwired: 4 in, 4 out]
                    n1147 = Format Into String(format string="tcp://127.0.0.1:%s" ("regular expression"), error in=w2442, w2443) -> (resulting string=w2436:string, error out=w2435:errorcluster)  [unwired: 1 in]
                    n1148 = call <vilib>:"zmq_socket.vi"("error in"=w2435, "linger (ms)"=100 ("timeout"), "socket type"=socket_type."ZMQ_DEALER", "context in"=w2444) -> ("error out"=w2437:errorcluster, "socket out"=w2438:refnum<class "zmq_socket.lvclass">)  [unwired: 1 in, 1 out]
                    n1149 = call <vilib>:"zmq_connect.vi"("error in"=w2437, "endpoint"=w2436, "socket in"=w2438) -> ("error out"=w2434:errorcluster, "socket out"=w2439:refnum<class "zmq_socket.lvclass">)  [unwired: 1 in]
                  }
                }
                n1150 = local write "Manual ZMQ Write"(FALSE ("Manual ZMQ Write")) -> ()
                n1151 = Build Array(w2402) -> (w2416:refnum<class "zmq_socket.lvclass">[])
                n1152 = call-poly <vilib>:"zmq_poll.vi"("error in"=w2407, "timeout"=100, "poll type"=poll_type."In/Out", "sockets"=w2416) -> ("error out"=w2411:errorcluster, "polled events"=w2415:T25[])  [unwired: 2 out]
                n1153 = Index Array(array=w2415) -> (element=w2412:T25)  [unwired: 1 in]
                n1154 = case shown="Default" w2412 {
                  tunnel: [errorcluster {"status"=FALSE, "code"=0, "source"="Manual ZMQ write not performed; no listeners\n(write would block until a listener became available!)"} ("error out") w2575] -> w2404
                  tunnel: w2411 -> [_ w2571]
                  tunnel: [w2566 w2570] -> w2403
                  tunnel: w2402 -> [w2566 w2569]
                  tunnel: w2400 -> [_ w2568]
                  frame "None" {
                  }
                  frame Default {
                    n1155 = for {
                      tunnel: w2568 -> [w2578] mode=indexing
                      tunnel: [w2576] -> w2572 mode=indexing
                      n1156 = Concatenate Strings(w2578, "\u0000" ("string")) -> (w2576:string)
                    }
                    n1157 = property on="Sending ZMQ" class="Bool (strict)"(error in=w2571, "Val(Sgnl)"=TRUE ("Value (Signaling)")) -> (error out=w2573:errorcluster)  [unwired: 1 in, 1 out]
                    n1158 = call <vilib>:"zmq_send_multi.vi"("error in"=w2573, "parts"=w2572, "socket in"=w2569) -> ("error out"=w2575:errorcluster, "socket out"=w2570:refnum<class "zmq_socket.lvclass">)  [unwired: 1 in]
                  }
                }
                n1159 = call "Append to display log.vi"("string"="Sending manual ZMQ message") -> ("error out"=w2420:errorcluster)  [unwired: 10 in]
                n1160 = case shown="True" w2406 {
                  tunnel: [w2422 w2424] -> w2405
                  tunnel: w2404 -> [w2422 w2425]
                  tunnel: w2403 -> [_ w2423]
                  frame False {
                  }
                  frame True {
                    n1161 = call <vilib>:"zmq_close.vi"("error in"=w2425, "socket"=w2423) -> ("error out"=w2424:errorcluster)  [unwired: 3 in]
                  }
                }
                n1162 = call <vilib>:"Clear Errors.vi"("error in (no error)"=w2420) -> ()  [unwired: 5 in, 2 out]
              }
              event "Show Group In Displayed Channels": Value Change {
                # "show only active subset"
                n1163 = event-data() -> ()  [unwired: 1 in, 2 out]
                n1164 = global read "CAEN globals.vi" "Groups"() -> (w2602:T19)
                n1165 = local read "Group"() -> (w2579:string)
                n1166 = for {
                  tunnel: w2602 -> [w2634] mode=indexing
                  tunnel: [w2632] -> w2604
                  tunnel: [w2631] -> w2601
                  tunnel: w2579 -> [w2630]
                  stop <- w2632 stop-if-true
                  n1167 = Unbundle By Name(w2634) -> ("Channels in Group"=w2631:T3[], "Group Name"=w2633:string)
                  n1168 = Equal?(x=w2633, y=w2630) -> (x = y?=w2632:bool)
                }
                n1169 = Format Into String(format string="group \"%s\" not in group list" ("string"), w2579) -> (resulting string=w2585:string, error out=w2583:errorcluster)  [unwired: 2 in]
                n1170 = local write "Show Group In Displayed Channels"(FALSE ("MRD")) -> ()
                n1171 = Bundle By Name(cluster=errorcluster {"status"=TRUE, "code"=0, "source"=""} ("error out"), "source"=w2585) -> (w2584:errorcluster)
                n1172 = Format Into String(format string="Filtering view to %s only" ("string"), error in=w2583, w2579) -> (resulting string=w2589:string, error out=w2588:errorcluster)  [unwired: 1 in]
                n1173 = for {
                  tunnel: w2601 -> [w2625] mode=indexing
                  tunnel: [w2627] -> w2599 mode=indexing
                  tunnel: [w2626] -> w2600 mode=indexing
                  tunnel: [w2623] -> w2592 mode=indexing
                  n1174 = Unbundle By Name(w2625) -> ("Crate"=w2623:i32, "Card.Channel"=w2624:dbl)
                  n1175 = Quotient & Remainder(x=w2624, y=1.0) -> (x-y*floor(x/y)=w2628:dbl, floor(x/y)=w2627:dbl)
                  n1176 = expression code="x*100"(w2628) -> (w2626:dbl)
                }
                n1177 = call "Append to display log.vi"("error in"=w2588, "string"=w2589) -> ("error out"=w2593:errorcluster)  [unwired: 9 in]
                n1178 = Select(t=errorcluster {"status"=FALSE, "code"=0, "source"=""} ("error in"), s=w2604, f=w2584) -> (s? t:f=w2598:errorcluster)
                n1179 = call <vilib>:"Clear Errors.vi"("error in (no error)"=w2593) -> ()  [unwired: 5 in, 2 out]
                n1180 = global read "CAEN globals.vi" "Channel Array Val"() -> (w2596:T8[])
                n1181 = for {
                  tunnel: w2600 -> [w2619] mode=indexing
                  tunnel: w2599 -> [w2620] mode=indexing
                  shift-right: [w2621] -> w2597
                  shift-left: w2598 -> [w2622]
                  tunnel: [w2617] -> w2581 mode=indexing
                  tunnel: w2592 -> [w2618] mode=indexing
                  tunnel: [w2616] -> _
                  tunnel: [w2615] -> w2582 mode=indexing
                  i -> [w2616]
                  n1182 = call "convert rel chan num.vi"("error in"=w2622, "Card"=w2620, "Channel"=w2619, "Crate"=w2618) -> ("error out"=w2621:errorcluster, "Absolute index"=w2617:i32, "ACTIVE index"=w2615:i32)  [unwired: 4 in, 1 out]
                }
                n1183 = case shown="\"GROUP00\"" w2579 {
                  tunnel: w2582 -> [_ w2611]
                  tunnel: w2581 -> [w2606 w2609]
                  tunnel: [w2606 w2607] -> w2580
                  frame "GROUP00" {
                  }
                  frame Default {
                    n1184 = call-poly <userlib>:"Filter 1D Array__ogtk.vi"("items to filter"=-1 ("Crate"), "array"=w2611) -> ("filtered item indices"=w2608:i32[])  [unwired: 4 in, 1 out]
                    n1185 = call-poly <userlib>:"Delete Elements from Array__ogtk.vi"("indices"=w2608, "array"=w2609) -> ("array w/ subset deleted"=w2607:i32[])  [unwired: 8 in, 1 out]
                  }
                }
                n1186 = for {
                  tunnel: w2596 -> [w2614]
                  tunnel: w2580 -> [w2613] mode=indexing
                  tunnel: [w2612] -> w2595 mode=indexing
                  n1187 = Index Array(array=w2614, index=w2613) -> (element=w2612:T8)
                }
                n1188 = global write "CAEN globals.vi" "Visible Channels"(w2580) -> ()
                n1189 = local write "Channel Array"(w2595) -> ()
              }
              event "Add Group to Displayed Channels": Value Change {
                n1190 = event-data() -> ()  [unwired: 1 in, 6 out]
                n1191 = global read "CAEN globals.vi" "Groups"() -> (w2654:T19)
                n1192 = local read "Group"() -> (w2640:string)
                n1193 = for {
                  tunnel: w2654 -> [w2683] mode=indexing
                  tunnel: [w2681] -> w2655
                  tunnel: [w2680] -> w2653
                  tunnel: w2640 -> [w2679]
                  stop <- w2681 stop-if-true
                  n1194 = Unbundle By Name(w2683) -> ("Channels in Group"=w2680:T3[], "Group Name"=w2682:string)
                  n1195 = Equal?(x=w2682, y=w2679) -> (x = y?=w2681:bool)
                }
                n1196 = Format Into String(format string="group \"%s\" not in group list" ("string"), w2640) -> (resulting string=w2643:string, error out=w2641:errorcluster)  [unwired: 2 in]
                n1197 = local write "Add Group to Displayed Channels"(FALSE ("MRD")) -> ()
                n1198 = Bundle By Name(cluster=errorcluster {"status"=TRUE, "code"=0, "source"=""} ("error out"), "source"=w2643) -> (w2642:errorcluster)
                n1199 = Format Into String(format string="Filtering view to %s only" ("string"), error in=w2641, w2640) -> (resulting string=w2645:string, error out=w2644:errorcluster)  [unwired: 1 in]
                n1200 = for {
                  tunnel: w2653 -> [w2674] mode=indexing
                  tunnel: [w2676] -> w2651 mode=indexing
                  tunnel: [w2675] -> w2652 mode=indexing
                  tunnel: [w2672] -> w2646 mode=indexing
                  n1201 = Unbundle By Name(w2674) -> ("Crate"=w2672:i32, "Card.Channel"=w2673:dbl)
                  n1202 = Quotient & Remainder(x=w2673, y=1.0) -> (x-y*floor(x/y)=w2677:dbl, floor(x/y)=w2676:dbl)
                  n1203 = expression code="x*100"(w2677) -> (w2675:dbl)
                }
                n1204 = call "Append to display log.vi"("error in"=w2644, "string"=w2645) -> ("error out"=w2647:errorcluster)  [unwired: 9 in]
                n1205 = Select(t=errorcluster {"status"=FALSE, "code"=0, "source"=""} ("error in"), s=w2655, f=w2642) -> (s? t:f=w2650:errorcluster)
                n1206 = call <vilib>:"Clear Errors.vi"("error in (no error)"=w2647) -> ()  [unwired: 5 in, 2 out]
                n1207 = global read "CAEN globals.vi" "Visible Channels"() -> (w2657:i32[])
                n1208 = global read "CAEN globals.vi" "Channel Array Val"() -> (w2649:T8[])
                n1209 = for {
                  tunnel: w2652 -> [w2667] mode=indexing
                  tunnel: w2651 -> [w2668] mode=indexing
                  shift-right: [w2670] -> w2635
                  shift-left: w2650 -> [w2671]
                  tunnel: [w2669] -> w2658 mode=indexing
                  tunnel: w2646 -> [w2666] mode=indexing
                  n1210 = call "convert rel chan num.vi"("error in"=w2671, "Card"=w2668, "Channel"=w2667, "Crate"=w2666) -> ("error out"=w2670:errorcluster, "ACTIVE index"=w2669:i32)  [unwired: 4 in, 2 out]
                }
                n1211 = Build Array (concatenate)(w2658, w2657) -> (w2656:i32[])
                n1212 = call-poly <userlib>:"Remove Duplicates from 1D Array__ogtk.vi"("Input Array"=w2656) -> ("Output Array"=w2659:i32[])  [unwired: 1 out]
                n1213 = global write "CAEN globals.vi" "Visible Channels"(w2659) -> ()
                n1214 = for {
                  tunnel: w2649 -> [w2665]
                  tunnel: w2659 -> [w2664] mode=indexing
                  tunnel: [w2663] -> w2648 mode=indexing
                  n1215 = Index Array(array=w2665, index=w2664) -> (element=w2663:T8)
                }
                n1216 = local write "Channel Array"(w2648) -> ()
              }
              event Value Change {
                n1217 = event-data() -> ("NewVal"=w2703:T5)  [unwired: 1 in]
                n1218 = control-ref of="This VI"() -> (w2692:refnum<vi>)
                n1219 = Equal?(x=w2703, y=tabs."Screen Emulation" ("NewVal")) -> (x = y?=w2691:bool)
                n1220 = Select(t=w2692, s=w2691, f=refnum<vi> refnum ("vi reference")) -> (s? t:f=w2687:refnum<vi>)
                n1221 = register-events(reference=w2689, w2687, w2686) -> (reference out=w2693:refnum<event-registration>, error out=w2688:errorcluster)  [unwired: 1 in]
                n1222 = control-ref of="This VI"() -> (w2699:refnum<vi>)
                n1223 = property class="VI"(reference=w2699, error in=w2688) -> (error out=w2700:errorcluster, "Panel"=w2701:refnum<vi>)  [unwired: 1 out]
                n1224 = property class="Pnl"(reference=w2701, error in=w2700) -> (error out=w2698:errorcluster, "Decos[]"=w2702:refnum<vi>[])  [unwired: 1 out]
                n1225 = Index Array(array=w2702) -> (element #1=w2695:refnum<vi>, element #2=w2694:refnum<vi>)  [unwired: 2 in]
                n1226 = property class="Decor"(reference=w2695, error in=w2698, "Visible"=w2691) -> (error out=w2697:errorcluster)  [unwired: 1 out]
                n1227 = property class="Decor"(reference=w2694, error in=w2697, "Visible"=w2691) -> (error out=w2696:errorcluster)  [unwired: 1 out]
              }
              event "Show hidden tabs": Value Change {
                # "hide array version of display - only really\nset up to work with display screen."
                n1228 = event-data() -> ("NewVal"=w2708:bool)  [unwired: 1 in]
                n1229 = property on="Tab Control" class="TabCtl (strict)"() -> ("Pages"=w2709:refnum<vi>[])  [unwired: 2 in, 2 out]
                n1230 = Index Array(array=w2709, index=3) -> (element=w2710:refnum<vi>)
                n1231 = property class="Page"(reference=w2710, "PageVis"=w2708) -> (error out=w2706:errorcluster)  [unwired: 1 in, 1 out]
              }
              event "'\\' codes display": Value Change {
                n1232 = event-data() -> ("NewVal"=w2715:bool)  [unwired: 1 in]
                n1233 = Select(t=u32 1 ("Display Style"), s=w2715, f=u32 0 ("Display Style")) -> (s? t:f=w2714:u32)
                n1234 = property on="Read buffer CAEN" class="Str"("Display Style"=w2714) -> (error out=w2713:errorcluster)  [unwired: 2 in, 1 out]
              }
              event "Line Wrapping": Value Change {
                n1235 = event-data() -> ("NewVal"=w2720:bool)  [unwired: 1 in]
                n1236 = property on="Read buffer CAEN" class="Str"("WrappingEnabled"=w2720) -> (error out=w2721:errorcluster)  [unwired: 2 in, 1 out]
              }
              event "stop": Value Change {
                n1237 = event-data() -> ()  [unwired: 1 in, 1 out]
                n1238 = local read "error out"() -> (w2725:errorcluster)
              }
            }
          }
          frame Error {
            n1239 = for {
              N: 1 -> [_]
              tunnel: w2731 -> [w2741]
              tunnel: [w2738] -> w2730
              tunnel: w2729 -> [w2737]
              tunnel: [w2736] -> w2728
              shift-right: [w2735] -> _
              shift-left: _ -> [w2734]
              i -> [w2739]
              stop <- w2740 continue-if-true
              n1240 = case shown="0" w2739 {
                tunnel: w2741 -> [_ w2824]
                tunnel: [_ w2773] -> w2740
                tunnel: [w2744 w2776] -> w2738
                tunnel: w2737 -> [w2743 w2777]
                tunnel: [w2745 _] -> w2736
                tunnel: [_ w2778] -> _
                tunnel: [_ w2772] -> w2735
                tunnel: w2734 -> [w2742 _]
                frame Default {
                  # "NOTE: DISABLED BY LOOP RANGE\nwould only work if error was on \nCAEN: probably not useful anyway"
                  n1241 = case shown="True" w2742 {
                    tunnel: [w2747 w2753] -> w2745
                    tunnel: [w2746 w2752] -> w2744
                    tunnel: w2743 -> [w2748 w2750]
                    frame False {
                      n1242 = VISA Flush I/O Buffer(VISA resource name=w2748) -> (VISA resource name out=w2746:refnum<visa-resource-name>, error out=w2747:errorcluster)  [unwired: 2 in]
                    }
                    frame True {
                      n1243 = VISA Close(VISA resource name=w2750) -> (error out=w2754:errorcluster)  [unwired: 1 in]
                      n1244 = call <vilib>:"Clear Errors.vi"("error in (no error)"=w2754) -> ("error out"=w2749:errorcluster)  [unwired: 5 in, 1 out]
                      n1245 = local read "CAEN Serial Port"() -> (w2751:i32)
                      n1246 = Format Into String(format string="ASRL%d::INSTR" ("write buffer"), error in=w2749, w2751) -> (resulting string=w2761:string, error out=w2758:errorcluster)  [unwired: 1 in]
                      n1247 = VISA Open(error in (no error)=w2758, VISA resource name=w2761) -> (VISA resource name=w2755:refnum<visa-resource-name>, error out=w2756:errorcluster)  [unwired: 3 in]
                      n1248 = call-poly "VISA Configure Serial Port"("VISA resource name"=w2755, "Enable Termination\nChar (T)"=FALSE ("Enable Termination\nChar (T)"), "baud rate (9600)"=u32 19200, "error in (no error)"=w2756) -> ("VISA resource name out"=w2752:refnum<visa-resource-name>, "error out"=w2753:errorcluster)  [unwired: 10 in]
                    }
                  }
                }
                frame 0 {
                  w2823 = T30 0 items=["no dialog", "OK message", "continue or stop message", "OK message + warnings", "continue/stop + warnings"] ("type of dialog (OK msg:1)")
                  # "write headers if this is a new file"
                  n1249 = global read "CAEN globals.vi" "Error Display String"() -> (w2765:string)
                  n1250 = local read "Alarm Screencap"() -> (w2767:string)
                  n1251 = global read "CAEN globals.vi" "Error Screencap"() -> (w2788:string[][])
                  n1252 = local write "error out"(w2824) -> ()
                  n1253 = local read "Current Error Log"() -> (w2814:path)
                  n1254 = Unbundle By Name(w2824) -> ("code"=w2780:i32, "source"=w2764:string)
                  n1255 = Empty String/Path?(string/path=w2767) -> (empty?=w2768:bool)
                  n1256 = Search and Replace String(replace all?=TRUE ("want seconds? (F)"), input string=w2765, search string="\t") -> (result string=w2766:string)  [unwired: 5 in, 3 out]
                  n1257 = Select(t=w2766, s=w2768, f=w2767) -> (s? t:f=w2769:string)
                  n1258 = Get File Size(file=w2814) -> (refnum out=w2796:refnum<file>, size (in bytes)=w2800:i64, 0:w2799:errorcluster)  [unwired: 1 in]
                  n1259 = global read "CAEN globals.vi" "Selection Position"() -> (w2805:cluster{i32, i32})
                  n1260 = local write "Alarm Screencap"(w2769) -> ()
                  n1261 = global read "CAEN globals.vi" "Error Read"() -> (w2786:string)
                  n1262 = Close File(refnum=w2796, error in=w2799) -> (path=w2797:path, error out=w2798:errorcluster)
                  n1263 = Array To Spreadsheet String(delimiter (Tab)=",", array=w2788, 3:"%s" ("delimiter (Tab)")) -> (spreadsheet string=w2787:string)
                  n1264 = case shown="Default" w2800 {
                    tunnel: [w2950 w2952] -> w2819
                    tunnel: [w2949 w2951] -> w2820
                    tunnel: w2798 -> [w2948 w2951]
                    tunnel: w2797 -> [w2947 w2952]
                    tunnel: string[] ["Timestamp", "Error Code", "Error Source", "Display at Time of Error", "Last Read", "Selection Position"] ("subarray") -> [w2946 _]
                    frame 0 {
                      n1265 = call-poly <vilib>:"Write Delimited Spreadsheet.vi"("file path (dialog if empty)"=w2947, "1D data"=w2946, "error in (no error)"=w2948) -> ("new file path (Not A Path if cancelled)"=w2950:path, "error out"=w2949:errorcluster)  [unwired: 11 in]
                    }
                    frame Default {
                    }
                  }
                  n1266 = Get Date/Time String(want seconds? (F)=TRUE) -> (date string=w2809:string, time string=w2812:string)  [unwired: 2 in]
                  n1267 = call "make subs for logging.vi"("spreadsheet string"=w2787) -> ("error out"=w2784:errorcluster, "trimmed string"=w2808:string)  [unwired: 9 in]
                  n1268 = call "make subs for logging.vi"("spreadsheet string"=w2786) -> ("error out"=w2785:errorcluster, "trimmed string"=w2782:string)  [unwired: 9 in]
                  n1269 = Unbundle(w2805) -> (w2804:i32, w2803:i32)
                  n1270 = call <vilib>:"Space Constant.vi"() -> ("String"=w2811:string)
                  n1271 = Concatenate Strings(w2809, w2811, w2812) -> (w2762:string)
                  "Error Timestamp" <- w2762
                  n1272 = Number To Decimal String(number=w2780) -> (decimal integer string=w2807:string)  [unwired: 1 in]
                  n1273 = Merge Errors(w2784, w2785) -> (w2783:errorcluster)
                  n1274 = Format Into String(w2804, w2803) -> (resulting string=w2781:string, error out=w2802:errorcluster)  [unwired: 3 in]
                  n1275 = local write "Screencap Timestamp"(w2762) -> ()
                  n1276 = Merge Errors(w2783, w2802) -> (w2801:errorcluster)
                  n1277 = xnode "Match Regular Expression"("input string"=w2764, "regular expression"="VISA Write|VISA Enable" ("source"), "ignore case? (F)"=TRUE) -> ("offset past match"=w2790:i32)  [unwired: 3 in, 4 out]
                  n1278 = Build Array(w2762, w2807, w2764, w2808, w2782, w2781) -> (w2813:string[])
                  n1279 = Build Array(w2762, w2807, w2764) -> (w2795:string[])
                  n1280 = Greater Or Equal To 0?(x=w2790) -> (x >= 0?=w2772:bool)
                  n1281 = Equal?(x=-1073807253, y=w2780) -> (x = y?=w2774:bool)
                  n1282 = call <vilib>:"Find First Error.vi"("error in (no error)"=w2801) -> ()  [unwired: 3 in, 2 out]
                  n1283 = Array To Spreadsheet String(delimiter (Tab)=", " ("format string"), array=w2795, 3:"%s" ("format string")) -> (spreadsheet string=w2792:string)
                  n1284 = call-poly <vilib>:"Write Delimited Spreadsheet.vi"("file path (dialog if empty)"=w2819, "1D data"=w2813, "append to file? (new file:F)"=TRUE ("append to file? (F)"), "error in (no error)"=w2820) -> ("error out"=w2822:errorcluster)  [unwired: 10 in, 1 out]
                  n1285 = disable-structure shown="Enabled" {
                    disable-tunnel: [w2827 _] -> w2778
                    disable-tunnel: w2777 -> [w2826 w2831]
                    disable-tunnel: [w2825 w2831] -> w2776
                    frame Disabled {
                      n1286 = VISA Write(VISA resource name=w2826, write buffer="\nQ" ("delimiter (Tab)")) -> (VISA resource name out=w2828:refnum<visa-resource-name>, error out=w2829:errorcluster)  [unwired: 1 in, 1 out]
                      n1287 = call "read caen.vi"("VISA in"=w2828, "error in"=w2829) -> ("VISA out"=w2825:refnum<visa-resource-name>, "error out"=w2827:errorcluster)  [unwired: 8 in, 4 out]
                    }
                    frame Enabled {
                    }
                  }
                  n1288 = Or(x=w2772, y=w2774) -> (x .or. y?=w2773:bool)
                  n1289 = local write "summary status"(w2792) -> ()
                  n1290 = local write "Status message"(w2792) -> ()
                  n1291 = feedback #5() -> (w2818:string[][])  [unwired: 1 in]
                  n1292 = Build Array (concatenate)(w2818, w2795) -> (w2817:string[][])
                  n1293 = Delete From Array(array=w2817, length=100) -> (deleted portion=w2815:string[][])  [unwired: 2 in, 1 out]
                  "Error Log" <- w2815
                  n1294 = feedback-in #5(w2815) -> ()
                  n1295 = call <vilib>:"General Error Handler.vi"("type of dialog (OK msg:1)"=w2823, "error in (no error)"=w2822) -> ()  [unwired: 9 in, 5 out]
                }
              }
            }
          }
        }
        n1296 = Not(x=w350) -> (.not. x?=w349:bool)
        "hb" <- w349
        n1297 = local read "slack"() -> (w326:T1)
      }
    }
    frame Error {
      n1298 = call <userlib>:"Wait (ms)__ogtk.vi"("milliseconds to wait"=u32 1000) -> ("error out"=w2954:errorcluster)  [unwired: 9 in, 1 out]
      n1299 = call <vilib>:"Simple Error Handler.vi"("error in (no error)"=w2959) -> ("error out"=w2958:errorcluster)  [unwired: 4 in, 4 out]
      n1300 = property on="stop" class="Bool (strict)"(error in=w2954, "Val(Sgnl)"=TRUE ("Value (Signaling)")) -> (error out=w2955:errorcluster)  [unwired: 1 in, 1 out]
      n1301 = flat-sequence {
        tunnel: "Initialization Error: Check power to crates" ("message") -> [w2966]
        tunnel: w2958 -> [_]
        frame #0 {
          n1302 = One Button Dialog(message=w2966) -> ()  [unwired: 1 in, 1 out]
        }
      }
      n1303 = call <vilib>:"Clear Errors.vi"("error in (no error)"=w2955) -> ()  [unwired: 5 in, 2 out]
      n1304 = local read "slack"() -> (w2957:T1)
    }
  }
  n1305 = case shown="No Error" w7 {
    tunnel: [w2967 _] -> w12
    frame No Error {
      n1306 = while {
        tunnel: [w2968] -> w2967
        stop <- w2969 stop-if-true
        n1307 = event shown="[0] \"Do L2 Page Read\": Value Change" {
          selector: _ -> [_ _]
          dyn-events: _ -> [_ _]
          timeout: _ -> [_ _]
          tunnel: [_ w3066] -> w2969
          tunnel: [w2970 _] -> w2968
          tunnel: [w2973 _] -> _
          event "Do L2 Page Read": Value Change {
            w2971 = 2  # Crate
            n1308 = event-data() -> ()  [unwired: 1 in, 1 out]
            n1309 = property on="Reading LeCroy2 Page" class="Bool (strict)"("Value"=TRUE ("Reading LeCroy2 Page")) -> (error out=w2972:errorcluster)  [unwired: 2 in, 1 out]
            n1310 = for {
              N: 3 -> [_]
              tunnel: [w2983] -> w2970
              tunnel: "Do L2 Page Read" -> [w2984]
              tunnel: w2972 -> [w2993]
              tunnel: w2971 -> [w2992]
              tunnel: [w2982] -> w2974
              stop <- w2995 continue-if-true
              n1311 = local read "Kill All"() -> (w2997:bool)
              n1312 = local read "Log to File"() -> (w2991:bool)
              n1313 = local read "stop"() -> (w2996:bool)
              n1314 = call "read channel page lecroy.vi"("Crate"=w2992, "page"=w2984, "error in"=w2993) -> ("VISA out"=w2998:refnum<visa-resource-name>, "New Channels"=w2987:T8[], "Start Index in ACTIVE"=w2985:i32, "error out"=w2994:errorcluster)  [unwired: 8 in, 1 out]
              n1315 = Compound Arithmetic op=AND(invert w2997, invert w2996, w2994) -> (w2995:bool)
              n1316 = case shown="No Error" w2994 {
                selector: w2994 -> [_ w3052]
                tunnel: [w3018 w3051] -> w3007
                tunnel: [w3017 _] -> w3006
                tunnel: [w3016 _] -> w3005
                tunnel: [w3015 _] -> w3004
                tunnel: [w3014 _] -> w3003
                tunnel: w2991 -> [w3013 _]
                tunnel: [w3012 _] -> w3002
                tunnel: [w3011 _] -> w3001
                tunnel: [w3010 _] -> w3000
                tunnel: w2987 -> [w3009 _]
                tunnel: [w3008 _] -> w2999
                tunnel: w2998 -> [_ w3050]
                frame No Error {
                  n1317 = for {
                    tunnel: w3009 -> [w3023] mode=indexing
                    tunnel: [w3040] -> w3018 mode=indexing
                    tunnel: [w3031] -> w3017 mode=indexing
                    tunnel: [w3038] -> w3016 mode=indexing
                    tunnel: [w3037] -> w3015 mode=indexing
                    tunnel: [w3036] -> w3014 mode=indexing
                    tunnel: w3013 -> [w3035]
                    tunnel: [w3032] -> w3012 mode=indexing
                    tunnel: [w3019] -> w3010
                    tunnel: [w3030] -> w3011 mode=indexing
                    tunnel: [TRUE ("append to file? (F)")] -> w3008
                    n1318 = Unbundle By Name(w3023) -> ("Timestamp"=w3034:string, "Vmon (V)"=w3031:dbl, "Vset (V)"=w3038:dbl, "Imon (A)"=w3037:dbl, "Iset (A)"=w3036:dbl, "Crate"=w3029:i32, "Card"=w3028:i32, "Channel"=w3027:i32)
                    n1319 = local read "Current Channel Log"() -> (w3025:path)
                    n1320 = Format Into String(format string="Monitoring_Log_%d-%d-%d.csv" ("string"), w3029, w3028, w3027) -> (resulting string=w3026:string, error out=w3020:errorcluster)  [unwired: 2 in]
                    n1321 = call "channel cluster to array.vi"("input cluster"=w3023) -> ("Array"=w3039:string[])  [unwired: 10 in]
                    n1322 = call-poly "Timestamp String to LV Timestamp Poly.vi"("Timestamp String"=w3034) -> ("Y M D H M S Array"=w3030:i32[], "Timestamp"=w3033:timestamp)
                    n1323 = Build Path(base path=w3025, name or relative path=w3026) -> (appended path=w3041:path)
                    n1324 = To Double Precision Float(number=w3033) -> (double precision float=w3032:dbl)
                    n1325 = local read "History Length"() -> (w3019:i32)
                    n1326 = case shown="True" w3035 {
                      tunnel: w3041 -> [_ w3047]
                      tunnel: [_ w3046] -> w3040
                      tunnel: w3039 -> [_ w3045]
                      tunnel: w3020 -> [_ w3043]
                      tunnel: TRUE ("append to file? (F)") -> [_ w3042]
                      frame False {
                      }
                      frame True {
                        n1327 = call-poly <vilib>:"Write Delimited Spreadsheet.vi"("file path (dialog if empty)"=w3047, "1D data"=w3045, "append to file? (new file:F)"=w3042, "error in (no error)"=w3043, "delimiter (\\t)"="," ("delimiter (\\t)")) -> ("error out"=w3046:errorcluster)  [unwired: 9 in, 1 out]
                      }
                    }
                  }
                }
                frame Error {
                  n1328 = Wait (ms)(milliseconds to wait=u32 1000) -> ()  [unwired: 1 out]
                  n1329 = VISA Flush I/O Buffer(VISA resource name=w3050) -> (error out=w3049:errorcluster)  [unwired: 2 in, 1 out]
                  n1330 = Build Array(w3052, w3049) -> (w3051:errorcluster[])
                }
              }
              n1331 = case shown="False" w2999 {
                tunnel: w3006 -> [_ w3059]
                tunnel: w3005 -> [_ w3060]
                tunnel: w3004 -> [_ w3061]
                tunnel: w3003 -> [_ w3062]
                tunnel: w3002 -> [_ w3058]
                tunnel: w3001 -> [_ w3065]
                tunnel: w3000 -> [_ w3064]
                tunnel: w2985 -> [_ w3063]
                frame False {
                }
                frame True {
                  w3053 = history_array_type."Iset" ("Log")
                  w3054 = history_array_type."Imon" ("Log")
                  w3055 = history_array_type."Vset" ("Log")
                  w3056 = history_array_type."Vmon" ("Log")
                  w3057 = history_array_type."TimeStamp" ("Log")
                  n1332 = call-poly "buffer array poly.vi"("Array"=w3065, "History length"=w3064, "Start channel"=w3063) -> ()  [unwired: 17 in]
                  n1333 = call "buffer array 1D.vi"("Array"=w3058, "History length"=w3064, "Log"=w3057, "Start channel"=w3063) -> ()  [unwired: 16 in]
                  n1334 = call "buffer array 1D.vi"("Array"=w3059, "History length"=w3064, "Log"=w3056, "Start channel"=w3063) -> ()  [unwired: 16 in]
                  n1335 = call "buffer array 1D.vi"("Array"=w3060, "History length"=w3064, "Log"=w3055, "Start channel"=w3063) -> ()  [unwired: 16 in]
                  n1336 = call "buffer array 1D.vi"("Array"=w3061, "History length"=w3064, "Log"=w3054, "Start channel"=w3063) -> ()  [unwired: 16 in]
                  n1337 = call "buffer array 1D.vi"("Array"=w3062, "History length"=w3064, "Log"=w3053, "Start channel"=w3063) -> ()  [unwired: 16 in]
                  n1338 = call-poly "buffer array poly.vi"("Array"=w3058, "History length"=w3064, "Log"=w3057, "Start channel"=w3063) -> ()  [unwired: 16 in]
                  n1339 = call-poly "buffer array poly.vi"("Array"=w3059, "History length"=w3064, "Log"=w3056, "Start channel"=w3063) -> ()  [unwired: 16 in]
                  n1340 = call-poly "buffer array poly.vi"("Array"=w3060, "History length"=w3064, "Log"=w3055, "Start channel"=w3063) -> ()  [unwired: 16 in]
                  n1341 = call-poly "buffer array poly.vi"("Array"=w3061, "History length"=w3064, "Log"=w3054, "Start channel"=w3063) -> ()  [unwired: 16 in]
                  n1342 = call-poly "buffer array poly.vi"("Array"=w3062, "History length"=w3064, "Log"=w3053, "Start channel"=w3063) -> ()  [unwired: 16 in]
                }
              }
              n1343 = Merge Errors(w3007) -> (w2986:errorcluster)
              n1344 = Array Size(array=w2987) -> (size(s)=w2990:i32)
              n1345 = Bundle(cluster=T2 {"Start Index"=0, "Num Channels Read"=0} ("Value (Signaling)"), "Start Index"=w2985, "Num Channels Read"=w2990) -> (w2989:T2)
              n1346 = property on="Update Plots & Alarms" class="Clust (strict)"(error in=w2986, "Val(Sgnl)"=w2989) -> (error out=w2983:errorcluster)  [unwired: 1 in, 1 out]
              n1347 = call <vilib>:"Clear Errors.vi"("error in (no error)"=w2983) -> ("error out"=w2982:errorcluster)  [unwired: 5 in, 1 out]
            }
            n1348 = case shown="Error" w2970 {
              selector: w2970 -> [_ w2979]
              tunnel: w2971 -> [_ w2980]
              frame No Error {
              }
              frame Error {
                n1349 = Bundle("Crate"=w2980, "error IO"=w2979) -> (w2981:cluster{"Crate":i32, "error IO":errorcluster})  [unwired: 1 in]
                n1350 = property on="read error" class="Clust (strict)"("Val(Sgnl)"=w2981) -> ()  [unwired: 2 in, 2 out]
              }
            }
            n1351 = property on="Reading LeCroy2 Page" class="Bool (strict)"(error in=w2974, "Value"=FALSE ("Reading LeCroy2 Page")) -> (error out=w2973:errorcluster)  [unwired: 1 in, 1 out]
          }
          event "stop": Value Change {
            n1352 = event-data() -> ("NewVal"=w3066:bool)  [unwired: 1 in, 5 out]
          }
        }
      }
    }
    frame Error {
    }
  }
  n1353 = case shown="No Error" w7 {
    tunnel: [w3067 _] -> w15
    tunnel: w11 -> [_ _]
    frame No Error {
      n1354 = while {
        tunnel: [w3068] -> w3067
        stop <- w3069 stop-if-true
        n1355 = event shown="[0] \"Do Caen Page Read\": Value Change" {
          selector: _ -> [_ _]
          dyn-events: _ -> [_ _]
          timeout: _ -> [_ _]
          tunnel: [_ w3173] -> w3069
          tunnel: [w3076 _] -> w3068
          event "Do Caen Page Read": Value Change {
            w3071 = 0  # Crate
            w3073 = TRUE ("Visible")
            # "TODO: add error\nhandling for vi\nthat generates\nplot images"
            n1356 = event-data() -> ()  [unwired: 1 in, 1 out]
            n1357 = property on="Reading page" class="Str"("Visible"=w3073) -> (error out=w3074:errorcluster)  [unwired: 2 in, 1 out]
            n1358 = property on="Reading page" class="Bool (strict)"(error in=w3074, "Value"=w3073) -> (error out=w3072:errorcluster)  [unwired: 1 in, 1 out]
            n1359 = for {
              N: 3 -> [_]
              tunnel: [w3091] -> w3070
              tunnel: "Do Caen Page Read" -> [w3086]
              tunnel: [w3086] -> w3079
              tunnel: [FALSE ("Visible")] -> w3075
              tunnel: w3072 -> [w3094]
              tunnel: w3071 -> [w3093]
              stop <- w3098 continue-if-true
              n1360 = local read "Kill All"() -> (w3100:bool)
              n1361 = local read "stop"() -> (w3099:bool)
              n1362 = call "read channel page caen.vi"("Crate"=w3093, "page"=w3086, "error in"=w3094) -> ("VISA out"=w3101:refnum<visa-resource-name>, "New Channels"=w3095:T8[], "Start Index in ACTIVE"=w3088:i32, "error out"=w3097:errorcluster)  [unwired: 8 in, 1 out]
              n1363 = Compound Arithmetic op=AND(invert w3100, invert w3099, w3097) -> (w3098:bool)
              n1364 = case shown="No Error" w3097 {
                selector: w3097 -> [_ w3159]
                tunnel: [w3122 w3158] -> w3111
                tunnel: [w3121 _] -> w3110
                tunnel: [w3120 _] -> w3109
                tunnel: [w3119 _] -> w3108
                tunnel: [w3118 _] -> w3107
                tunnel: "Log to File" -> [w3117 _]
                tunnel: [w3116 _] -> w3105
                tunnel: [w3115 _] -> w3104
                tunnel: [w3114 _] -> w3103
                tunnel: w3095 -> [w3113 _]
                tunnel: [w3112 _] -> w3102
                tunnel: w3101 -> [_ w3153]
                frame No Error {
                  n1365 = for {
                    tunnel: w3113 -> [w3126] mode=indexing
                    tunnel: [w3144] -> w3122 mode=indexing
                    tunnel: [w3134] -> w3121 mode=indexing
                    tunnel: [w3142] -> w3120 mode=indexing
                    tunnel: [w3141] -> w3119 mode=indexing
                    tunnel: [w3140] -> w3118 mode=indexing
                    tunnel: w3117 -> [w3139]
                    tunnel: [w3136] -> w3116 mode=indexing
                    tunnel: ["History Length"] -> w3114
                    tunnel: [w3133] -> w3115 mode=indexing
                    tunnel: [TRUE ("append to file? (F)")] -> w3112
                    n1366 = Unbundle By Name(w3126) -> ("Timestamp"=w3138:string, "Vmon (V)"=w3134:dbl, "Vset (V)"=w3142:dbl, "Imon (A)"=w3141:dbl, "Iset (A)"=w3140:dbl, "Crate"=w3132:i32, "Card"=w3131:i32, "Channel"=w3130:i32)
                    n1367 = local read "Current Channel Log"() -> (w3128:path)
                    n1368 = Format Into String(format string="Monitoring_Log_%d-%d-%d.csv" ("string"), w3132, w3131, w3130) -> (resulting string=w3129:string, error out=w3123:errorcluster)  [unwired: 2 in]
                    n1369 = call "channel cluster to array.vi"("input cluster"=w3126) -> ("Array"=w3143:string[])  [unwired: 10 in]
                    n1370 = call-poly "Timestamp String to LV Timestamp Poly.vi"("Timestamp String"=w3138) -> ("Y M D H M S Array"=w3133:i32[], "Timestamp"=w3137:timestamp)
                    n1371 = Build Path(base path=w3128, name or relative path=w3129) -> (appended path=w3145:path)
                    n1372 = To Double Precision Float(number=w3137) -> (double precision float=w3136:dbl)
                    n1373 = case shown="True" w3139 {
                      tunnel: w3145 -> [_ w3151]
                      tunnel: [_ w3150] -> w3144
                      tunnel: w3143 -> [_ w3149]
                      tunnel: w3123 -> [_ w3147]
                      tunnel: TRUE ("append to file? (F)") -> [_ w3146]
                      frame False {
                      }
                      frame True {
                        n1374 = call-poly <vilib>:"Write Delimited Spreadsheet.vi"("file path (dialog if empty)"=w3151, "1D data"=w3149, "append to file? (new file:F)"=w3146, "error in (no error)"=w3147, "delimiter (\\t)"="," ("delimiter (\\t)")) -> ("error out"=w3150:errorcluster)  [unwired: 9 in, 1 out]
                      }
                    }
                  }
                }
                frame Error {
                  n1375 = VISA Write(VISA resource name=w3153, write buffer="\nQ") -> (VISA resource name out=w3155:refnum<visa-resource-name>, error out=w3156:errorcluster)  [unwired: 1 in, 1 out]
                  n1376 = call "read caen.vi"("VISA in"=w3155, "Extended Delay"=TRUE, "error in"=w3156) -> ("error out"=w3152:errorcluster)  [unwired: 7 in, 5 out]
                  n1377 = Build Array(w3159, w3152) -> (w3158:errorcluster[])
                }
              }
              n1378 = case shown="True" w3102 {
                tunnel: w3110 -> [_ w3166]
                tunnel: w3109 -> [_ w3167]
                tunnel: w3108 -> [_ w3168]
                tunnel: w3107 -> [_ w3169]
                tunnel: w3105 -> [_ w3165]
                tunnel: w3104 -> [_ w3172]
                tunnel: w3103 -> [_ w3171]
                tunnel: w3088 -> [_ w3170]
                frame False {
                }
                frame True {
                  w3160 = history_array_type."Iset" ("Log")
                  w3161 = history_array_type."Imon" ("Log")
                  w3162 = history_array_type."Vset" ("Log")
                  w3163 = history_array_type."Vmon" ("Log")
                  w3164 = history_array_type."TimeStamp" ("Log")
                  n1379 = call-poly "buffer array poly.vi"("Array"=w3172, "History length"=w3171, "Start channel"=w3170) -> ()  [unwired: 17 in]
                  n1380 = call "buffer array 1D.vi"("Array"=w3165, "History length"=w3171, "Log"=w3164, "Start channel"=w3170) -> ()  [unwired: 16 in]
                  n1381 = call "buffer array 1D.vi"("Array"=w3166, "History length"=w3171, "Log"=w3163, "Start channel"=w3170) -> ()  [unwired: 16 in]
                  n1382 = call "buffer array 1D.vi"("Array"=w3167, "History length"=w3171, "Log"=w3162, "Start channel"=w3170) -> ()  [unwired: 16 in]
                  n1383 = call "buffer array 1D.vi"("Array"=w3168, "History length"=w3171, "Log"=w3161, "Start channel"=w3170) -> ()  [unwired: 16 in]
                  n1384 = call "buffer array 1D.vi"("Array"=w3169, "History length"=w3171, "Log"=w3160, "Start channel"=w3170) -> ()  [unwired: 16 in]
                  n1385 = call-poly "buffer array poly.vi"("Array"=w3165, "History length"=w3171, "Log"=w3164, "Start channel"=w3170) -> ()  [unwired: 16 in]
                  n1386 = call-poly "buffer array poly.vi"("Array"=w3166, "History length"=w3171, "Log"=w3163, "Start channel"=w3170) -> ()  [unwired: 16 in]
                  n1387 = call-poly "buffer array poly.vi"("Array"=w3167, "History length"=w3171, "Log"=w3162, "Start channel"=w3170) -> ()  [unwired: 16 in]
                  n1388 = call-poly "buffer array poly.vi"("Array"=w3168, "History length"=w3171, "Log"=w3161, "Start channel"=w3170) -> ()  [unwired: 16 in]
                  n1389 = call-poly "buffer array poly.vi"("Array"=w3169, "History length"=w3171, "Log"=w3160, "Start channel"=w3170) -> ()  [unwired: 16 in]
                }
              }
              n1390 = Merge Errors(w3111) -> (w3092:errorcluster)
              n1391 = Array Size(array=w3095) -> (size(s)=w3087:i32)
              n1392 = Bundle(cluster=T2 {"Start Index"=0, "Num Channels Read"=0} ("Value (Signaling)"), "Start Index"=w3088, "Num Channels Read"=w3087) -> (w3089:T2)
              n1393 = property on="Update Plots & Alarms" class="Clust (strict)"(error in=w3092, "Val(Sgnl)"=w3089) -> (error out=w3091:errorcluster)  [unwired: 1 in, 1 out]
            }
            n1394 = property on="Reading page" class="Str"("Visible"=w3075) -> (error out=w3077:errorcluster)  [unwired: 2 in, 1 out]
            n1395 = case shown="Error" w3070 {
              selector: w3070 -> [_ w3081]
              tunnel: w3071 -> [_ w3083]
              frame No Error {
              }
              frame Error {
                n1396 = Bundle("Crate"=w3083, "error IO"=w3081) -> (w3082:cluster{"Crate":i32, "error IO":errorcluster})  [unwired: 1 in]
                n1397 = property on="read error" class="Clust (strict)"("Val(Sgnl)"=w3082) -> ()  [unwired: 2 in, 2 out]
              }
            }
            n1398 = case shown="0" w3079 {
              tunnel: w3070 -> [_ w3085]
              tunnel: [_ w3084] -> _
              frame Default {
              }
              frame 0 {
                n1399 = call "picture plot.vi"("error in"=w3085) -> ("error out"=w3084:errorcluster)  [unwired: 9 in, 1 out]
              }
            }
            n1400 = property on="Reading page" class="Bool (strict)"(error in=w3077, "Value"=w3075) -> (error out=w3076:errorcluster)  [unwired: 1 in, 1 out]
          }
          event "stop": Value Change {
            n1401 = event-data() -> ("NewVal"=w3173:bool)  [unwired: 1 in, 5 out]
          }
        }
      }
    }
    frame Error {
    }
  }
  n1402 = case shown="No Error" w7 {
    tunnel: [w3174 _] -> w13
    frame No Error {
      n1403 = while {
        tunnel: [w3175] -> w3174
        stop <- w3176 stop-if-true
        n1404 = event shown="[0] \"Do L1 Page Read\": Value Change" {
          selector: _ -> [_ _]
          dyn-events: _ -> [_ _]
          timeout: _ -> [_ _]
          tunnel: [_ w3273] -> w3176
          tunnel: [w3177 _] -> w3175
          tunnel: [w3181 _] -> _
          event "Do L1 Page Read": Value Change {
            w3178 = 1  # Crate
            n1405 = event-data() -> ()  [unwired: 1 in, 1 out]
            n1406 = property on="Reading LeCroy1 Page" class="Bool (strict)"("Value"=TRUE ("Reading LeCroy1 Page")) -> (error out=w3179:errorcluster)  [unwired: 2 in, 1 out]
            n1407 = for {
              N: 3 -> [_]
              tunnel: [w3190] -> w3177
              tunnel: "Do L1 Page Read" -> [w3205]
              tunnel: w3179 -> [w3199]
              tunnel: w3178 -> [w3198]
              tunnel: [w3189] -> w3180
              stop <- w3201 continue-if-true
              n1408 = local read "Kill All"() -> (w3203:bool)
              n1409 = local read "Log to File"() -> (w3197:bool)
              n1410 = local read "stop"() -> (w3202:bool)
              n1411 = call "read channel page lecroy.vi"("Crate"=w3198, "page"=w3205, "error in"=w3199) -> ("VISA out"=w3204:refnum<visa-resource-name>, "New Channels"=w3193:T8[], "Start Index in ACTIVE"=w3191:i32, "error out"=w3200:errorcluster)  [unwired: 8 in, 1 out]
              n1412 = Compound Arithmetic op=AND(invert w3203, invert w3202, w3200) -> (w3201:bool)
              n1413 = case shown="No Error" w3200 {
                selector: w3200 -> [_ w3259]
                tunnel: [w3225 w3258] -> w3214
                tunnel: [w3224 _] -> w3213
                tunnel: [w3223 _] -> w3212
                tunnel: [w3222 _] -> w3211
                tunnel: [w3221 _] -> w3210
                tunnel: w3197 -> [w3220 _]
                tunnel: [w3219 _] -> w3209
                tunnel: [w3218 _] -> w3208
                tunnel: [w3217 _] -> w3207
                tunnel: w3193 -> [w3216 _]
                tunnel: [w3215 _] -> w3206
                tunnel: w3204 -> [_ w3257]
                frame No Error {
                  n1414 = for {
                    tunnel: w3216 -> [w3230] mode=indexing
                    tunnel: [w3247] -> w3225 mode=indexing
                    tunnel: [w3238] -> w3224 mode=indexing
                    tunnel: [w3245] -> w3223 mode=indexing
                    tunnel: [w3244] -> w3222 mode=indexing
                    tunnel: [w3243] -> w3221 mode=indexing
                    tunnel: w3220 -> [w3242]
                    tunnel: [w3239] -> w3219 mode=indexing
                    tunnel: [w3226] -> w3217
                    tunnel: [w3237] -> w3218 mode=indexing
                    tunnel: [TRUE ("append to file? (F)")] -> w3215
                    n1415 = Unbundle By Name(w3230) -> ("Timestamp"=w3241:string, "Vmon (V)"=w3238:dbl, "Vset (V)"=w3245:dbl, "Imon (A)"=w3244:dbl, "Iset (A)"=w3243:dbl, "Crate"=w3236:i32, "Card"=w3235:i32, "Channel"=w3234:i32)
                    n1416 = local read "Current Channel Log"() -> (w3232:path)
                    n1417 = Format Into String(format string="Monitoring_Log_%d-%d-%d.csv" ("string"), w3236, w3235, w3234) -> (resulting string=w3233:string, error out=w3227:errorcluster)  [unwired: 2 in]
                    n1418 = call "channel cluster to array.vi"("input cluster"=w3230) -> ("Array"=w3246:string[])  [unwired: 10 in]
                    n1419 = call-poly "Timestamp String to LV Timestamp Poly.vi"("Timestamp String"=w3241) -> ("Y M D H M S Array"=w3237:i32[], "Timestamp"=w3240:timestamp)
                    n1420 = Build Path(base path=w3232, name or relative path=w3233) -> (appended path=w3248:path)
                    n1421 = To Double Precision Float(number=w3240) -> (double precision float=w3239:dbl)
                    n1422 = local read "History Length"() -> (w3226:i32)
                    n1423 = case shown="True" w3242 {
                      tunnel: w3248 -> [_ w3254]
                      tunnel: [_ w3253] -> w3247
                      tunnel: w3246 -> [_ w3252]
                      tunnel: w3227 -> [_ w3250]
                      tunnel: TRUE ("append to file? (F)") -> [_ w3249]
                      frame False {
                      }
                      frame True {
                        n1424 = call-poly <vilib>:"Write Delimited Spreadsheet.vi"("file path (dialog if empty)"=w3254, "1D data"=w3252, "append to file? (new file:F)"=w3249, "error in (no error)"=w3250, "delimiter (\\t)"="," ("delimiter (\\t)")) -> ("error out"=w3253:errorcluster)  [unwired: 9 in, 1 out]
                      }
                    }
                  }
                }
                frame Error {
                  n1425 = VISA Flush I/O Buffer(VISA resource name=w3257) -> (error out=w3256:errorcluster)  [unwired: 2 in, 1 out]
                  n1426 = Wait (ms)(milliseconds to wait=u32 1000) -> ()  [unwired: 1 out]
                  n1427 = Build Array(w3259, w3256) -> (w3258:errorcluster[])
                }
              }
              n1428 = case shown="True" w3206 {
                tunnel: w3213 -> [_ w3266]
                tunnel: w3212 -> [_ w3267]
                tunnel: w3211 -> [_ w3268]
                tunnel: w3210 -> [_ w3269]
                tunnel: w3209 -> [_ w3265]
                tunnel: w3208 -> [_ w3272]
                tunnel: w3207 -> [_ w3271]
                tunnel: w3191 -> [_ w3270]
                frame False {
                }
                frame True {
                  w3260 = history_array_type."Iset" ("Log")
                  w3261 = history_array_type."Imon" ("Log")
                  w3262 = history_array_type."Vset" ("Log")
                  w3263 = history_array_type."Vmon" ("Log")
                  w3264 = history_array_type."TimeStamp" ("Log")
                  n1429 = call-poly "buffer array poly.vi"("Array"=w3272, "History length"=w3271, "Start channel"=w3270) -> ()  [unwired: 17 in]
                  n1430 = call "buffer array 1D.vi"("Array"=w3265, "History length"=w3271, "Log"=w3264, "Start channel"=w3270) -> ()  [unwired: 16 in]
                  n1431 = call "buffer array 1D.vi"("Array"=w3266, "History length"=w3271, "Log"=w3263, "Start channel"=w3270) -> ()  [unwired: 16 in]
                  n1432 = call "buffer array 1D.vi"("Array"=w3267, "History length"=w3271, "Log"=w3262, "Start channel"=w3270) -> ()  [unwired: 16 in]
                  n1433 = call "buffer array 1D.vi"("Array"=w3268, "History length"=w3271, "Log"=w3261, "Start channel"=w3270) -> ()  [unwired: 16 in]
                  n1434 = call "buffer array 1D.vi"("Array"=w3269, "History length"=w3271, "Log"=w3260, "Start channel"=w3270) -> ()  [unwired: 16 in]
                  n1435 = call-poly "buffer array poly.vi"("Array"=w3265, "History length"=w3271, "Log"=w3264, "Start channel"=w3270) -> ()  [unwired: 16 in]
                  n1436 = call-poly "buffer array poly.vi"("Array"=w3266, "History length"=w3271, "Log"=w3263, "Start channel"=w3270) -> ()  [unwired: 16 in]
                  n1437 = call-poly "buffer array poly.vi"("Array"=w3267, "History length"=w3271, "Log"=w3262, "Start channel"=w3270) -> ()  [unwired: 16 in]
                  n1438 = call-poly "buffer array poly.vi"("Array"=w3268, "History length"=w3271, "Log"=w3261, "Start channel"=w3270) -> ()  [unwired: 16 in]
                  n1439 = call-poly "buffer array poly.vi"("Array"=w3269, "History length"=w3271, "Log"=w3260, "Start channel"=w3270) -> ()  [unwired: 16 in]
                }
              }
              n1440 = Merge Errors(w3214) -> (w3192:errorcluster)
              n1441 = Array Size(array=w3193) -> (size(s)=w3196:i32)
              n1442 = Bundle(cluster=T2 {"Start Index"=0, "Num Channels Read"=0} ("Value (Signaling)"), "Start Index"=w3191, "Num Channels Read"=w3196) -> (w3195:T2)
              n1443 = property on="Update Plots & Alarms" class="Clust (strict)"(error in=w3192, "Val(Sgnl)"=w3195) -> (error out=w3190:errorcluster)  [unwired: 1 in, 1 out]
              n1444 = call <vilib>:"Clear Errors.vi"("error in (no error)"=w3190) -> ("error out"=w3189:errorcluster)  [unwired: 5 in, 1 out]
            }
            n1445 = case shown="Error" w3177 {
              selector: w3177 -> [_ w3186]
              tunnel: w3178 -> [_ w3187]
              frame No Error {
              }
              frame Error {
                n1446 = Bundle("Crate"=w3187, "error IO"=w3186) -> (w3188:cluster{"Crate":i32, "error IO":errorcluster})  [unwired: 1 in]
                n1447 = property on="read error" class="Clust (strict)"("Val(Sgnl)"=w3188) -> ()  [unwired: 2 in, 2 out]
              }
            }
            n1448 = property on="Reading LeCroy1 Page" class="Bool (strict)"(error in=w3180, "Value"=FALSE ("Reading LeCroy1 Page")) -> (error out=w3181:errorcluster)  [unwired: 1 in, 1 out]
          }
          event "stop": Value Change {
            n1449 = event-data() -> ("NewVal"=w3273:bool)  [unwired: 1 in, 5 out]
          }
        }
      }
    }
    frame Error {
    }
  }
  n1450 = control-ref of="stop"() -> (w4:refnum<vi>)
  n1451 = case shown="No Error" w7 {
    frame No Error {
      n1452 = while {
        stop <- w3275 stop-if-true
        n1453 = event shown="[0] Timeout" {
          selector: _ -> [_ _]
          dyn-events: _ -> [_ _]
          timeout: 5 -> [_ _]
          tunnel: [_ w3339] -> w3275
          event Timeout {
            # "192.168.163.5\n annielx02"
            n1454 = event-data() -> ()  [unwired: 1 in, 1 out]
            n1455 = call <vilib>:"TCP Listen.vi"("timeout ms (wait forever: -1)"=1000 ("timeout ms (60000)"), "port"="Slack port") -> ("error out"=w3277:errorcluster, "connection ID"=w3280:refnum<k5>)  [unwired: 5 in, 3 out]
            n1456 = case shown="No Error" w3277 {
              selector: w3277 -> [w3287 w3331]
              tunnel: w3280 -> [w3290 _]
              tunnel: 56 ("specific error code to clear (0: all)") -> [_ w3330]
              frame No Error {
                n1457 = local read "slack"() -> (w3289:T1)
                n1458 = call <vilib>:"Acquire Semaphore.vi"("error in (no error)"=w3287, "ms timeout (-1)"=1000 ("timeout ms (60000)"), "semaphore"=w3289) -> ("error out"=w3284:errorcluster, "timed out"=w3285:bool, "semaphore out"=w3283:T1)  [unwired: 2 in]
                n1459 = Or(x=w3285, y=w3284) -> (x .or. y?=w3286:bool)
                n1460 = case shown="False" w3286 {
                  tunnel: w3290 -> [w3301 _]
                  tunnel: w3284 -> [w3298 w3325]
                  tunnel: [_ w3326] -> _
                  tunnel: w3283 -> [w3294 _]
                  frame False {
                    w3295 = T30 0 items=["no dialog", "OK message", "continue or stop message", "OK message + warnings", "continue/stop + warnings"] ("type of dialog (OK msg:1)")
                    n1461 = case shown="Default" "New Errors" {
                      selector: "New Errors" -> [_ w3316]
                      tunnel: w3301 -> [w3315 w3320]
                      tunnel: [w3315 w3319] -> w3300
                      tunnel: [w3314 w3318] -> w3299
                      tunnel: w3298 -> [w3314 w3317]
                      frame "" {
                      }
                      frame Default {
                        n1462 = TCP Write(connection ID=w3320, data in=w3316, error in (no error)=w3317) -> (connection ID out=w3319:refnum<k5>, error out=w3318:errorcluster)  [unwired: 2 out]
                      }
                    }
                    n1463 = TCP Close Connection(connection ID=w3300, error in (no error)=w3299) -> (error out=w3296:errorcluster)  [unwired: 1 in, 1 out]
                    n1464 = case shown="No Error" w3296 {
                      selector: w3296 -> [_ w3311]
                      tunnel: "Error transmitting errors to annielx01! Error was: %s" ("string") -> [_ w3312]
                      tunnel: w3295 -> [_ w3310]
                      tunnel: [_ w3308] -> _
                      tunnel: [_ w3307] -> _
                      tunnel: [_ w3306] -> _
                      frame No Error {
                      }
                      frame Error {
                        n1465 = call <vilib>:"Simple Error Handler.vi"("type of dialog (OK msg:1)"=w3310, "error in (no error)"=w3311) -> ("error out"=w3308:errorcluster, "message"=w3309:string)  [unwired: 3 in, 3 out]
                        n1466 = Format Into String(format string=w3312, w3309) -> (resulting string=w3313:string, error out=w3307:errorcluster)  [unwired: 2 in]
                        n1467 = property on="slack error" class="Str"("Val(Sgnl)"=w3313) -> (error out=w3306:errorcluster)  [unwired: 2 in, 1 out]
                      }
                    }
                    n1468 = flat-sequence {
                      tunnel: "New Errors" -> [_]
                      tunnel: w3294 -> [w3303]
                      tunnel: [w3303] -> w3292
                      tunnel: "" -> [w3302]
                      tunnel: [w3304] -> _
                      tunnel: w3292 -> [w3305]
                      frame #0 {
                        n1469 = local write "New Errors"(w3302) -> ()
                      }
                      frame #1 {
                        n1470 = call <vilib>:"Release Semaphore.vi"("semaphore"=w3305) -> ("error out"=w3304:errorcluster)  [unwired: 5 in, 1 out]
                      }
                    }
                  }
                  frame True {
                    w3327 = T30 0 items=["no dialog", "OK message", "continue or stop message", "OK message + warnings", "continue/stop + warnings"] ("type of dialog (OK msg:1)")
                    n1471 = call <vilib>:"Simple Error Handler.vi"("type of dialog (OK msg:1)"=w3327, "error in (no error)"=w3325) -> ("error out"=w3324:errorcluster, "message"=w3323:string)  [unwired: 3 in, 3 out]
                    n1472 = Select(t=w3323, s=w3324, f="Timed out obtaining semaphore for reading new messages from slack buffer!\nErrors will NOT be sent to slack!!" ("source")) -> (s? t:f=w3321:string)
                    n1473 = property on="slack error" class="Str"("Val(Sgnl)"=w3321) -> (error out=w3326:errorcluster)  [unwired: 2 in, 1 out]
                  }
                }
                n1474 = call "Append to display log.vi"("string"="Reporting new errors to Slack") -> ("error out"=w3282:errorcluster)  [unwired: 10 in]
                n1475 = call <vilib>:"Clear Errors.vi"("error in (no error)"=w3282) -> ()  [unwired: 5 in, 2 out]
              }
              frame Error {
                n1476 = call <vilib>:"Clear Errors.vi"("error in (no error)"=w3331, "specific error code to clear (0: all)"=w3330) -> ("error out"=w3329:errorcluster)  [unwired: 4 in, 1 out]
                n1477 = case shown="No Error" w3329 {
                  selector: w3329 -> [_ w3337]
                  tunnel: "Error listening to TCP port %d for reporting errors to slack! Error was: %s" ("string") -> [_ w3338]
                  tunnel: [_ w3332] -> _
                  frame No Error {
                    # "timeout error - expected\nwhen no poll request\nreceived from annielx01"
                  }
                  frame Error {
                    # "Something else is wrong with slack\nerror reporting network connection!"
                    n1478 = Unbundle(w3337) -> ("code"=w3336:i32, "source"=w3335:string)  [unwired: 1 out]
                    n1479 = Format Into String(format string=w3338, w3336, w3335) -> (resulting string=w3334:string, error out=w3333:errorcluster)  [unwired: 2 in]
                    n1480 = property on="slack error" class="Str"(error in=w3333, "Val(Sgnl)"=w3334) -> (error out=w3332:errorcluster)  [unwired: 1 in, 1 out]
                  }
                }
              }
            }
          }
          event "stop": Value Change {
            n1481 = event-data() -> ("NewVal"=w3339:bool)  [unwired: 1 in]
          }
        }
      }
    }
    frame Error {
    }
  }
  n1482 = control-ref of="Current ZMQ Log"() -> (w3:refnum<vi>)
  n1483 = disable-structure shown="Disabled" {
    disable-tunnel: [w3340 _] -> _
    frame Disabled {
      # "standalone exe that connects to the ZMQ and reads any outstanding writes. \nIndended to stop the ZMQ write hanging by reading messages that weren't picked up within a time limit.\nBut we can't do this! ZMQ Dealer sends messages on a ROUND ROBIN TO ALL CONNECTED LISTENERS.\nIf we set up another context to listen, it will receive half the messages, preventing them getting to the DAQ!"
      n1484 = local read "ZMQ endpoint"() -> (w3343:string)
      n1485 = xnode "Match Regular Expression"("input string"=w3343, "regular expression"="[0-9]+$") -> ("before match"=w3345:string, "error out"=w3341:errorcluster)  [unwired: 4 in, 3 out]
      n1486 = Concatenate Strings("\"C:\\Users\\ANNIE\\Documents\\CAEN_SY527 v3\\builds\\standalone ZMQ\\flush_ZMQ_standalone\\flush_ZMQ_standalone.exe\" " ("command line"), w3345) -> (w3344:string)
      n1487 = case shown="No Error" w3341 {
        selector: w3341 -> [_ w3383]
        tunnel: [w3352 w3383] -> w3340
        tunnel: [w3348 _] -> _
        tunnel: w3344 -> [w3347 _]
        frame No Error {
          n1488 = node-c288(0 ("Processor")) -> (w3351:T32)
          n1489 = timed-loop {
            tunnel: [w3354] -> w3352
            timing: w3351 -> [_]
            timing-out: [_] -> w3350
            tunnel: w3347 -> [w3353]
            stop <- w3355 stop-if-true
            n1490 = event shown="[0] \"Sending ZMQ\": Value Change" {
              selector: _ -> [_ _]
              dyn-events: _ -> [_ _]
              timeout: _ -> [_ _]
              tunnel: [w3359 _] -> w3356
              tunnel: [w3360 _] -> w3354
              tunnel: [w3359 w3375] -> w3355
              tunnel: w3353 -> [w3357 _]
              event "Sending ZMQ": Value Change {
                n1491 = event-data() -> ("NewVal"=w3358:bool, "Time"=w3361:u32)  [unwired: 1 in]
                n1492 = case shown="True" w3358 {
                  tunnel: w3361 -> [_ w3368]
                  tunnel: [_ w3363] -> w3360
                  tunnel: [_ w3364] -> w3359
                  tunnel: w3357 -> [_ w3365]
                  frame False {
                  }
                  frame True {
                    n1493 = while {
                      tunnel: w3368 -> [w3373]
                      tunnel: [w3370] -> w3364
                      stop <- w3370 continue-if-true
                      n1494 = Tick Count (ms)() -> (millisecond timer value=w3374:u32)
                      n1495 = Subtract(x=w3374, y=w3373) -> (x-y=w3372:u32)
                      n1496 = Wait (ms)(milliseconds to wait=u32 1000 ("y")) -> ()  [unwired: 1 out]
                      n1497 = Less Or Equal?(x=w3372, y=u32 10000) -> (x <= y?=w3370:bool)
                    }
                    n1498 = call <vilib>:"System Exec.vi"("run minimized? (F)"=w3364, "command line"=w3365) -> ("error out"=w3363:errorcluster, "standard output"=w3362:string)  [unwired: 6 in, 2 out]
                    n1499 = Build Array (concatenate)("Unsent Messages", w3362) -> (w3366:string[])
                    n1500 = local write "Unsent Messages"(w3366) -> ()
                  }
                }
              }
              event "stop": Value Change {
                n1501 = event-data() -> ("NewVal"=w3375:bool)  [unwired: 1 in]
              }
            }
            "Sending ZMQ" <- w3356
          }
          n1502 = node-c288(w3350) -> (w3348:errorcluster)
        }
        frame Error {
        }
      }
    }
    frame Enabled {
    }
  }
  n1503 = call "ZMQ queue reads.vi"("context in"=w9, "Current ZMQ Log"=w3, "zmq_socket in"=w19, "queue in"=w37, "Stop"=w4, "Error in"=w2) -> ("ZMQ error out"=w28:errorcluster, "Queue error out"=w26:errorcluster)  [unwired: 7 in, 1 out]
  n1504 = disable-structure shown="Enabled" {
    disable-tunnel: w2 -> [w3499 w3513 _]
    disable-tunnel: [w3498 w3512 _] -> w1
    frame Disabled {
      n1505 = case shown="No Error" w3499 {
        selector: w3499 -> [_ w3511]
        tunnel: [_ w3511] -> w3498
        frame No Error {
          n1506 = while {
            stop <- w3502 stop-if-true
            w3500 = u32 600000 ("timeout ms (-1 never timeout)")
            n1507 = To Long Integer(number=w3500) -> (32bit integer=w3501:i32)
            n1508 = Tick Count (ms)() -> (millisecond timer value=w3505:u32)
            n1509 = Wait For Front Panel Activity(1:w3501) -> (0:w3506:u32)  [unwired: 2 in]
            n1510 = Compound Arithmetic op=ADD(invert w3505, w3506) -> (w3503:u32)
            n1511 = Greater Or Equal?(x=w3503, y=w3500) -> (x >= y?=w3504:bool)
            n1512 = case shown="True" w3504 {
              tunnel: [w3507 w3508] -> w3502
              frame False {
                n1513 = local read "stop"() -> (w3507:bool)
              }
              frame True {
                # "No UI activity for 10\",\nmake sure lock and scan\nare reset"
                n1514 = local write "Lock Page"(FALSE ("Lock Page")) -> ()
                n1515 = local read "stop"() -> (w3508:bool)
                n1516 = local write "scan"(TRUE ("Lock Page")) -> ()
              }
            }
          }
        }
        frame Error {
        }
      }
    }
    frame Disabled {
      n1517 = case shown="No Error" w3513 {
        selector: w3513 -> [_ w3524]
        tunnel: [_ w3524] -> w3512
        frame No Error {
          n1518 = while {
            stop <- w3514 stop-if-true
            n1519 = event shown="[0] Timeout" {
              selector: _ -> [_ _]
              dyn-events: _ -> [_ _]
              timeout: 500 -> [_ _]
              tunnel: [_ w3523] -> w3514
              event Timeout {
                w3516 = u32 600000 ("timeout ms (-1 never timeout)")
                n1520 = event-data() -> ()  [unwired: 1 in, 1 out]
                n1521 = Tick Count (ms)() -> (millisecond timer value=w3519:u32)
                n1522 = Wait For Front Panel Activity(1:w3516) -> (0:w3520:u32)  [unwired: 2 in]
                n1523 = Compound Arithmetic op=ADD(invert w3519, w3520) -> (w3517:u32)
                n1524 = Greater Or Equal?(x=w3517, y=w3516) -> (x >= y?=w3518:bool)
                n1525 = case shown="True" w3518 {
                  frame False {
                  }
                  frame True {
                    # "No UI activity for 10\",\nmake sure lock and scan\nare reset"
                    n1526 = local write "Lock Page"(FALSE ("Lock Page")) -> ()
                    n1527 = local write "scan"(TRUE ("Lock Page")) -> ()
                  }
                }
              }
              event "stop": Value Change {
                n1528 = event-data() -> ("NewVal"=w3523:bool)  [unwired: 1 in]
              }
            }
          }
        }
        frame Error {
        }
      }
    }
    frame Enabled {
    }
  }
  n1529 = Release Queue(queue=w35) -> (error out=w34:errorcluster)  [unwired: 2 in, 2 out]
  n1530 = VISA Close(VISA resource name=w33, error in (no error)=w32) -> (error out=w31:errorcluster)
  n1531 = Unregister For Events(event registration refnum=w55) -> (error out=w36:errorcluster)  [unwired: 1 in]
  n1532 = Destroy User Event(user event=w29, error in=w28) -> (error out=w27:errorcluster)
  n1533 = Get Date/Time String(want seconds? (F)=w18) -> (date string=w50:string, time string=w51:string)  [unwired: 2 in]
  n1534 = call <vilib>:"Release Semaphore Reference.vi"("semaphore"=w6) -> ("error out"=w5:errorcluster)  [unwired: 9 in, 1 out]
  n1535 = call <vilib>:"Space Constant.vi"() -> ("String"=w52:string)
  n1536 = Merge Errors(w15, w13, w12) -> (w14:errorcluster)
  n1537 = Concatenate Strings(w50, w52, w51) -> (w53:string)
  n1538 = Concatenate Strings("Program stopped at " ("string"), w53) -> (w42:string)
  n1539 = Merge Errors(w34, w36, w27, w31, w26, w1, w14, w5) -> (w30:errorcluster)
  n1540 = call "Append to display log.vi"("string"=w42) -> ("error out"=w41:errorcluster)  [unwired: 10 in]
  n1541 = local write "error out"(w30) -> ()
  n1542 = call <vilib>:"Clear Errors.vi"("error in (no error)"=w41) -> ("error out"=w43:errorcluster)  [unwired: 5 in, 1 out]
  n1543 = call "Append to event log.vi"("error in"=w43, "string"="Program stopped ") -> ("error out"=w44:errorcluster)  [unwired: 9 in]
  n1544 = call <vilib>:"Clear Errors.vi"("error in (no error)"=w44) -> ()  [unwired: 5 in, 2 out]
